vi "squash2016_2.vi"() -> ()   [LabVIEW 2014]
uses:
  <vilib>/vision/Image Controls.llb/IMAQ Image.ctl
  <vilib>/Utility/file.llb/Read From Spreadsheet File (string).vi
  <vilib>/Utility/file.llb/Read From Spreadsheet File (I64).vi
panel:
  in  "Upload edited video":bool
  in  "Extract data":bool
  in  "UNex win1":string="Unexpected \nwinner"
  in  "Expected Winner1 4":bool
  in  "Player 1 shots":string[](array[string])=["Att drive", "Def drive", "Att SW drive", "Def SW drive", "", "Drop", "Chop", "Lob", "Boast 2", "Boast 3", "Smash", "", "F-hand", "B-hand", "", "Straight", "Cross", "", "Bounce", "Volley", "H-volley"]
  in  "Player 1 shots 2":string[](array[string])=["Att drive", "Def drive", "Att SW drive", "Def SW drive", "", "Drop", "Chop", "Lob", "Boast 2", "Boast 3", "Smash", "", "F-hand", "B-hand", "", "Straight", "Cross", "", "Bounce", "Volley", "H-volley"]
  in  "Player2 2":bool
  in  "Player1 2":bool
  in  "FH":bool
  in  "BH":bool
  in  "ST":bool
  in  "CR":bool
  in  "Bounce":bool
  in  "Half Volley":bool
  in  "Volley":bool
  out "last saved data":i64[](array[numeric])
  out "Btn 10":string
  out "Btn 9":string
  out "Btn 8":string
  out "Btn 7":string
  out "Btn 6":string
  out "subarray":i64[](array[numeric])
  out "output array":i64[][](array[numeric])
  out "appended array":i64[](array[numeric])
  out "0, 1":i16[](array[numeric])
  in  "REPORT":bool
  out "Player 2 data":i64[](array[numeric])
  out "player 1 data":i64[](array[numeric])
  out "both player data":i64[](array[numeric])
  out "Edited data":i64[][](array[numeric])
  out "Event After":i64[][](array[numeric])
  out "Event before":i64[][](array[numeric])
  out "result":i32[](array[numeric])
  out "EVENTS\nTO PLAY":i32[](array[numeric])
  out "Combined data":i64[][](array[numeric])
  out "Extra":i16
  out "Score change":bool[](array[boolean])
  out "last row":i32[](array[numeric])
  out "Player 1/2":i16
  out "Service":i16
  out "Cross":i16
  out "Straight":i16
  out "position":i16
  out "Main tab 2":T1(ring)
  in  "fast rewind":bool
  out "refnum of data save file":refnum<file>
  in  "START":bool
  out "frames to write":i64[][](array[numeric])
  in  "Data file":path=path "C:/Users/KoKuM/Desktop/Current work/ISN/SQUASH/testdata/test2.xls" caption="Data"
  in  "playback speed":dbl(slide)=1.0 min=0.25 max=1.5 step=0.25 scale=0.25..1.5
  in  "Main tab":enum32{"Coding", "Display"}(tab)
  in  "Boast 10":bool
  in  "Boast 12":bool
  in  "Boast 9":bool
  in  "Boast 11":bool
  in  "Smash 12":bool
  in  "Smash 11":bool
  in  "Smash 10":bool
  in  "Smash 9":bool
  in  "lob 12":bool
  in  "Drop 12":bool
  in  "lob 11":bool
  in  "Drop 11":bool
  in  "lob 10":bool
  in  "Drop 10":bool
  in  "lob 9":bool
  in  "Drop 9":bool
  in  "Chop 12":bool
  in  "Chop 11":bool
  in  "Chop 10":bool
  in  "Chop 9":bool
  in  "Smash 8":bool
  in  "Smash 7":bool
  in  "Smash 6":bool
  in  "Smash 5":bool
  in  "Smash":bool
  in  "Smash 2":bool
  in  "Smash 3":bool
  in  "Smash 4":bool
  in  "Chop 8":bool
  in  "Chop 7":bool
  in  "Chop 6":bool
  in  "Chop 5":bool
  in  "Chop":bool
  in  "Chop 2":bool
  in  "Chop 3":bool
  in  "Chop 4":bool
  in  "Boast 7":bool
  in  "Boast 5":bool
  in  "Boast 3":bool
  in  "Boast":bool
  in  "lob 8":bool
  in  "Drop 8":bool
  in  "Boast 6":bool
  in  "lob 7":bool
  in  "Drop 7":bool
  in  "lob 6":bool
  in  "Drop 6":bool
  in  "Boast 8":bool
  in  "lob 5":bool
  in  "Drop 5":bool
  in  "lob 13":bool
  in  "Drop":bool
  in  "Boast 2":bool
  in  "lob 2":bool
  in  "Drop 2":bool
  in  "lob 3":bool
  in  "Drop 3":bool
  in  "Boast 4":bool
  in  "lob 4":bool
  in  "Drop 4":bool
  in  "Let":bool
  in  "Nolet1":bool
  in  "Nolet2":bool
  in  "Stroke1":bool
  in  "Stroke2":bool
  in  "Expected Winner1":bool
  in  "Expected Winner2":bool
  in  "Unexpected Winner1":bool
  in  "Unexpected Winner2":bool
  in  "Forced Error1":bool
  in  "Unforced Error1":bool
  in  "Forced Error2":bool
  in  "Unforced Error2":bool
  in  "Pause lag(s)":dbl=1.0 min=0.0 max=2.0 step=0.5 format="%#.1g"
  in  "Code lag(s)":dbl=1.0 min=0.0 max=5.0 step=0.5 format="%#.1g"
  in  "Link Errors":bool
  in  "Btn 1":string
  in  "Btn 2":string
  in  "Btn 3":string
  in  "Btn 4":string
  in  "Btn 5":string
  in  "Button 1":bool
  in  "Button 2":bool
  in  "Button 3":bool
  in  "Button 4":bool
  in  "Button 5":bool
  out "P2":i32
  out "P1":i32
  out "Player1/Player2":bool[](array[boolean])
  in  "S6":bool
  in  "S5":bool
  in  "S4":bool
  in  "S3":bool
  in  "S2":bool
  in  "Service1":bool
  in  "Service2":bool
  in  "S1":bool
  in  "Player2":bool
  in  "Player1":bool
  in  "Auto switch":bool
  in  "5 4":bool
  in  "5 3":bool
  in  "5 2":bool
  in  "5 1":bool
  in  "6 4":bool
  in  "6 3":bool
  in  "6 2":bool
  in  "6 1":bool
  in  "4 4":bool
  in  "4 3":bool
  in  "4 2":bool
  in  "4 1":bool
  in  "3 4":bool
  in  "3 3":bool
  in  "3 2":bool
  in  "3 1":bool
  in  "2 4":bool
  in  "2 3":bool
  in  "2 2":bool
  in  "2 1":bool
  in  "1 4":bool
  in  "1 3":bool
  in  "1 2":bool
  in  "1 1":bool
  in  "after 2":u8(slide)=2 scale=0.0..5.0
  in  "before 2":u8(slide)=2
  in  "Pause lag on":bool
  in  "SWDrive":bool
  in  "SWADrive 12":bool
  in  "SWADrive 11":bool
  in  "SWADrive 10":bool
  in  "SWADrive 9":bool
  in  "SWDDrive 12":bool
  in  "SWDDrive 11":bool
  in  "SWDDrive 10":bool
  in  "SWDDrive 9":bool
  in  "ADrive 12":bool
  in  "ADrive 11":bool
  in  "ADrive 10":bool
  in  "ADrive 9":bool
  in  "DDrive 12":bool
  in  "DDrive 11":bool
  in  "DDrive 10":bool
  in  "DDrive 9":bool
  in  "DDrive 8":bool
  in  "DDrive 7":bool
  in  "DDrive 6":bool
  in  "DDrive 5":bool
  in  "DDrive":bool
  in  "DDrive 2":bool
  in  "DDrive 3":bool
  in  "DDrive 4":bool
  in  "ADrive 8":bool
  in  "ADrive 7":bool
  in  "ADrive 6":bool
  in  "ADrive 5":bool
  in  "ADrive":bool
  in  "ADrive 2":bool
  in  "ADrive 3":bool
  in  "ADrive 4":bool
  in  "SWDDrive 8":bool
  in  "SWDDrive 7":bool
  in  "SWDDrive 6":bool
  in  "SWDDrive 5":bool
  in  "SWDDrive":bool
  in  "SWDDrive 2":bool
  in  "SWDDrive 3":bool
  in  "SWDDrive 4":bool
  in  "SWADrive 8":bool
  in  "SWADrive 7":bool
  in  "SWADrive 6":bool
  in  "SWADrive 5":bool
  in  "SWADrive":bool
  in  "SWADrive 2":bool
  in  "SWADrive 3":bool
  in  "SWADrive 4":bool
  in  "Drive":bool
  in  "Undo":bool
  in  "Display tab":enum32{"Edit ", "Data Display"}(tab)
  in  "1 10":bool
  in  "1 7":bool
  in  "1 6":bool
  in  "1 5":bool
  in  "2 10":bool
  in  "2 7":bool
  in  "2 6":bool
  in  "2 5":bool
  in  "3 9":bool
  in  "3 7":bool
  in  "3 6":bool
  in  "3 5":bool
  in  "4 9":bool
  in  "4 7":bool
  in  "4 6":bool
  in  "4 5":bool
  in  "before":u8(slide)=2
  in  "after":u8(slide)=2 scale=0.0..5.0
  in  "Combine":bool
  in  "S6 2":bool
  in  "S5 2":bool
  in  "S4 2":bool
  in  "S1 2":bool
  in  "Service2 2":bool
  in  "Service1 2":bool
  in  "S2 2":bool
  in  "S3 2":bool
  out "Video files to write":string[](array[string])
  in  "Video compress":bool=TRUE
  in  "Abort":bool
  in  "Write file":bool
  in  "Delete":bool[](array[boolean])
  out "Writing":u32(slide) scale=0.0..404.0
  in  "File name":string
  in  "Add to lib":bool
  in  "Video to write":path caption="Folder"
  in  "Examine code":bool
  in  "Update":bool
  in  "Reset":bool
  in  "Code number display":i32 min=1 max=4
  in  "Next":bool
  in  "Previous":bool
  in  "6 5":bool
  in  "6 6":bool
  in  "6 7":bool
  in  "6 8":bool
  in  "5 5":bool
  in  "5 6":bool
  in  "5 7":bool
  in  "5 8":bool
  in  "Button 7":bool
  in  "Button 8":bool
  in  "Button 9":bool
  in  "Button 10":bool
  in  "Button 6":bool
  in  "playback interval on":bool
  in  "Player 2 shots":string[](array[string])=["Att drive", "Def drive", "Att SW drive", "Def SW drive", "", "Drop", "Chop", "Lob", "Boast 2", "Boast 3", "Smash", "", "F-hand", "B-hand", "", "Straight", "Cross", "", "Bounce", "Volley", "H-volley"]
  out "FH 2":u8(slide) scale=0.0..2.0
  out "BH 2":u8(slide) scale=0.0..2.0
  out "Straight 2":u8(slide) scale=0.0..2.0
  out "Cross 2":u8(slide) scale=0.0..2.0
  out "Bounce 2":u8(slide) scale=0.0..2.0
  out "Volley 2":u8(slide) scale=0.0..2.0
  out "Drive 2":u8(slide) scale=0.0..2.0
  out "Lob 2":u8(slide) scale=0.0..2.0
  out "Drop 13":u8(slide) scale=0.0..2.0
  out "Boast 13":u8(slide) scale=0.0..2.0
  out "Player 2 shots numbers":string[](array[string])=["0", "0", "0", "0", "", " ", "0", "0", "", "0", "0", "", "0", "0"]
  in  "Fh 2":string="Forehand"
  in  "BH 4":string="Backhand"
  in  "Cross 6":string="Cross"
  in  "bounce 2":string="Bounce"
  in  "Straight 6":string="Straight"
  in  "volley 2":string="Volley"
  in  "H-volley 2":string="Half volley"
  out "F-hand 2":string="0"
  out "B-hand 2":string="0"
  out "Cross 3":string="0"
  out "Bounce 3":string="0"
  out "Straight 3":string="0"
  out "Volley 3":string="0"
  out "H-volley 3":string="0"
  out "4 42":dbl
  out "4 32":dbl
  out "4 22":dbl
  out "4 12":dbl
  out "3 42":dbl
  out "3 32":dbl
  out "3 22":dbl
  out "3 12":dbl
  out "2 42":dbl
  out "2 32":dbl
  out "2 22":dbl
  out "2 12":dbl
  out "1 42":dbl
  out "1 32":dbl
  out "1 22":dbl
  out "1 12":dbl
  in  "H-volley":string="Half volley"
  in  "volley":string="Volley"
  in  "Straight 5":string="Straight"
  in  "bounce":string="Bounce"
  in  "Cross 5":string="Cross"
  in  "BH 3":string="Backhand"
  in  "Fh":string="Forehand"
  out "1 14":dbl
  out "1 13":dbl
  out "1 11":dbl
  out "1 9":dbl
  out "2 14":dbl
  out "2 13":dbl
  out "2 11":dbl
  out "2 9":dbl
  out "3 13":dbl
  out "3 11":dbl
  out "3 10":dbl
  out "3 8":dbl
  out "4 13":dbl
  out "4 11":dbl
  out "4 10":dbl
  out "4 8":dbl
  out "H-volley 1":string="0"
  out "F-hand 1":string="0"
  out "B-hand 1":string="0"
  out "Cross 1":string="0"
  out "Bounce 1":string="0"
  out "Straight 1":string="0"
  out "Volley 1":string="0"
  out "FH 1":u8(slide) scale=0.0..2.0
  out "BH 1":u8(slide) scale=0.0..2.0
  out "Straight 4":u8(slide) scale=0.0..2.0
  out "Cross 4":u8(slide) scale=0.0..2.0
  out "Bounce 4":u8(slide) scale=0.0..2.0
  out "Volley 4":u8(slide) scale=0.0..2.0
  out "Drive 1":u8(slide) scale=0.0..2.0
  out "Lob 1":u8(slide) scale=0.0..2.0
  out "Drop 1":u8(slide) scale=0.0..2.0
  out "Boast 1":u8(slide) scale=0.0..2.0
  out "Player 1 shots numbers":string[](array[string])=["0", "0", "0", "0", "", " ", "0", "0", "", "0", "0", "", "0", "0"]
  in  "display\nselection":string(combo)="1"
  out "5 14":dbl
  out "5 23":dbl
  out "5 33":dbl
  out "5 43":dbl
  out "6 15":dbl
  out "6 24":dbl
  out "6 34":dbl
  out "6 44":dbl
  out "5 18":dbl
  out "5 15":dbl
  out "5 16":dbl
  out "5 17":dbl
  out "6 18":dbl
  out "6 19":dbl
  out "6 20":dbl
  out "6 21":dbl
  in  "Smash 13":bool
  in  "DSWdrive":bool
  in  "Lob":bool
  in  "ASWdrive":bool
  in  "Adrive":bool
  in  "Ddrive":bool
  in  "Chop 13":bool
  in  "Drop 14":bool
  in  "Boast2":bool
  in  "Boast3":bool
  in  "String":string="Def SW drive"
  out "No Let 2":string="0"
  out "Let 4":string="0"
  out "Stroke 4":string="0"
  out "ex win2 num":string="0"
  out "UNex win2 num":string="0"
  out "F err2 num":string="0"
  out "UF err2 num":string="0"
  in  "Let 5":bool
  in  "Nolet2 2":bool
  in  "Stroke2 2":bool
  in  "Unforced Error2 2":bool
  in  "Forced Error2 2":bool
  in  "Unexpected Winner2 2":bool
  in  "Expected Winner2 2":bool
  out "No Let 1":string="0"
  out "Let 3":string="0"
  out "Stroke 3":string="0"
  out "ex win1 num":string="0"
  out "UNex win1 num":string="0"
  out "F err1 num":string="0"
  out "UF err1 num":string="0"
  in  "Let 2":bool
  in  "Nolet1 2":bool
  in  "Stroke1 2":bool
  in  "Unforced Error1 2":bool
  in  "Forced Error1 2":bool
  in  "Unexpected Winner1 2":bool
  in  "Expected Winner1 2":bool
  in  "Load video":bool
  in  "Play":bool
  out "ful video frames":i64[](array[numeric])
  out "playback speed":dbl
  out "Number of Frames":u32
  out "framesPerSecond":u32
  out "Last Edit":bool[](array[boolean])
  out "frames 2 play":i64[](array[numeric])
  in  "stop":bool
  out "Video Frame":u32
  out "edited\nevents":i64[][](array[numeric])
  out "edited to play":i64[](array[numeric])
  out "frames edited":i64[](array[numeric])
  in  "fast forward":bool
  in  "Pause":bool
  out "coding":i64[][](array[numeric])
  in  "Progress...":u32(slide) min=400 max=47374 scale=-1.1..130372.0
  in  "Video file":path=path "C:/Users/KoKuM/Desktop/Current work/ISN/SQUASH/testdata/WWC16_FIN_w1.avi" caption="Video"
  out "task":i32(slide) scale=0.0..300.0
  out "Video":T2(plugin-control)
  # "Playback interval (s)"
  # "© 2016 National Sports Institute of Malaysia All Rights Reserved"
  # "Position"
  # "Drop"
  # "Chop"
  # "Lob"
  # "Boast"
  # "Smash"
  # "Att"
  # "Def"
  # "Att"
  # "Def"
  # "Half volley"
  # "Forehand"
  # "Backhand"
  # "St"
  # "Cr"
  # "St"
  # "Cr"
  # "Volley"
  # "Forehand"
  # "Backhand"
  # "St"
  # "Cr"
  # "St"
  # "Cr"
  # "Bounce"
  # "Forehand"
  # "Backhand"
  # "St"
  # "Cr"
  # "St"
  # "Cr"
  # "Lead and lag settings"
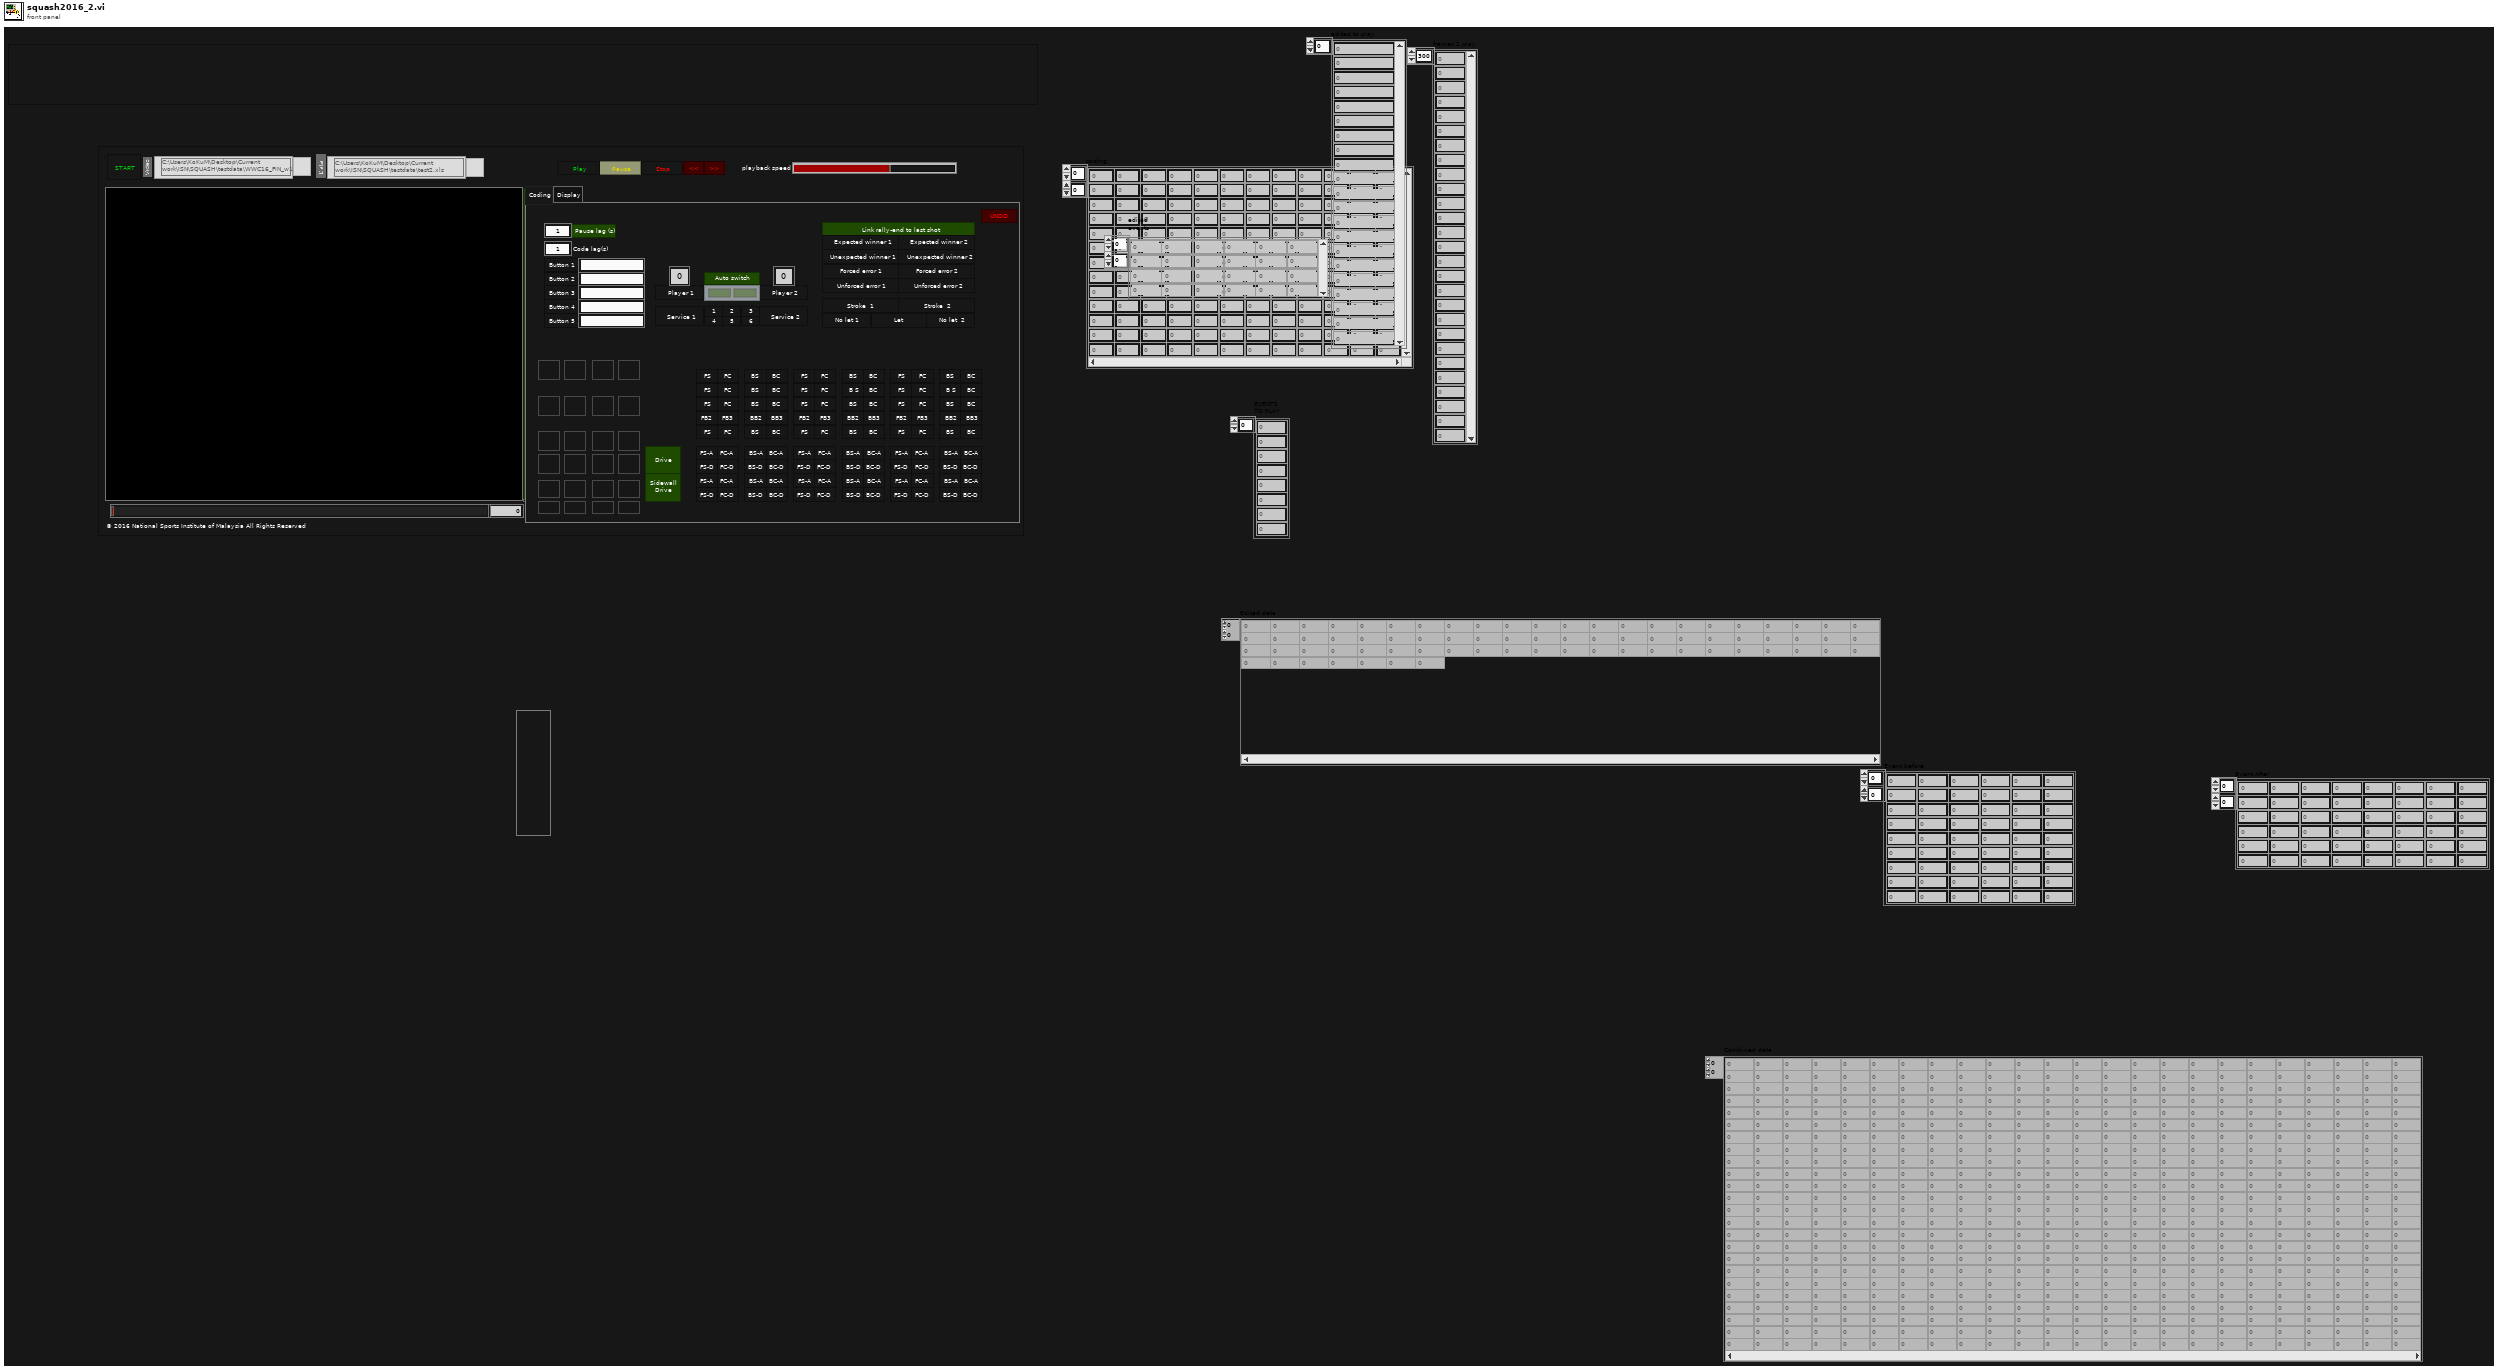
[diagram p1: front panel]
types:
  T1 = enum32{"Coding", "Edit video", "Examine coding", "Display", "Update coding", "Edit coding"}
  T2 = typedef "IMAQ Image.ctl" = refnum<image>
  T3 = enum16{"open", "replace", "create", "open or create", "replace or create", "replace or create with confirmation"}
  T4 = enum8{"Enabled", "Disabled", "Disabled and Grayed Out"}
  T5 = typedef "Image Type" = u32
  T6 = typedef "AviRefnum.ctl" = refnum<k1>
  T7 = cluster{"width":u32, "height":u32, "framesPerSecond":u32, "compressionFilter":string, "hasData":bool}
  T8 = typedef "eventvkey.ctl" = enum16{"ASCII", "Enter", "Return", "Shift", "Ctrl", "Alt", "Cmd", "Opt", "Caps", "NumLock", "Clear", "Break", "Up", "Down", "Left", "Right", "Insert", "Delete", "Home", "End", "PageUp", "PageDown", "Escape", "Help", "Pause", "ScrollLock", "F1", "F2", "F3", "F4", "F5", "F6", "F7", "F8", "F9", "F10", "F11", "F12", "F13", "F14", "F15", "F16", "F17", "F18", "F19", "F20", "F21", "F22", "F23", "F24", "Play", "VolumeUp", "VolumeDown", "Mute", "Two Byte Char"}
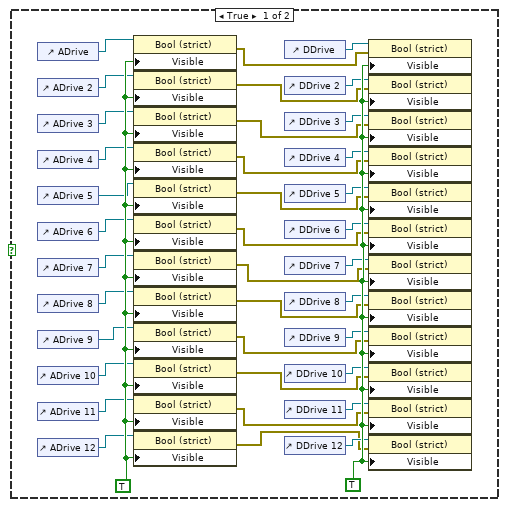
[diagram p2: hidden frame]
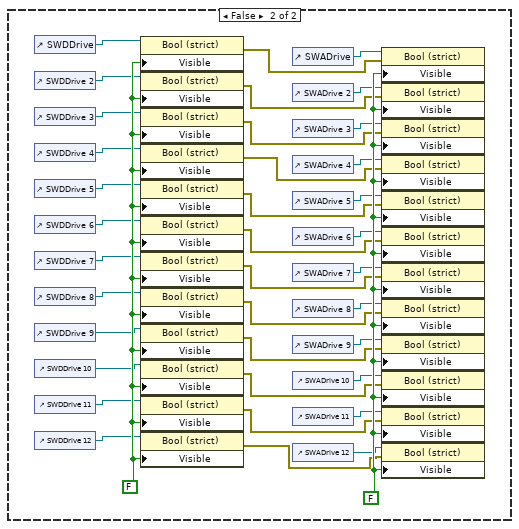
[diagram p3: hidden frame]
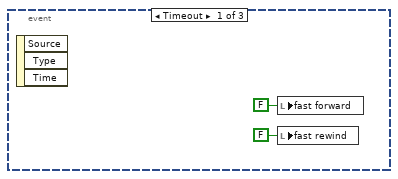
[diagram p4: hidden frame]
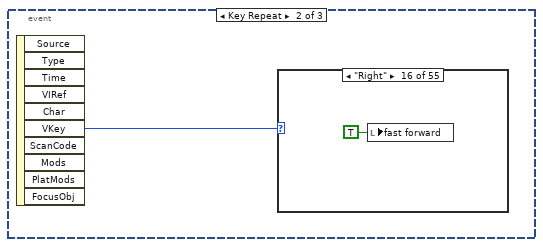
[diagram p5: hidden frame]
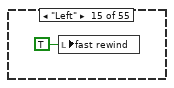
[diagram p20: hidden frame]
diagram:
  n1 = while {
    stop <- FALSE stop-if-true
    n2 = flat-sequence {
      tunnel: [w42] -> w15
      tunnel: [w43] -> w16
      tunnel: w16 -> [w136]
      tunnel: w15 -> [w135]
      tunnel: [w135] -> w14
      tunnel: [w136] -> w13
      tunnel: w14 -> [w176]
      tunnel: w13 -> [w159]
      tunnel: [w175] -> w11
      tunnel: [w158] -> w10
      tunnel: [w157] -> w9
      tunnel: [w156] -> w1
      tunnel: [w155] -> w8
      frame #0 {
        w37 = T4."Enabled" ("Disabled")
        w39 = u32 0 ("Progress...")
        w36 = FALSE ("START")
        w35 = T4."Disabled and Grayed Out" ("Disabled")
        n3 = property on="Play" class="Bool (strict)"("DisabledEnum"=w35, "Value"=w36) -> ()  [unwired: 2 in, 2 out]
        n4 = property on="stop" class="Bool (strict)"("DisabledEnum"=w35, "Value"=w36) -> ()  [unwired: 2 in, 2 out]
        n5 = property on="Pause" class="Bool (strict)"("DisabledEnum"=w35, "Value"=w36) -> ()  [unwired: 2 in, 2 out]
        n6 = property on="fast forward" class="Bool (strict)"("DisabledEnum"=w35, "Value"=w36) -> ()  [unwired: 2 in, 2 out]
        n7 = property on="playback speed" class="Slide (strict)"("DisabledEnum"=w35, "Value"=1.0 ("playback speed")) -> ()  [unwired: 2 in, 2 out]
        n8 = property on="Main tab" class="TabCtl (strict)"("DisabledEnum"=w35, "Value"=enum32{"Coding", "Display"}."Coding" ("Main tab")) -> ()  [unwired: 2 in, 2 out]
        n9 = property on="Progress..." class="Slide (strict)"("DisabledEnum"=w35, "Value"=w39) -> ()  [unwired: 2 in, 2 out]
        n10 = property on="Video Frame" class="DigNum (strict)"("DisabledEnum"=w35, "Value"=w39) -> ()  [unwired: 2 in, 2 out]
        n11 = property on="Video" class="ImageControl"("DisabledEnum"=w35, "Value"=T2 refnum ("Video")) -> ()  [unwired: 2 in, 2 out]
        n12 = property on="START" class="Bool (strict)"("DisabledEnum"=w37, "Value"=w36) -> ()  [unwired: 2 in, 2 out]
        n13 = property on="Video file" class="Path"("DisabledEnum"=w37) -> ()  [unwired: 2 in, 2 out]
        n14 = property on="Data file" class="Path"("DisabledEnum"=w37) -> ()  [unwired: 2 in, 2 out]
        n15 = property on="fast rewind" class="Bool (strict)"("DisabledEnum"=w35, "Value"=w36) -> ()  [unwired: 2 in, 2 out]
      }
      frame #1 {
        n16 = while {
          tunnel: [w45] -> w43
          tunnel: [w44] -> w42
          stop <- w46 stop-if-true
          n17 = case shown="True" "START" {
            tunnel: [FALSE w51] -> w46
            tunnel: [w48 w54] -> w45
            tunnel: [w48 w53] -> w44
            frame False {
              w48 = path "" ("dup path")
              n18 = Wait (ms)(milliseconds to wait=u32 200) -> ()  [unwired: 1 out]
            }
            frame True {
              n19 = Path To String(path="Data file") -> (string=w63:string)
              n20 = Wait (ms)(milliseconds to wait=u32 200) -> ()  [unwired: 1 out]
              n21 = Empty String/Path?(string/path=w63) -> (empty?=w62:bool)
              n22 = case shown="False" w62 {
                tunnel: "Data file" -> [w84 w109]
                tunnel: [w83 FALSE] -> w60
                tunnel: [w82 w109] -> w53
                frame False {
                  n23 = Strip Path(path=w84) -> (stripped path=w89:path)  [unwired: 1 out]
                  n24 = Path To String(path=w89) -> (string=w88:string)
                  n25 = call <vilib>:"Get File Extension.vi"("file"=w84) -> ("filename without extension"=w91:string)  [unwired: 7 in, 3 out]
                  n26 = Concatenate Strings(w88, "\\" ("string"), w91, ".xls" ("string")) -> (w90:string)
                  n27 = String To Path(string=w90) -> (path=w85:path)
                  n28 = call <vilib>:"Check if File or Folder Exists.vi"("path"=w85) -> ("file or folder exists?"=w86:bool)  [unwired: 8 in, 2 out]
                  n29 = case shown="True" w86 {
                    selector: w86 -> [_ w108]
                    tunnel: w85 -> [w95 w107]
                    tunnel: [w94 w108] -> w83
                    tunnel: [w93 w107] -> w82
                    frame False {
                      n30 = Two Button Dialog(message="This data file does not exist.\nDo you wish to start a new project?", 1:"No" ("F button name (\"Cancel\")"), 2:"Yes" ("T button name (\"OK\")")) -> (T button?=w96:bool)
                      n31 = case shown="False" w96 {
                        selector: w96 -> [w101 w103]
                        tunnel: w95 -> [_ w102]
                        tunnel: [w101 w103] -> w94
                        tunnel: [path "" ("dup path") w102] -> w93
                        frame False {
                        }
                        frame True {
                          n32 = Open/Create/Replace File(file path (use dialog)=w102, operation (0:open)=T3."create") -> (refnum out=w104:refnum<file>, error out=w106:errorcluster)  [unwired: 4 in, 1 out]
                          n33 = Close File(refnum=w104, error in=w106) -> ()  [unwired: 2 out]
                        }
                      }
                    }
                    frame True {
                    }
                  }
                }
                frame True {
                  n34 = One Button Dialog(message="Please enter data file") -> ()  [unwired: 1 in, 1 out]
                }
              }
              n35 = Path To String(path="Video file") -> (string=w58:string)
              n36 = Empty String/Path?(string/path=w58) -> (empty?=w57:bool)
              n37 = case shown="True" w57 {
                selector: w57 -> [_ w81]
                tunnel: "Video file" -> [w68 w79]
                tunnel: [w65 w79] -> w54
                tunnel: [w64 w81] -> w55
                frame False {
                  n38 = call <vilib>:"Check if File or Folder Exists.vi"("path"=w68) -> ("file or folder exists?"=w72:bool, "dup path"=w66:path)  [unwired: 8 in, 1 out]
                  n39 = call <vilib>:"Get File Extension.vi"("file"=w68) -> ("lowercase file extension"=w69:string)  [unwired: 7 in, 3 out]
                  n40 = Not(x=w72) -> (.not. x?=w73:bool)
                  n41 = Not Equal?(x=w69, y="avi" ("lowercase file extension")) -> (x != y?=w71:bool)
                  n42 = Or(x=w73, y=w71) -> (x .or. y?=w67:bool)
                  n43 = case shown="True" w67 {
                    selector: w67 -> [w74 w76]
                    tunnel: w66 -> [w75 _]
                    tunnel: [w75 path "" ("dup path")] -> w65
                    tunnel: [w74 w76] -> w64
                    frame False {
                    }
                    frame True {
                      n44 = One Button Dialog(message="You have chosen an invalid video file for coding\n\nPossible reasons\n1)\tChosen video file format was not AVI\n2)\tChosen video file does not exist") -> ()  [unwired: 1 in, 1 out]
                    }
                  }
                }
                frame True {
                  n45 = One Button Dialog(message="Please enter video file") -> ()  [unwired: 1 in, 1 out]
                }
              }
              n46 = Not(x=w55) -> (.not. x?=w59:bool)
              n47 = local write "Video file"(w54) -> ()
              n48 = And(x=w59, y=w60) -> (x .and. y?=w51:bool)
              n49 = local write "Data file"(w53) -> ()
              n50 = local write "START"(w51) -> ()
            }
          }
        }
      }
      frame #2 {
        w115 = FALSE ("Combine")
        w114 = i64[] [] ("to write")
        w131 = 0 ("P1")
        w112 = FALSE ("4 6")
        w116 = TRUE ("4 6")
        w151 = FALSE ("4 6")
        w149 = TRUE ("Extract data")
        w117 = u8 2 ("before")
        w134 = T4."Disabled and Grayed Out" ("Disabled")
        w154 = u32 0 ("Progress...")
        w137 = FALSE ("START")
        w138 = T4."Enabled" ("Disabled")
        n51 = property on="Play" class="Bool (strict)"("DisabledEnum"=w138, "Value"=w137) -> ()  [unwired: 2 in, 2 out]
        n52 = property on="stop" class="Bool (strict)"("DisabledEnum"=w138, "Value"=w137) -> ()  [unwired: 2 in, 2 out]
        n53 = property on="Pause" class="Bool (strict)"("DisabledEnum"=w138, "Value"=w137) -> ()  [unwired: 2 in, 2 out]
        n54 = property on="fast forward" class="Bool (strict)"("DisabledEnum"=w138, "Value"=w137) -> ()  [unwired: 2 in, 2 out]
        n55 = property on="fast rewind" class="Bool (strict)"("DisabledEnum"=w138, "Value"=w137) -> ()  [unwired: 2 in, 2 out]
        n56 = property on="playback speed" class="Slide (strict)"("DisabledEnum"=w138, "Value"=1.0 ("playback speed")) -> ()  [unwired: 2 in, 2 out]
        n57 = property on="Main tab" class="TabCtl (strict)"("DisabledEnum"=w138, "Value"=enum32{"Coding", "Display"}."Coding" ("Main tab")) -> ()  [unwired: 2 in, 2 out]
        n58 = property on="Progress..." class="Slide (strict)"("DisabledEnum"=w138, "Value"=w154) -> ()  [unwired: 2 in, 2 out]
        n59 = property on="Video Frame" class="DigNum (strict)"("DisabledEnum"=w138, "Value"=w154) -> ()  [unwired: 2 in, 2 out]
        n60 = property on="Video" class="ImageControl"("DisabledEnum"=w138) -> ()  [unwired: 2 in, 2 out]
        n61 = property on="Video file" class="Path"("DisabledEnum"=w134) -> ()  [unwired: 2 in, 2 out]
        n62 = property on="Data file" class="Path"("DisabledEnum"=w134) -> ()  [unwired: 2 in, 2 out]
        n63 = property on="Code number display" class="DigNum (strict)"("DisabledEnum"=w134) -> ()  [unwired: 2 in, 2 out]
        n64 = property on="Next" class="Bool (strict)"("DisabledEnum"=w134) -> ()  [unwired: 2 in, 2 out]
        n65 = property on="Reset" class="Bool (strict)"("DisabledEnum"=w134) -> ()  [unwired: 2 in, 2 out]
        n66 = property on="Update" class="Bool (strict)"("DisabledEnum"=w134) -> ()  [unwired: 2 in, 2 out]
        n67 = property on="Previous" class="Bool (strict)"("DisabledEnum"=w134) -> ()  [unwired: 2 in, 2 out]
        n68 = local write "Pause lag(s)"(1.0 ("Pause lag(s)")) -> ()
        n69 = local write "Code lag(s)"(0.5 ("Code lag(s)")) -> ()
        n70 = local write "Link Errors"(TRUE ("Link Errors")) -> ()
        n71 = local write "Pause lag on"(w116) -> ()
        n72 = local write "SWDrive"(w116) -> ()
        n73 = local write "Drive"(w116) -> ()
        n74 = local write "playback interval on"(w116) -> ()
        n75 = local write "Auto switch"(w116) -> ()
        n76 = local write "Combine"(w115) -> ()
        n77 = local write "Button 10"(w115) -> ()
        n78 = local write "Undo"(w115) -> ()
        n79 = local write "Button 8"(w115) -> ()
        n80 = local write "Button 9"(w115) -> ()
        n81 = local write "Button 6"(w115) -> ()
        n82 = local write "Button 7"(w115) -> ()
        n83 = local write "Last Edit"(bool[] [FALSE, FALSE, FALSE, FALSE, FALSE, FALSE, FALSE, FALSE, FALSE, FALSE, FALSE, FALSE, FALSE, FALSE, FALSE, FALSE, FALSE, FALSE, FALSE, FALSE, FALSE, FALSE, FALSE, FALSE, FALSE, FALSE, FALSE, FALSE, FALSE, FALSE, FALSE, FALSE, FALSE, FALSE, FALSE, FALSE] ("Last Edit")) -> ()
        n84 = local write "File name"("" ("File name")) -> ()
        n85 = local write "Code number display"(1 ("Code number display")) -> ()
        n86 = local write "Delete"(bool[] [TRUE, TRUE, TRUE, TRUE, TRUE] ("Array 2")) -> ()
        n87 = local write "Video compress"(w149) -> ()
        n88 = local write "Extract data"(w149) -> ()
        n89 = local write "Upload edited video"(w151) -> ()
        n90 = local write "Add to lib"(w151) -> ()
        n91 = local write "Abort"(w151) -> ()
        n92 = local write "Write file"(w151) -> ()
        n93 = local write "REPORT"(w151) -> ()
        n94 = local write "Examine code"(w151) -> ()
        n95 = local write "Update"(w151) -> ()
        n96 = local write "Reset"(w151) -> ()
        n97 = local write "Previous"(w151) -> ()
        n98 = local write "Next"(w151) -> ()
        n99 = local write "before"(w117) -> ()
        n100 = local write "after"(w117) -> ()
        n101 = local write "before 2"(w117) -> ()
        n102 = local write "after 2"(w117) -> ()
        n103 = call-poly <vilib>:"Read From Spreadsheet File.vi"("file path (dialog if empty)"=w135) -> ("all rows"=w123:string[][])  [unwired: 6 in, 4 out]
        n104 = Index Array(array=w123, index (row)=3) -> (element=w125:string[])  [unwired: 1 in]
        n105 = Index Array(array=w125, index #1=71 ("index"), index #2=72 ("index"), index #3=73 ("index"), index #4=74 ("index"), index #5=75 ("index")) -> (element #1=w120:string, element #2=w121:string, element #3=w122:string, element #4=w119:string, element #5=w118:string)
        n106 = local write "display\nselection"("1" ("display\nselection")) -> ()
        n107 = local write "task"(300 ("task")) -> ()
        n108 = local write "Load video"(FALSE ("Pause")) -> ()
        n109 = local write "Video files to write"(string[] [] ("Video files to write")) -> ()
        n110 = local write "frames to write"(i64[][] [] ("to write")) -> ()
        n111 = local write "player 1 data"(w114) -> ()
        n112 = local write "both player data"(w114) -> ()
        n113 = local write "Player 2 data"(w114) -> ()
        n114 = local write "last saved data"(w114) -> ()
        n115 = local write "Btn 1"(w120) -> ()
        n116 = local write "Btn 2"(w121) -> ()
        n117 = local write "Btn 3"(w122) -> ()
        n118 = local write "Btn 4"(w119) -> ()
        n119 = local write "Btn 5"(w118) -> ()
        n120 = local write "P1"(w131) -> ()
        n121 = local write "P2"(w131) -> ()
        n122 = local write "Drop"(w112) -> ()
        n123 = local write "Drop 2"(w112) -> ()
        n124 = local write "Drop 3"(w112) -> ()
        n125 = local write "Drop 4"(w112) -> ()
        n126 = local write "Drop 5"(w112) -> ()
        n127 = local write "Drop 6"(w112) -> ()
        n128 = local write "Drop 7"(w112) -> ()
        n129 = local write "Drop 8"(w112) -> ()
        n130 = local write "Drop 9"(w112) -> ()
        n131 = local write "Drop 10"(w112) -> ()
        n132 = local write "Drop 11"(w112) -> ()
        n133 = local write "Drop 12"(w112) -> ()
        n134 = local write "Chop"(w112) -> ()
        n135 = local write "Chop 2"(w112) -> ()
        n136 = local write "Chop 3"(w112) -> ()
        n137 = local write "Chop 4"(w112) -> ()
        n138 = local write "Chop 5"(w112) -> ()
        n139 = local write "Chop 6"(w112) -> ()
        n140 = local write "Chop 7"(w112) -> ()
        n141 = local write "Chop 8"(w112) -> ()
        n142 = local write "Chop 9"(w112) -> ()
        n143 = local write "Chop 10"(w112) -> ()
        n144 = local write "Chop 11"(w112) -> ()
        n145 = local write "Chop 12"(w112) -> ()
        n146 = local write "Player2 2"(w112) -> ()
        n147 = local write "Player1 2"(w112) -> ()
        n148 = local write "Button 7"(w112) -> ()
        n149 = local write "Button 8"(w112) -> ()
        n150 = local write "Button 9"(w112) -> ()
        n151 = local write "Button 10"(w112) -> ()
        n152 = local write "Button 6"(w112) -> ()
        n153 = local write "S6 2"(w112) -> ()
        n154 = local write "S5 2"(w112) -> ()
        n155 = local write "S4 2"(w112) -> ()
        n156 = local write "S1 2"(w112) -> ()
        n157 = local write "Service2 2"(w112) -> ()
        n158 = local write "Service1 2"(w112) -> ()
        n159 = local write "S2 2"(w112) -> ()
        n160 = local write "S3 2"(w112) -> ()
        n161 = local write "lob 13"(w112) -> ()
        n162 = local write "lob 2"(w112) -> ()
        n163 = local write "lob 3"(w112) -> ()
        n164 = local write "lob 4"(w112) -> ()
        n165 = local write "lob 5"(w112) -> ()
        n166 = local write "lob 6"(w112) -> ()
        n167 = local write "lob 7"(w112) -> ()
        n168 = local write "lob 8"(w112) -> ()
        n169 = local write "lob 9"(w112) -> ()
        n170 = local write "lob 10"(w112) -> ()
        n171 = local write "lob 11"(w112) -> ()
        n172 = local write "lob 12"(w112) -> ()
        n173 = local write "Smash"(w112) -> ()
        n174 = local write "Smash 2"(w112) -> ()
        n175 = local write "Smash 3"(w112) -> ()
        n176 = local write "Smash 4"(w112) -> ()
        n177 = local write "Smash 5"(w112) -> ()
        n178 = local write "Smash 6"(w112) -> ()
        n179 = local write "Smash 7"(w112) -> ()
        n180 = local write "Smash 8"(w112) -> ()
        n181 = local write "Smash 9"(w112) -> ()
        n182 = local write "Smash 10"(w112) -> ()
        n183 = local write "Smash 11"(w112) -> ()
        n184 = local write "Smash 12"(w112) -> ()
        n185 = local write "4 5"(w112) -> ()
        n186 = local write "4 6"(w112) -> ()
        n187 = local write "4 7"(w112) -> ()
        n188 = local write "4 9"(w112) -> ()
        n189 = local write "3 5"(w112) -> ()
        n190 = local write "3 6"(w112) -> ()
        n191 = local write "3 7"(w112) -> ()
        n192 = local write "3 9"(w112) -> ()
        n193 = local write "2 5"(w112) -> ()
        n194 = local write "2 6"(w112) -> ()
        n195 = local write "2 7"(w112) -> ()
        n196 = local write "2 10"(w112) -> ()
        n197 = local write "1 5"(w112) -> ()
        n198 = local write "1 6"(w112) -> ()
        n199 = local write "1 7"(w112) -> ()
        n200 = local write "1 10"(w112) -> ()
        n201 = local write "6 5"(w112) -> ()
        n202 = local write "6 6"(w112) -> ()
        n203 = local write "6 7"(w112) -> ()
        n204 = local write "6 8"(w112) -> ()
        n205 = local write "5 5"(w112) -> ()
        n206 = local write "5 6"(w112) -> ()
        n207 = local write "5 7"(w112) -> ()
        n208 = local write "5 8"(w112) -> ()
        n209 = local write "Half Volley"(w112) -> ()
        n210 = local write "ADrive"(w112) -> ()
        n211 = local write "ADrive 2"(w112) -> ()
        n212 = local write "ADrive 3"(w112) -> ()
        n213 = local write "ADrive 4"(w112) -> ()
        n214 = local write "ADrive 5"(w112) -> ()
        n215 = local write "ADrive 6"(w112) -> ()
        n216 = local write "ADrive 7"(w112) -> ()
        n217 = local write "ADrive 8"(w112) -> ()
        n218 = local write "ADrive 9"(w112) -> ()
        n219 = local write "ADrive 10"(w112) -> ()
        n220 = local write "ADrive 11"(w112) -> ()
        n221 = local write "ADrive 12"(w112) -> ()
        n222 = local write "DDrive"(w112) -> ()
        n223 = local write "DDrive 2"(w112) -> ()
        n224 = local write "DDrive 3"(w112) -> ()
        n225 = local write "DDrive 4"(w112) -> ()
        n226 = local write "DDrive 5"(w112) -> ()
        n227 = local write "DDrive 6"(w112) -> ()
        n228 = local write "DDrive 7"(w112) -> ()
        n229 = local write "DDrive 8"(w112) -> ()
        n230 = local write "DDrive 9"(w112) -> ()
        n231 = local write "DDrive 10"(w112) -> ()
        n232 = local write "DDrive 11"(w112) -> ()
        n233 = local write "DDrive 12"(w112) -> ()
        n234 = local write "Smash 13"(w112) -> ()
        n235 = local write "Boast3"(w112) -> ()
        n236 = local write "DSWdrive"(w112) -> ()
        n237 = local write "Lob"(w112) -> ()
        n238 = local write "ASWdrive"(w112) -> ()
        n239 = local write "Adrive"(w112) -> ()
        n240 = local write "Ddrive"(w112) -> ()
        n241 = local write "Chop 13"(w112) -> ()
        n242 = local write "Drop 14"(w112) -> ()
        n243 = local write "Boast2"(w112) -> ()
        n244 = local write "FH"(w112) -> ()
        n245 = local write "BH"(w112) -> ()
        n246 = local write "ST"(w112) -> ()
        n247 = local write "CR"(w112) -> ()
        n248 = local write "Bounce"(w112) -> ()
        n249 = local write "Volley"(w112) -> ()
        n250 = local write "SWADrive"(w112) -> ()
        n251 = local write "SWADrive 2"(w112) -> ()
        n252 = local write "SWADrive 3"(w112) -> ()
        n253 = local write "SWADrive 4"(w112) -> ()
        n254 = local write "SWADrive 5"(w112) -> ()
        n255 = local write "SWADrive 6"(w112) -> ()
        n256 = local write "SWADrive 7"(w112) -> ()
        n257 = local write "SWADrive 8"(w112) -> ()
        n258 = local write "SWADrive 9"(w112) -> ()
        n259 = local write "SWADrive 10"(w112) -> ()
        n260 = local write "SWADrive 11"(w112) -> ()
        n261 = local write "SWADrive 12"(w112) -> ()
        n262 = local write "SWDDrive"(w112) -> ()
        n263 = local write "SWDDrive 2"(w112) -> ()
        n264 = local write "SWDDrive 3"(w112) -> ()
        n265 = local write "SWDDrive 4"(w112) -> ()
        n266 = local write "SWDDrive 5"(w112) -> ()
        n267 = local write "SWDDrive 6"(w112) -> ()
        n268 = local write "SWDDrive 7"(w112) -> ()
        n269 = local write "SWDDrive 8"(w112) -> ()
        n270 = local write "SWDDrive 9"(w112) -> ()
        n271 = local write "SWDDrive 10"(w112) -> ()
        n272 = local write "SWDDrive 11"(w112) -> ()
        n273 = local write "SWDDrive 12"(w112) -> ()
        n274 = local write "Let 2"(w112) -> ()
        n275 = local write "Nolet2 2"(w112) -> ()
        n276 = local write "Nolet1 2"(w112) -> ()
        n277 = local write "Stroke2 2"(w112) -> ()
        n278 = local write "Stroke1 2"(w112) -> ()
        n279 = local write "Unforced Error2 2"(w112) -> ()
        n280 = local write "Forced Error2 2"(w112) -> ()
        n281 = local write "Unforced Error1 2"(w112) -> ()
        n282 = local write "Forced Error1 2"(w112) -> ()
        n283 = local write "Unexpected Winner2 2"(w112) -> ()
        n284 = local write "Unexpected Winner1 2"(w112) -> ()
        n285 = local write "Expected Winner2 2"(w112) -> ()
        n286 = local write "Expected Winner1 2"(w112) -> ()
        n287 = local write "Let 5"(w112) -> ()
        n288 = local write "Boast"(w112) -> ()
        n289 = local write "Boast 2"(w112) -> ()
        n290 = local write "Boast 3"(w112) -> ()
        n291 = local write "Boast 4"(w112) -> ()
        n292 = local write "Boast 5"(w112) -> ()
        n293 = local write "Boast 6"(w112) -> ()
        n294 = local write "Boast 7"(w112) -> ()
        n295 = local write "Boast 8"(w112) -> ()
        n296 = local write "Boast 9"(w112) -> ()
        n297 = local write "Boast 10"(w112) -> ()
        n298 = local write "Boast 11"(w112) -> ()
        n299 = local write "Boast 12"(w112) -> ()
        n300 = local write "4 4"(w112) -> ()
        n301 = local write "4 3"(w112) -> ()
        n302 = local write "4 2"(w112) -> ()
        n303 = local write "4 1"(w112) -> ()
        n304 = local write "3 4"(w112) -> ()
        n305 = local write "3 3"(w112) -> ()
        n306 = local write "3 2"(w112) -> ()
        n307 = local write "3 1"(w112) -> ()
        n308 = local write "2 4"(w112) -> ()
        n309 = local write "2 3"(w112) -> ()
        n310 = local write "2 2"(w112) -> ()
        n311 = local write "2 1"(w112) -> ()
        n312 = local write "1 4"(w112) -> ()
        n313 = local write "1 3"(w112) -> ()
        n314 = local write "1 2"(w112) -> ()
        n315 = local write "1 1"(w112) -> ()
        n316 = local write "5 4"(w112) -> ()
        n317 = local write "5 3"(w112) -> ()
        n318 = local write "5 2"(w112) -> ()
        n319 = local write "5 1"(w112) -> ()
        n320 = local write "6 4"(w112) -> ()
        n321 = local write "6 3"(w112) -> ()
        n322 = local write "6 2"(w112) -> ()
        n323 = local write "6 1"(w112) -> ()
        n324 = local write "S6"(w112) -> ()
        n325 = local write "S5"(w112) -> ()
        n326 = local write "S4"(w112) -> ()
        n327 = local write "S1"(w112) -> ()
        n328 = local write "S2"(w112) -> ()
        n329 = local write "S3"(w112) -> ()
        n330 = local write "Let"(w112) -> ()
        n331 = local write "Unexpected Winner2"(w112) -> ()
        n332 = local write "Unexpected Winner1"(w112) -> ()
        n333 = local write "Expected Winner2"(w112) -> ()
        n334 = local write "Expected Winner1"(w112) -> ()
        n335 = local write "Forced Error2"(w112) -> ()
        n336 = local write "Forced Error1"(w112) -> ()
        n337 = local write "Service2"(w112) -> ()
        n338 = local write "Service1"(w112) -> ()
        n339 = local write "Nolet2"(w112) -> ()
        n340 = local write "Nolet1"(w112) -> ()
        n341 = local write "Stroke2"(w112) -> ()
        n342 = local write "Stroke1"(w112) -> ()
        n343 = local write "Unforced Error2"(w112) -> ()
        n344 = local write "Unforced Error1"(w112) -> ()
        n345 = local write "Button 5"(w112) -> ()
        n346 = local write "Button 4"(w112) -> ()
        n347 = local write "Button 3"(w112) -> ()
        n348 = local write "Button 2"(w112) -> ()
        n349 = local write "Button 1"(w112) -> ()
        "Score change" <- bool[] [FALSE, FALSE] ("Score change")
        "Player1/Player2" <- bool[] [TRUE, FALSE] ("Score change")
      }
      frame #3 {
        w161 = T5 4 items=["Grayscale (U8)", "Grayscale (I16)", "Grayscale (SGL)", "Complex (CSG)", "RGB (U32)", "HSL (U32)", "RGB (U64)"] ("Image Type")
        n350 = Path to Array of Strings(0:w159) -> (2:w172:string[])  [unwired: 1 out]
        n351 = call "IMAQ AVI Open"("AVI Path"=w159) -> ("error out"=w163:errorcluster, "Avi Refnum"=w162:T6)  [unwired: 9 in]
        n352 = Delete From Array(array=w172) -> (array with subset deleted=w173:string[])  [unwired: 2 in, 1 out]
        n353 = call "IMAQ AVI Get Info"("error in (no error)"=w163, "Avi Refnum"=w162) -> ("error out"=w165:errorcluster, "Number of Frames"=w168:u32, "Avi Refnum (duplicate)"=w158:T6, "Frame Data"=w164:T7)  [unwired: 5 in, 1 out]
        "Number of Frames" <- w168
        n354 = Array of Strings to Path(0:w173) -> (2:w174:path)  [unwired: 1 in]
        n355 = call-poly <vilib>:"Read From Spreadsheet File.vi"("file path (dialog if empty)"=w176) -> ("all rows"=w179:i64[][])  [unwired: 6 in, 4 out]
        n356 = Decrement(x=w168) -> (x-1=w171:u32)
        n357 = local write "Video to write"(w174) -> ()
        n358 = Subtract(x=w171, y=200.0) -> (x-y=w169:dbl)
        n359 = Unbundle By Name(w164) -> ("framesPerSecond"=→"framesPerSecond":u32)
        n360 = property on="Progress..." class="Slide (strict)"(error in=w165, "Scale.Maximum"=w171) -> (error out=w166:errorcluster)  [unwired: 1 in, 1 out]
        n361 = Delete From Array(array=w179, length=4, index (row)=0) -> (array with subset deleted=w175:i64[][])  [unwired: 1 in, 1 out]
        n362 = for {
          N: w169 -> [_]
          tunnel: [w183] -> w155 mode=indexing
          i -> [w183]
        }
        "ful video frames" <- w155
        n363 = Index Array(array=w175, index (col)=0 ("disabled index (col)")) -> (element=w181:i64[])  [unwired: 1 in]
        n364 = Array Max & Min(array=w181) -> (max value=w180:i64)  [unwired: 3 out]
        n365 = call "IMAQ Create"("Image Name"="Video", "Image Type"=w161, "error in (no error)"=w166) -> ("New Image"=w157:T2, "error out"=w156:errorcluster)  [unwired: 2 in]
        n366 = local write "Progress..."(w180) -> ()
      }
    }
    n367 = while {
      tunnel: w10 -> [w355]
      tunnel: w9 -> [w354]
      tunnel: w1 -> [w353]
      shift-right: [w347] -> _
      shift-left: w8 -> [w346]
      tunnel: [w330] -> w4
      stop <- w331 continue-if-true
      # "This loop is the video play loop"
      # "1000/playback speed    / frames per sec"
      n368 = while {
        stop <- w371 continue-if-true
        n369 = local read "START"() -> (w370:bool)
        n370 = And(x=w370, y="Pause") -> (x .and. y?=w371:bool)
      }
      n371 = Index Array(array=w346, index="Progress...") -> (element=w333:i64)
      n372 = Array Max & Min(array=w346) -> (max value=w351:i64, max index (indices)=w352:i32)  [unwired: 2 out]
      n373 = while {
        stop <- w360 stop-if-true
        n374 = local read "START"() -> (w357:bool)
        n375 = Not(x=w357) -> (.not. x?=w356:bool)
        n376 = Compound Arithmetic op=OR(w356, "Play", "Load video", "stop") -> (w360:bool)
        n377 = case shown="True" "stop" {
          frame False {
          }
          frame True {
            w362 = FALSE ("Play")
            n378 = local write "stop"(w362) -> ()
            n379 = local write "Play"(w362) -> ()
          }
        }
      }
      n380 = property on="Progress..." class="Slide (strict)"("Scale.Maximum"=w352) -> ()  [unwired: 2 in, 2 out]
      n381 = Increment(x=w333) -> (x+1=w334:i64)
      n382 = Greater Or Equal?(x=w334, y=w351) -> (x >= y?=w337:bool)
      n383 = Select(t=w351, s=w337, f=w333) -> (s? t:f=w348:i64)
      "Video Frame" <- w348
      n384 = call "IMAQ AVI Read Frame"("error in (no error)"=w353, "Frame Number"=w348, "Image"=w354, "Avi Refnum"=w355) -> ("Image Out"=→"Video":T2, "Avi Refnum (duplicate)"=w330:T6)  [unwired: 4 in, 2 out]
      n385 = Search 1D Array(1D array=w346, element=w348) -> ()  [unwired: 1 in, 1 out]
      n386 = Or(x="fast forward", y="fast rewind") -> (x .or. y?=w328:bool)
      n387 = Increment(x="Progress...") -> (x+1=w329:u32)
      n388 = Select(t=1.0, s=w328, f="playback speed") -> (s? t:f=w340:dbl)
      n389 = Increment(x=w329) -> (x+1=w332:u32)
      n390 = local read "framesPerSecond"() -> (w345:u32)
      n391 = Select(t=w332, s="fast forward", f=w329) -> (s? t:f=w324:u32)
      n392 = Subtract(x="Progress...", y=2) -> (x-y=w325:u32)
      n393 = Divide(x=1000.0, y=w340) -> (x/y=w344:dbl)
      n394 = Divide(x=w344, y=w345) -> (x/y=w342:dbl)
      n395 = Select(t=w325, s="fast rewind", f=w324) -> (s? t:f=w323:u32)
      n396 = Round Toward -Infinity(1:w342) -> (0:w341:dbl)
      "playback speed" <- w341
      n397 = Wait (ms)(milliseconds to wait=w341) -> ()  [unwired: 1 out]
      n398 = local read "Load video"() -> (w335:bool)
      n399 = Select(t="Progress...", s=w337, f=w323) -> (s? t:f=w336:u32)
      n400 = case shown="True" w335 {
        tunnel: w346 -> [w363 _]
        tunnel: w336 -> [w364 _]
        tunnel: [w364 w365] -> w350
        tunnel: [w363 w368] -> w347
        frame False {
        }
        frame True {
          n401 = local read "frames 2 play"() -> (w368:i64[])
          n402 = Array Max & Min(array=w368) -> (max index (indices)=w367:i32)  [unwired: 3 out]
          n403 = property on="Progress..." class="Slide (strict)"("Scale.Maximum"=w367) -> ()  [unwired: 2 in, 2 out]
          n404 = local write "Load video"(FALSE ("Play")) -> ()
          n405 = local read "Progress..."() -> (w365:u32)
        }
      }
      n406 = local write "Progress..."(w350) -> ()
      n407 = local read "START"() -> (w331:bool)
    }
    n408 = while {
      shift-right: [w372] -> _
      shift-left: T1."Display" ("Main tab") -> [w373]
      tunnel: w10 -> [w386]
      shift-right: [w376] -> _
      shift-left: w11 -> [w389]
      tunnel: w8 -> [_]
      tunnel: w1 -> [_]
      tunnel: [w374] -> w7
      stop <- w375 continue-if-true
      w379 = T1."Coding" ("Main tab")
      # "Moving to display tab"
      n409 = case shown="\"Coding\", Default" w373 {
        tunnel: w389 -> [w576 w1482 w1740 w2107 w2144 w2279]
        tunnel: [w420 w1482 w1740 w2107 w2144 w2261] -> w376
        tunnel: [T1."Edit video" ("Main tab") w1494 T1."Display" ("Main tab") T1."Edit coding" ("Main tab") w2145 T1."Edit video" ("Main tab")] -> w381
        tunnel: w386 -> [w574 _ _ _ _ _]
        tunnel: [w416 w1487 w1754 w2105 w2142 w2267] -> w374
        frame "Coding", Default {
          n410 = local read "Drop"() -> (w572:bool)
          n411 = local read "Drop 2"() -> (w571:bool)
          n412 = local read "Drop 3"() -> (w570:bool)
          n413 = local read "Drop 4"() -> (w569:bool)
          n414 = local read "Drop 5"() -> (w568:bool)
          n415 = local read "Drop 6"() -> (w567:bool)
          n416 = local read "Drop 7"() -> (w566:bool)
          n417 = local read "Drop 8"() -> (w565:bool)
          n418 = local read "Drop 9"() -> (w564:bool)
          n419 = local read "Drop 10"() -> (w563:bool)
          n420 = local read "Drop 11"() -> (w562:bool)
          n421 = local read "Drop 12"() -> (w561:bool)
          n422 = local read "Chop"() -> (w560:bool)
          n423 = local read "Chop 2"() -> (w559:bool)
          n424 = local read "Chop 3"() -> (w558:bool)
          n425 = local read "Chop 4"() -> (w557:bool)
          n426 = local read "Chop 5"() -> (w556:bool)
          n427 = local read "Chop 6"() -> (w555:bool)
          n428 = local read "Chop 7"() -> (w554:bool)
          n429 = local read "Chop 8"() -> (w553:bool)
          n430 = local read "Chop 9"() -> (w552:bool)
          n431 = local read "Chop 10"() -> (w551:bool)
          n432 = local read "Chop 11"() -> (w550:bool)
          n433 = local read "Chop 12"() -> (w549:bool)
          n434 = local read "Let"() -> (w548:bool)
          n435 = local read "Unexpected Winner2"() -> (w539:bool)
          n436 = local read "Unexpected Winner1"() -> (w538:bool)
          n437 = local read "Expected Winner2"() -> (w537:bool)
          n438 = local read "Expected Winner1"() -> (w536:bool)
          n439 = local read "Forced Error2"() -> (w542:bool)
          n440 = local read "Forced Error1"() -> (w540:bool)
          n441 = local read "Nolet2"() -> (w547:bool)
          n442 = local read "Nolet1"() -> (w546:bool)
          n443 = local read "Stroke2"() -> (w545:bool)
          n444 = local read "Stroke1"() -> (w544:bool)
          n445 = local read "Unforced Error2"() -> (w543:bool)
          n446 = local read "Unforced Error1"() -> (w541:bool)
          n447 = Build Array(w572, w571, w570, w569, w568, w567, w566, w565, w564, w563, w562, w561, w560, w559, w558, w557, w556, w555, w554, w553, w552, w551, w550, w549, w548, w547, w546, w545, w544, w543, w542, w541, w540, w539, w538, w537, w536) -> (w426:bool[])
          n448 = local read "lob 13"() -> (w535:bool)
          n449 = local read "lob 2"() -> (w534:bool)
          n450 = local read "lob 3"() -> (w533:bool)
          n451 = local read "lob 4"() -> (w532:bool)
          n452 = local read "lob 5"() -> (w531:bool)
          n453 = local read "lob 6"() -> (w530:bool)
          n454 = local read "lob 7"() -> (w529:bool)
          n455 = local read "lob 8"() -> (w528:bool)
          n456 = local read "lob 9"() -> (w527:bool)
          n457 = local read "lob 10"() -> (w526:bool)
          n458 = local read "lob 11"() -> (w525:bool)
          n459 = local read "lob 12"() -> (w524:bool)
          n460 = local read "Smash"() -> (w523:bool)
          n461 = local read "Smash 2"() -> (w522:bool)
          n462 = local read "Smash 3"() -> (w521:bool)
          n463 = local read "Smash 4"() -> (w520:bool)
          n464 = local read "Smash 5"() -> (w519:bool)
          n465 = local read "Smash 6"() -> (w518:bool)
          n466 = local read "Smash 7"() -> (w517:bool)
          n467 = local read "Smash 8"() -> (w516:bool)
          n468 = local read "Smash 9"() -> (w515:bool)
          n469 = local read "Smash 10"() -> (w514:bool)
          n470 = local read "Smash 11"() -> (w513:bool)
          n471 = local read "Smash 12"() -> (w512:bool)
          n472 = local read "Boast"() -> (w511:bool)
          n473 = local read "Boast 2"() -> (w510:bool)
          n474 = local read "Boast 3"() -> (w509:bool)
          n475 = local read "Boast 4"() -> (w508:bool)
          n476 = local read "Boast 5"() -> (w507:bool)
          n477 = local read "Boast 6"() -> (w506:bool)
          n478 = local read "Boast 7"() -> (w505:bool)
          n479 = local read "Boast 8"() -> (w504:bool)
          n480 = local read "Boast 9"() -> (w503:bool)
          n481 = local read "Boast 10"() -> (w502:bool)
          n482 = local read "Boast 11"() -> (w501:bool)
          n483 = local read "Boast 12"() -> (w500:bool)
          n484 = Build Array(w535, w534, w533, w532, w531, w530, w529, w528, w527, w526, w525, w524, w523, w522, w521, w520, w519, w518, w517, w516, w515, w514, w513, w512, w511, w510, w509, w508, w507, w506, w505, w504, w503, w502, w501, w500) -> (w425:bool[])
          n485 = local read "Player2"() -> (w417:bool)
          n486 = local read "Player1"() -> (w418:bool)
          n487 = local read "Pause"() -> (w419:bool)
          n488 = local read "ADrive"() -> (w499:bool)
          n489 = local read "ADrive 2"() -> (w498:bool)
          n490 = local read "ADrive 3"() -> (w497:bool)
          n491 = local read "ADrive 4"() -> (w496:bool)
          n492 = local read "ADrive 5"() -> (w495:bool)
          n493 = local read "ADrive 6"() -> (w494:bool)
          n494 = local read "ADrive 7"() -> (w493:bool)
          n495 = local read "ADrive 8"() -> (w492:bool)
          n496 = local read "ADrive 9"() -> (w491:bool)
          n497 = local read "ADrive 10"() -> (w490:bool)
          n498 = local read "ADrive 11"() -> (w489:bool)
          n499 = local read "ADrive 12"() -> (w488:bool)
          n500 = local read "SWADrive"() -> (w487:bool)
          n501 = local read "SWADrive 2"() -> (w486:bool)
          n502 = local read "SWADrive 3"() -> (w485:bool)
          n503 = local read "SWADrive 4"() -> (w484:bool)
          n504 = local read "SWADrive 5"() -> (w483:bool)
          n505 = local read "SWADrive 6"() -> (w482:bool)
          n506 = local read "SWADrive 7"() -> (w481:bool)
          n507 = local read "SWADrive 8"() -> (w480:bool)
          n508 = local read "SWADrive 9"() -> (w479:bool)
          n509 = local read "SWADrive 10"() -> (w478:bool)
          n510 = local read "SWADrive 11"() -> (w477:bool)
          n511 = local read "SWADrive 12"() -> (w476:bool)
          n512 = local read "S6"() -> (w473:bool)
          n513 = local read "S5"() -> (w472:bool)
          n514 = local read "S4"() -> (w471:bool)
          n515 = local read "S1"() -> (w470:bool)
          n516 = local read "S2"() -> (w469:bool)
          n517 = local read "S3"() -> (w468:bool)
          n518 = local read "Service2"() -> (w475:bool)
          n519 = local read "Service1"() -> (w474:bool)
          n520 = Build Array(w499, w498, w497, w496, w495, w494, w493, w492, w491, w490, w489, w488, w487, w486, w485, w484, w483, w482, w481, w480, w479, w478, w477, w476, w475, w474, w473, w472, w471, w470, w469, w468, w419, w418, w417) -> (w424:bool[])
          n521 = local read "DDrive"() -> (w467:bool)
          n522 = local read "DDrive 2"() -> (w466:bool)
          n523 = local read "DDrive 3"() -> (w465:bool)
          n524 = local read "DDrive 4"() -> (w464:bool)
          n525 = local read "DDrive 5"() -> (w463:bool)
          n526 = local read "DDrive 6"() -> (w462:bool)
          n527 = local read "DDrive 7"() -> (w461:bool)
          n528 = local read "DDrive 8"() -> (w460:bool)
          n529 = local read "DDrive 9"() -> (w459:bool)
          n530 = local read "DDrive 10"() -> (w458:bool)
          n531 = local read "DDrive 11"() -> (w457:bool)
          n532 = local read "DDrive 12"() -> (w456:bool)
          n533 = local read "SWDDrive"() -> (w455:bool)
          n534 = local read "SWDDrive 2"() -> (w454:bool)
          n535 = local read "SWDDrive 3"() -> (w453:bool)
          n536 = local read "SWDDrive 4"() -> (w452:bool)
          n537 = local read "SWDDrive 5"() -> (w451:bool)
          n538 = local read "SWDDrive 6"() -> (w450:bool)
          n539 = local read "SWDDrive 7"() -> (w449:bool)
          n540 = local read "SWDDrive 8"() -> (w448:bool)
          n541 = local read "SWDDrive 9"() -> (w447:bool)
          n542 = local read "SWDDrive 10"() -> (w446:bool)
          n543 = local read "SWDDrive 11"() -> (w445:bool)
          n544 = local read "SWDDrive 12"() -> (w444:bool)
          n545 = local read "Button 5"() -> (w415:bool)
          n546 = local read "Button 4"() -> (w414:bool)
          n547 = local read "Button 3"() -> (w413:bool)
          n548 = local read "Button 2"() -> (w412:bool)
          n549 = local read "Button 1"() -> (w411:bool)
          n550 = Build Array(w467, w466, w465, w464, w463, w462, w461, w460, w459, w458, w457, w456, w455, w454, w453, w452, w451, w450, w449, w448, w447, w446, w445, w444) -> (w422:bool[])
          n551 = local read "4 4"() -> (w436:bool)
          n552 = local read "4 3"() -> (w437:bool)
          n553 = local read "4 2"() -> (w438:bool)
          n554 = local read "4 1"() -> (w439:bool)
          n555 = local read "3 4"() -> (w440:bool)
          n556 = local read "3 3"() -> (w441:bool)
          n557 = local read "3 2"() -> (w442:bool)
          n558 = local read "3 1"() -> (w443:bool)
          n559 = local read "2 4"() -> (w435:bool)
          n560 = local read "2 3"() -> (w434:bool)
          n561 = local read "2 2"() -> (w433:bool)
          n562 = local read "2 1"() -> (w432:bool)
          n563 = local read "1 4"() -> (w431:bool)
          n564 = local read "1 3"() -> (w430:bool)
          n565 = local read "1 2"() -> (w429:bool)
          n566 = local read "1 1"() -> (w428:bool)
          n567 = local read "5 4"() -> (w409:bool)
          n568 = local read "5 3"() -> (w408:bool)
          n569 = local read "5 2"() -> (w407:bool)
          n570 = local read "5 1"() -> (w406:bool)
          n571 = local read "6 4"() -> (w405:bool)
          n572 = local read "6 3"() -> (w404:bool)
          n573 = local read "6 2"() -> (w403:bool)
          n574 = local read "6 1"() -> (w402:bool)
          n575 = local read "Undo"() -> (w401:bool)
          n576 = Build Array(w415, w414, w413, w412, w411, w401) -> (w410:bool[])
          n577 = Build Array(w436, w437, w438, w439, w440, w441, w442, w443, w435, w434, w433, w432, w431, w430, w429, w428, w409, w408, w407, w406, w405, w404, w403, w402) -> (w423:bool[])
          n578 = local read "Video Frame"() -> (w573:u32)
          n579 = Build Array(w410, w422, w423, w424, w425, w426) -> (w427:bool[][])
          n580 = Or Array Elements(Boolean array=w427) -> (logical OR=w421:bool)
          n581 = case shown="True" w421 {
            tunnel: w573 -> [_ w739]
            tunnel: w576 -> [w580 w740]
            tunnel: [w580 w603] -> w420
            tunnel: w574 -> [_ w736]
            tunnel: [w577 w632] -> w416
            frame False {
              n582 = local read "Data file"() -> (w578:path)
              n583 = Open/Create/Replace File(file path (use dialog)=w578, operation (0:open)=T3."open") -> (refnum out=w577:refnum<file>)  [unwired: 4 in, 2 out]
            }
            frame True {
              w597 = 0 ("index")
              w607 = "\t"
              w643 = "\r"
              # "extra code buttons\n\nundo button / error button\n\nlink all (extra buttons) to linkshots logic"
              n584 = stacked-sequence {
                tunnel: w740 -> [w764 _ _ _ _ _ _ _ _ _ _ _ _ _ w1430 _]
                tunnel: [w764 _ _ _ _ _ _ _ _ _ _ _ _ _ _ _] -> w601
                tunnel: w739 -> [w770 _ _ _ _ _ _ _ _ _ _ _ _ _ _ _]
                tunnel: [w770 _ _ _ _ _ _ _ _ _ _ _ _ _ _ _] -> w605
                tunnel: w736 -> [w769 _ _ _ _ _ _ _ _ _ _ _ _ _ _ _]
                tunnel: [w766 _ _ _ _ _ _ _ _ _ _ _ _ _ _ _] -> w735
                tunnel: [_ _ "before 2" _ _ _ _ _ _ _ _ _ _ _ _ _] -> w734
                tunnel: [_ _ "after 2" _ _ _ _ _ _ _ _ _ _ _ _ _] -> w733
                tunnel: [_ _ w851 _ _ _ _ _ _ _ _ _ _ _ _ _] -> w732
                tunnel: [_ _ w850 _ _ _ _ _ _ _ _ _ _ _ _ _] -> w731
                tunnel: [_ _ w849 _ _ _ _ _ _ _ _ _ _ _ _ _] -> w730
                tunnel: [_ _ w848 _ _ _ _ _ _ _ _ _ _ _ _ _] -> w729
                tunnel: [_ _ w847 _ _ _ _ _ _ _ _ _ _ _ _ _] -> w728
                tunnel: [_ _ w846 _ _ _ _ _ _ _ _ _ _ _ _ _] -> w727
                tunnel: [_ _ w845 _ _ _ _ _ _ _ _ _ _ _ _ _] -> w726
                tunnel: [_ _ w844 _ _ _ _ _ _ _ _ _ _ _ _ _] -> w725
                tunnel: [_ _ w843 _ _ _ _ _ _ _ _ _ _ _ _ _] -> w724
                tunnel: [_ _ w842 _ _ _ _ _ _ _ _ _ _ _ _ _] -> w723
                tunnel: [_ _ w841 _ _ _ _ _ _ _ _ _ _ _ _ _] -> w722
                tunnel: [_ _ w840 _ _ _ _ _ _ _ _ _ _ _ _ _] -> w721
                tunnel: [_ _ w839 _ _ _ _ _ _ _ _ _ _ _ _ _] -> w720
                tunnel: [_ _ w838 _ _ _ _ _ _ _ _ _ _ _ _ _] -> w719
                tunnel: [_ _ w837 _ _ _ _ _ _ _ _ _ _ _ _ _] -> w718
                tunnel: [_ _ w836 _ _ _ _ _ _ _ _ _ _ _ _ _] -> w717
                tunnel: [_ _ w835 _ _ _ _ _ _ _ _ _ _ _ _ _] -> w716
                tunnel: [_ _ w834 _ _ _ _ _ _ _ _ _ _ _ _ _] -> w715
                tunnel: [_ _ w833 _ _ _ _ _ _ _ _ _ _ _ _ _] -> w714
                tunnel: [_ _ w832 _ _ _ _ _ _ _ _ _ _ _ _ _] -> w713
                tunnel: [_ _ w831 _ _ _ _ _ _ _ _ _ _ _ _ _] -> w712
                tunnel: [_ _ w830 _ _ _ _ _ _ _ _ _ _ _ _ _] -> w711
                tunnel: [_ _ w829 _ _ _ _ _ _ _ _ _ _ _ _ _] -> w710
                tunnel: [_ _ w828 _ _ _ _ _ _ _ _ _ _ _ _ _] -> w709
                tunnel: [_ _ _ w893 _ _ _ _ _ _ _ _ _ _ _ _] -> w708
                tunnel: [_ _ _ w892 _ _ _ _ _ _ _ _ _ _ _ _] -> w707
                tunnel: [_ _ _ w891 _ _ _ _ _ _ _ _ _ _ _ _] -> w706
                tunnel: [_ _ _ w890 _ _ _ _ _ _ _ _ _ _ _ _] -> w705
                tunnel: [_ _ _ _ w948 _ _ _ _ _ _ _ _ _ _ _] -> w704
                tunnel: [_ _ _ _ w947 _ _ _ _ _ _ _ _ _ _ _] -> w703
                tunnel: [_ _ _ _ w946 _ _ _ _ _ _ _ _ _ _ _] -> w702
                tunnel: [_ _ _ _ _ w990 _ _ _ _ _ _ _ _ _ _] -> w701
                tunnel: [_ _ _ _ _ w989 _ _ _ _ _ _ _ _ _ _] -> w700
                tunnel: [_ _ _ _ _ w988 _ _ _ _ _ _ _ _ _ _] -> w699
                tunnel: [_ _ _ _ _ _ w1018 _ _ _ _ _ _ _ _ _] -> w698
                tunnel: [_ _ _ _ _ _ _ w1076 _ _ _ _ _ _ _ _] -> w697
                tunnel: [_ _ _ _ _ _ _ _ w1134 _ _ _ _ _ _ _] -> w696
                tunnel: [_ _ _ _ _ _ _ _ _ w1186 _ _ _ _ _ _] -> w695
                tunnel: [_ _ _ _ _ _ _ _ _ _ w1250 _ _ _ _ _] -> w694
                tunnel: [_ _ _ _ _ _ _ _ _ _ _ w1290 _ _ _ _] -> w693
                tunnel: [_ _ _ _ _ _ _ _ _ _ _ _ w1330 _ _ _] -> w692
                tunnel: [_ _ _ _ _ _ _ _ _ _ _ _ _ _ w1393 _] -> w691
                tunnel: [_ _ _ _ _ _ _ _ _ _ _ _ _ _ w1394 _] -> w690
                tunnel: [_ _ _ _ _ _ _ _ _ _ _ _ _ _ w1395 _] -> w689
                tunnel: [_ _ _ _ _ _ _ _ _ _ _ _ _ _ w1400 _] -> w688
                tunnel: [_ _ _ _ _ _ _ _ _ _ _ _ _ _ w1401 _] -> w687
                tunnel: [_ _ _ _ _ _ _ _ _ _ _ _ _ _ w1402 _] -> w686
                tunnel: [_ _ _ _ _ _ _ _ _ _ _ _ _ _ w1403 _] -> w685
                tunnel: [_ _ _ _ _ _ _ _ _ _ _ _ _ _ w1404 _] -> w684
                tunnel: [_ _ _ _ _ _ _ _ _ _ _ _ _ _ w1405 _] -> w683
                tunnel: [_ _ _ _ _ _ _ _ _ _ _ _ _ _ w1406 _] -> w682
                tunnel: [_ _ _ _ _ _ _ _ _ _ _ _ _ _ w1407 _] -> w681
                tunnel: [_ _ _ _ _ _ _ _ _ _ _ _ _ _ w1408 _] -> w680
                tunnel: [_ _ _ _ _ _ _ _ _ _ _ _ _ _ w1408 _] -> w679
                tunnel: [_ _ _ _ _ _ _ _ _ _ _ _ _ _ w1396 _] -> w678
                tunnel: [_ _ _ _ _ _ _ _ _ _ _ _ _ _ w1397 _] -> w677
                tunnel: [_ _ _ _ _ _ _ _ _ _ _ _ _ _ w1398 _] -> w676
                tunnel: [_ _ _ _ _ _ _ _ _ _ _ _ _ _ w1399 _] -> w675
                tunnel: [_ _ _ _ _ _ _ _ _ _ _ _ _ _ _ w1449] -> w646
                tunnel: [_ _ _ _ _ _ _ _ _ _ _ _ _ w1379 _ _] -> w631
                tunnel: [_ _ _ _ _ _ _ _ _ _ _ _ _ w1378 _ _] -> w630
                tunnel: [_ _ _ _ _ _ _ _ _ _ _ _ _ w1377 _ _] -> w629
                tunnel: [_ _ _ _ _ _ _ _ _ _ _ _ _ w1376 _ _] -> w628
                tunnel: [_ _ _ _ _ _ _ _ _ _ _ _ _ w1375 _ _] -> w627
                tunnel: [_ _ w815 _ _ _ _ _ _ _ _ _ _ _ _ _] -> w619
                tunnel: [_ _ _ _ _ _ _ _ _ _ _ _ _ w1374 _ _] -> w618
                tunnel: [_ _ _ _ _ _ _ _ _ _ _ _ _ w1373 _ _] -> w617
                tunnel: [_ _ _ _ _ _ _ _ _ _ _ _ _ w1372 _ _] -> w616
                tunnel: [_ _ _ _ _ _ _ _ _ _ _ _ _ w1371 _ _] -> w615
                tunnel: [_ _ _ _ _ _ _ _ _ _ _ _ _ w1370 _ _] -> w614
                tunnel: [_ _ w819 _ _ _ _ _ _ _ _ _ _ _ _ _] -> w613
                tunnel: [_ _ w818 _ _ _ _ _ _ _ _ _ _ _ _ _] -> w612
                tunnel: [_ _ w817 _ _ _ _ _ _ _ _ _ _ _ _ _] -> w611
                tunnel: [_ _ w816 _ _ _ _ _ _ _ _ _ _ _ _ _] -> w610
                frame #0 {
                  n585 = local read "Pause"() -> (w765:bool)
                  n586 = And(x=w765, y="Pause lag on") -> (x .and. y?=w768:bool)
                  n587 = case shown="False" w765 {
                    frame False {
                      n588 = Tick Count (ms)() -> (millisecond timer value=w771:u32)
                      n589 = while {
                        tunnel: w771 -> [w783]
                        i -> [w774]
                        stop <- w781 stop-if-true
                        w777 = u32 25 ("milliseconds to wait")
                        n590 = Tick Count (ms)() -> (millisecond timer value=w784:u32)
                        n591 = Subtract(x=w784, y=w783) -> (x-y=w782:u32)
                        n592 = Multiply(x="Code lag(s)", y=1000) -> (x*y=w778:dbl)
                        n593 = Greater Or Equal?(x=w782, y=w778) -> (x >= y?=w781:bool)
                        n594 = Divide(x=w778, y=w777) -> (x/y=w776:dbl)
                        n595 = Divide(x=300.0, y=w776) -> (x/y=w773:dbl)
                        n596 = Multiply(x=w774, y=w773) -> (x*y=→"task":dbl)
                        n597 = Wait (ms)(milliseconds to wait=w777) -> ()  [unwired: 1 out]
                      }
                    }
                    frame True {
                    }
                  }
                  n598 = case shown="True" w768 {
                    tunnel: w770 -> [_ w788]
                    tunnel: w769 -> [_ w790]
                    tunnel: ["pauselag" ("Image Name") w786] -> w766
                    frame False {
                    }
                    frame True {
                      w791 = T5 4 items=["Grayscale (U8)", "Grayscale (I16)", "Grayscale (SGL)", "Complex (CSG)", "RGB (U32)", "HSL (U32)", "RGB (U64)"] ("Image Type")
                      n599 = local read "framesPerSecond"() -> (w797:u32)
                      n600 = local read "Number of Frames"() -> (w787:u32)
                      n601 = Increment(x=w788) -> (x+1=w789:u32)
                      n602 = Multiply(x="Pause lag(s)", y=w797) -> (x*y=w795:dbl)
                      n603 = call "IMAQ Create"("Image Name"="pauselag", "Image Type"=w791) -> ("New Image"=w786:T2, "error out"=w792:errorcluster)  [unwired: 3 in]
                      n604 = Round Toward +Infinity(x=w795) -> (ceil(x): smallest int >= x=w794:dbl)
                      n605 = for {
                        N: w794 -> [_]
                        tunnel: w789 -> [w804]
                        tunnel: w792 -> [w807]
                        tunnel: w786 -> [w806]
                        tunnel: w790 -> [w803]
                        tunnel: w787 -> [w801]
                        i -> [w805]
                        n606 = Add(x=w805, y=w804) -> (x+y=w800:u32)
                        n607 = local read "playback speed"() -> (w798:dbl)
                        n608 = Less Or Equal?(x=w801, y=w800) -> (x <= y?=w802:bool)
                        n609 = Select(t=w801, s=w802, f=w800) -> (s? t:f=w799:u32)
                        n610 = call "IMAQ AVI Read Frame"("error in (no error)"=w807, "Frame Number"=w799, "Image"=w806, "Avi Refnum"=w803) -> ("Image Out"=w808:T2)  [unwired: 4 in, 3 out]
                        n611 = local write "Video"(w808) -> ()
                        n612 = Wait (ms)(milliseconds to wait=w798) -> ()  [unwired: 1 out]
                      }
                    }
                  }
                }
                frame #1 {
                  w809 = i16 0 ("Service")
                  n613 = while {
                    stop <- w810 continue-if-true
                    n614 = local read "START"() -> (w811:bool)
                    n615 = local read "Pause"() -> (w812:bool)
                    n616 = And(x=w811, y=w812) -> (x .and. y?=w810:bool)
                  }
                  n617 = local write "Service"(w809) -> ()
                  n618 = local write "Cross"(w809) -> ()
                  n619 = local write "Straight"(w809) -> ()
                  n620 = local write "position"(w809) -> ()
                  n621 = local write "Player 1/2"(w809) -> ()
                  n622 = local write "Extra"(w809) -> ()
                }
                frame #2 {
                  n623 = local read "Service1"() -> (w859:bool)
                  n624 = local read "Service2"() -> (w861:bool)
                  n625 = Compound Arithmetic op=OR(w859, "Player1", w861, "Player2") -> (w858:bool)
                  n626 = Or(x="Player1", y="Player2") -> (x .or. y?=w864:bool)
                  n627 = case shown="True" w858 {
                    tunnel: w859 -> [_ w887]
                    tunnel: w861 -> [_ w886]
                    tunnel: "Player1" -> [_ w885]
                    tunnel: "Player2" -> [_ w884]
                    frame False {
                    }
                    frame True {
                      n628 = Or(x=w887, y=w885) -> (x .or. y?=w889:bool)
                      n629 = Or(x=w886, y=w884) -> (x .or. y?=w888:bool)
                      n630 = Build Array(w889, w888) -> (w883:bool[])
                      n631 = local write "Player1/Player2"(w883) -> ()
                    }
                  }
                  n632 = Boolean To (0,1)(Boolean=w864) -> (0, 1=→"Player 1/2":i16)
                  n633 = Boolean To (0,1)(Boolean="1 1") -> (0, 1=w851:i16)
                  n634 = Boolean To (0,1)(Boolean="1 2") -> (0, 1=w850:i16)
                  n635 = Boolean To (0,1)(Boolean="1 3") -> (0, 1=w849:i16)
                  n636 = Boolean To (0,1)(Boolean="1 4") -> (0, 1=w848:i16)
                  n637 = Boolean To (0,1)(Boolean="2 1") -> (0, 1=w847:i16)
                  n638 = Boolean To (0,1)(Boolean="2 2") -> (0, 1=w846:i16)
                  n639 = Boolean To (0,1)(Boolean="2 3") -> (0, 1=w845:i16)
                  n640 = Boolean To (0,1)(Boolean="2 4") -> (0, 1=w844:i16)
                  n641 = Boolean To (0,1)(Boolean="3 1") -> (0, 1=w843:i16)
                  n642 = Boolean To (0,1)(Boolean="3 2") -> (0, 1=w842:i16)
                  n643 = Boolean To (0,1)(Boolean="3 3") -> (0, 1=w841:i16)
                  n644 = Boolean To (0,1)(Boolean="3 4") -> (0, 1=w840:i16)
                  n645 = Boolean To (0,1)(Boolean="4 1") -> (0, 1=w839:i16)
                  n646 = Boolean To (0,1)(Boolean="4 2") -> (0, 1=w838:i16)
                  n647 = Boolean To (0,1)(Boolean="4 3") -> (0, 1=w837:i16)
                  n648 = Boolean To (0,1)(Boolean="4 4") -> (0, 1=w836:i16)
                  n649 = Boolean To (0,1)(Boolean="5 1") -> (0, 1=w835:i16)
                  n650 = Boolean To (0,1)(Boolean="5 2") -> (0, 1=w834:i16)
                  n651 = Boolean To (0,1)(Boolean="5 3") -> (0, 1=w833:i16)
                  n652 = Boolean To (0,1)(Boolean="5 4") -> (0, 1=w832:i16)
                  n653 = Boolean To (0,1)(Boolean="6 1") -> (0, 1=w831:i16)
                  n654 = Boolean To (0,1)(Boolean="6 2") -> (0, 1=w830:i16)
                  n655 = Boolean To (0,1)(Boolean="6 3") -> (0, 1=w829:i16)
                  n656 = Boolean To (0,1)(Boolean="6 4") -> (0, 1=w828:i16)
                  n657 = Compound Arithmetic op=OR("1 1", "1 2", "1 3", "1 4", "2 1", "2 2", "2 3", "2 4", "3 1", "3 2", "3 3", "3 4", "4 1", "4 2", "4 3", "4 4", "5 1", "5 2", "5 3", "5 4", "6 1", "6 2", "6 3", "6 4") -> (w882:bool)
                  n658 = Boolean To (0,1)(Boolean=w882) -> (0, 1=→"position":i16)
                  n659 = Boolean To (0,1)(Boolean="Button 1") -> (0, 1=w819:i16)
                  n660 = Boolean To (0,1)(Boolean="Button 2") -> (0, 1=w818:i16)
                  n661 = Boolean To (0,1)(Boolean="Button 3") -> (0, 1=w817:i16)
                  n662 = Boolean To (0,1)(Boolean="Button 4") -> (0, 1=w816:i16)
                  n663 = Boolean To (0,1)(Boolean="Button 5") -> (0, 1=w815:i16)
                  n664 = Compound Arithmetic op=OR(w819, w818, w817, w816, w815) -> (→"Extra":i16)
                }
                frame #3 {
                  n665 = Compound Arithmetic op=OR("ADrive", "ADrive 2", "ADrive 3", "ADrive 4", "ADrive 5", "ADrive 6", "ADrive 7", "ADrive 8", "ADrive 9", "ADrive 10", "ADrive 11", "ADrive 12") -> (w945:bool)
                  n666 = Compound Arithmetic op=OR("SWADrive", "SWADrive 2", "SWADrive 3", "SWADrive 4", "SWADrive 5", "SWADrive 6", "SWADrive 7", "SWADrive 8", "SWADrive 9", "SWADrive 10", "SWADrive 11", "SWADrive 12") -> (w906:bool)
                  n667 = Boolean To (0,1)(Boolean=w945) -> (0, 1=w893:i16)
                  n668 = Boolean To (0,1)(Boolean=w906) -> (0, 1=w891:i16)
                  n669 = Compound Arithmetic op=OR("DDrive", "DDrive 2", "DDrive 3", "DDrive 4", "DDrive 5", "DDrive 6", "DDrive 7", "DDrive 8", "DDrive 9", "DDrive 10", "DDrive 11", "DDrive 12") -> (w932:bool)
                  n670 = Compound Arithmetic op=OR("SWDDrive", "SWDDrive 2", "SWDDrive 3", "SWDDrive 4", "SWDDrive 5", "SWDDrive 6", "SWDDrive 7", "SWDDrive 8", "SWDDrive 9", "SWDDrive 10", "SWDDrive 11", "SWDDrive 12") -> (w919:bool)
                  n671 = Boolean To (0,1)(Boolean=w932) -> (0, 1=w892:i16)
                  n672 = Boolean To (0,1)(Boolean=w919) -> (0, 1=w890:i16)
                }
                frame #4 {
                  n673 = Compound Arithmetic op=OR("Chop", "Chop 2", "Chop 3", "Chop 4", "Chop 5", "Chop 6", "Chop 7", "Chop 8", "Chop 9", "Chop 10", "Chop 11", "Chop 12") -> (w985:bool)
                  n674 = Boolean To (0,1)(Boolean=w985) -> (0, 1=w947:i16)
                  n675 = Compound Arithmetic op=OR("lob 13", "lob 2", "lob 3", "lob 4", "lob 5", "lob 6", "lob 7", "lob 8", "lob 9", "lob 10", "lob 11", "lob 12") -> (w986:bool)
                  n676 = Compound Arithmetic op=OR("Drop", "Drop 2", "Drop 3", "Drop 4", "Drop 5", "Drop 6", "Drop 7", "Drop 8", "Drop 9", "Drop 10", "Drop 11", "Drop 12") -> (w987:bool)
                  n677 = Boolean To (0,1)(Boolean=w987) -> (0, 1=w948:i16)
                  n678 = Boolean To (0,1)(Boolean=w986) -> (0, 1=w946:i16)
                }
                frame #5 {
                  n679 = Compound Arithmetic op=OR("Boast 2", "Boast 4", "Boast 6", "Boast 8", "Boast 10", "Boast 12") -> (w1009:bool)
                  n680 = Boolean To (0,1)(Boolean=w1009) -> (0, 1=w989:i16)
                  n681 = Compound Arithmetic op=OR("Smash", "Smash 2", "Smash 3", "Smash 4", "Smash 5", "Smash 6", "Smash 7", "Smash 8", "Smash 9", "Smash 10", "Smash 11", "Smash 12") -> (w1016:bool)
                  n682 = Compound Arithmetic op=OR("Boast", "Boast 3", "Boast 5", "Boast 7", "Boast 9", "Boast 11") -> (w1017:bool)
                  n683 = Boolean To (0,1)(Boolean=w1017) -> (0, 1=w990:i16)
                  n684 = Boolean To (0,1)(Boolean=w1016) -> (0, 1=w988:i16)
                }
                frame #6 {
                  # "forehand"
                  n685 = local read "Smash 10"() -> (w1052:bool)
                  n686 = local read "Chop 10"() -> (w1064:bool)
                  n687 = local read "Smash 2"() -> (w1056:bool)
                  n688 = local read "Smash 5"() -> (w1055:bool)
                  n689 = local read "Smash 6"() -> (w1054:bool)
                  n690 = local read "Smash 9"() -> (w1053:bool)
                  n691 = local read "Boast 10"() -> (w1046:bool)
                  n692 = local read "Drop 10"() -> (w1070:bool)
                  n693 = local read "Chop 2"() -> (w1068:bool)
                  n694 = local read "Chop 5"() -> (w1067:bool)
                  n695 = local read "Chop 6"() -> (w1066:bool)
                  n696 = local read "Chop 9"() -> (w1065:bool)
                  n697 = local read "Boast 2"() -> (w1050:bool)
                  n698 = local read "Boast 5"() -> (w1049:bool)
                  n699 = local read "Boast 6"() -> (w1048:bool)
                  n700 = local read "Boast 9"() -> (w1047:bool)
                  n701 = local read "Drop 2"() -> (w1074:bool)
                  n702 = local read "Drop 5"() -> (w1073:bool)
                  n703 = local read "Drop 6"() -> (w1072:bool)
                  n704 = local read "Drop 9"() -> (w1071:bool)
                  n705 = local read "Smash"() -> (w1057:bool)
                  n706 = local read "lob 10"() -> (w1058:bool)
                  n707 = local read "Chop"() -> (w1069:bool)
                  n708 = local read "Boast"() -> (w1051:bool)
                  n709 = local read "Drop"() -> (w1075:bool)
                  n710 = local read "lob 2"() -> (w1062:bool)
                  n711 = local read "lob 5"() -> (w1061:bool)
                  n712 = local read "lob 6"() -> (w1060:bool)
                  n713 = local read "lob 9"() -> (w1059:bool)
                  n714 = local read "lob 13"() -> (w1063:bool)
                  n715 = Compound Arithmetic op=OR(w1075, w1074, w1073, w1072, w1071, w1070, w1069, w1068, w1067, w1066, w1065, w1064, w1063, w1062, w1061, w1060, w1059, w1058, w1057, w1056, w1055, w1054, w1053, w1052, w1051, w1050, w1049, w1048, w1047, w1046) -> (w1019:bool)
                  n716 = local read "SWADrive 10"() -> (w1039:bool)
                  n717 = local read "SWDDrive 10"() -> (w1045:bool)
                  n718 = local read "SWADrive 2"() -> (w1035:bool)
                  n719 = local read "SWADrive 5"() -> (w1036:bool)
                  n720 = local read "SWADrive 6"() -> (w1037:bool)
                  n721 = local read "SWADrive 9"() -> (w1038:bool)
                  n722 = local read "SWDDrive 2"() -> (w1041:bool)
                  n723 = local read "SWDDrive 5"() -> (w1042:bool)
                  n724 = local read "SWDDrive 6"() -> (w1043:bool)
                  n725 = local read "SWDDrive 9"() -> (w1044:bool)
                  n726 = local read "SWADrive"() -> (w1034:bool)
                  n727 = local read "SWDDrive"() -> (w1040:bool)
                  n728 = local read "ADrive 10"() -> (w1027:bool)
                  n729 = local read "DDrive 10"() -> (w1033:bool)
                  n730 = local read "ADrive 2"() -> (w1023:bool)
                  n731 = local read "ADrive 5"() -> (w1024:bool)
                  n732 = local read "ADrive 6"() -> (w1025:bool)
                  n733 = local read "ADrive 9"() -> (w1026:bool)
                  n734 = local read "DDrive 2"() -> (w1029:bool)
                  n735 = local read "DDrive 5"() -> (w1030:bool)
                  n736 = local read "DDrive 6"() -> (w1031:bool)
                  n737 = local read "DDrive 9"() -> (w1032:bool)
                  n738 = local read "ADrive"() -> (w1022:bool)
                  n739 = local read "DDrive"() -> (w1028:bool)
                  n740 = Compound Arithmetic op=OR(w1022, w1023, w1024, w1025, w1026, w1027, w1028, w1029, w1030, w1031, w1032, w1033, w1034, w1035, w1036, w1037, w1038, w1039, w1040, w1041, w1042, w1043, w1044, w1045) -> (w1020:bool)
                  n741 = Or(x=w1019, y=w1020) -> (x .or. y?=w1021:bool)
                  n742 = Boolean To (0,1)(Boolean=w1021) -> (0, 1=w1018:i16)
                }
                frame #7 {
                  # "backhand"
                  n743 = local read "Smash 11"() -> (w1108:bool)
                  n744 = local read "Smash 12"() -> (w1107:bool)
                  n745 = local read "Chop 11"() -> (w1120:bool)
                  n746 = local read "Chop 12"() -> (w1119:bool)
                  n747 = local read "Smash 3"() -> (w1112:bool)
                  n748 = local read "Smash 4"() -> (w1111:bool)
                  n749 = local read "Smash 7"() -> (w1110:bool)
                  n750 = local read "Smash 8"() -> (w1109:bool)
                  n751 = local read "Boast 11"() -> (w1102:bool)
                  n752 = local read "Boast 12"() -> (w1101:bool)
                  n753 = local read "Drop 11"() -> (w1126:bool)
                  n754 = local read "Drop 12"() -> (w1125:bool)
                  n755 = local read "Chop 3"() -> (w1124:bool)
                  n756 = local read "Chop 4"() -> (w1123:bool)
                  n757 = local read "Chop 7"() -> (w1122:bool)
                  n758 = local read "Chop 8"() -> (w1121:bool)
                  n759 = local read "Boast 3"() -> (w1106:bool)
                  n760 = local read "Boast 4"() -> (w1105:bool)
                  n761 = local read "Boast 7"() -> (w1104:bool)
                  n762 = local read "Boast 8"() -> (w1103:bool)
                  n763 = local read "Drop 3"() -> (w1130:bool)
                  n764 = local read "Drop 4"() -> (w1129:bool)
                  n765 = local read "Drop 7"() -> (w1128:bool)
                  n766 = local read "Drop 8"() -> (w1127:bool)
                  n767 = local read "lob 11"() -> (w1114:bool)
                  n768 = local read "lob 12"() -> (w1113:bool)
                  n769 = local read "lob 3"() -> (w1118:bool)
                  n770 = local read "lob 4"() -> (w1117:bool)
                  n771 = local read "lob 7"() -> (w1116:bool)
                  n772 = local read "lob 8"() -> (w1115:bool)
                  n773 = Compound Arithmetic op=OR(w1130, w1129, w1128, w1127, w1126, w1125, w1124, w1123, w1122, w1121, w1120, w1119, w1118, w1117, w1116, w1115, w1114, w1113, w1112, w1111, w1110, w1109, w1108, w1107, w1106, w1105, w1104, w1103, w1102, w1101) -> (w1131:bool)
                  n774 = local read "SWADrive 11"() -> (w1084:bool)
                  n775 = local read "SWADrive 12"() -> (w1083:bool)
                  n776 = local read "SWDDrive 11"() -> (w1078:bool)
                  n777 = local read "SWDDrive 12"() -> (w1077:bool)
                  n778 = local read "SWADrive 3"() -> (w1088:bool)
                  n779 = local read "SWADrive 4"() -> (w1087:bool)
                  n780 = local read "SWADrive 7"() -> (w1086:bool)
                  n781 = local read "SWADrive 8"() -> (w1085:bool)
                  n782 = local read "SWDDrive 3"() -> (w1082:bool)
                  n783 = local read "SWDDrive 4"() -> (w1081:bool)
                  n784 = local read "SWDDrive 7"() -> (w1080:bool)
                  n785 = local read "SWDDrive 8"() -> (w1079:bool)
                  n786 = local read "ADrive 11"() -> (w1096:bool)
                  n787 = local read "ADrive 12"() -> (w1095:bool)
                  n788 = local read "DDrive 11"() -> (w1090:bool)
                  n789 = local read "DDrive 12"() -> (w1089:bool)
                  n790 = local read "ADrive 3"() -> (w1100:bool)
                  n791 = local read "ADrive 4"() -> (w1099:bool)
                  n792 = local read "ADrive 7"() -> (w1098:bool)
                  n793 = local read "ADrive 8"() -> (w1097:bool)
                  n794 = local read "DDrive 3"() -> (w1094:bool)
                  n795 = local read "DDrive 4"() -> (w1093:bool)
                  n796 = local read "DDrive 7"() -> (w1092:bool)
                  n797 = local read "DDrive 8"() -> (w1091:bool)
                  n798 = Compound Arithmetic op=OR(w1100, w1099, w1098, w1097, w1096, w1095, w1094, w1093, w1092, w1091, w1090, w1089, w1088, w1087, w1086, w1085, w1084, w1083, w1082, w1081, w1080, w1079, w1078, w1077) -> (w1132:bool)
                  n799 = Or(x=w1131, y=w1132) -> (x .or. y?=w1133:bool)
                  n800 = Boolean To (0,1)(Boolean=w1133) -> (0, 1=w1076:i16)
                }
                frame #8 {
                  # "straight"
                  n801 = local read "Smash 11"() -> (w1159:bool)
                  n802 = local read "Chop 11"() -> (w1171:bool)
                  n803 = local read "Smash 3"() -> (w1163:bool)
                  n804 = local read "Smash 5"() -> (w1162:bool)
                  n805 = local read "Smash 7"() -> (w1161:bool)
                  n806 = local read "Smash 9"() -> (w1160:bool)
                  n807 = local read "Drop 11"() -> (w1177:bool)
                  n808 = local read "Chop 3"() -> (w1175:bool)
                  n809 = local read "Chop 5"() -> (w1174:bool)
                  n810 = local read "Chop 7"() -> (w1173:bool)
                  n811 = local read "Chop 9"() -> (w1172:bool)
                  n812 = local read "Drop 3"() -> (w1181:bool)
                  n813 = local read "Drop 5"() -> (w1180:bool)
                  n814 = local read "Drop 7"() -> (w1179:bool)
                  n815 = local read "Drop 9"() -> (w1178:bool)
                  n816 = local read "Smash"() -> (w1164:bool)
                  n817 = local read "lob 11"() -> (w1165:bool)
                  n818 = local read "Chop"() -> (w1176:bool)
                  n819 = local read "Drop"() -> (w1182:bool)
                  n820 = local read "lob 3"() -> (w1169:bool)
                  n821 = local read "lob 5"() -> (w1168:bool)
                  n822 = local read "lob 7"() -> (w1167:bool)
                  n823 = local read "lob 9"() -> (w1166:bool)
                  n824 = local read "lob 13"() -> (w1170:bool)
                  n825 = Compound Arithmetic op=OR(w1182, w1181, w1180, w1179, w1178, w1177, w1176, w1175, w1174, w1173, w1172, w1171, w1170, w1169, w1168, w1167, w1166, w1165, w1164, w1163, w1162, w1161, w1160, w1159) -> (w1183:bool)
                  n826 = local read "SWADrive 11"() -> (w1141:bool)
                  n827 = local read "SWDDrive 11"() -> (w1135:bool)
                  n828 = local read "SWADrive 3"() -> (w1145:bool)
                  n829 = local read "SWADrive 5"() -> (w1144:bool)
                  n830 = local read "SWADrive 7"() -> (w1143:bool)
                  n831 = local read "SWADrive 9"() -> (w1142:bool)
                  n832 = local read "SWDDrive 3"() -> (w1139:bool)
                  n833 = local read "SWDDrive 5"() -> (w1138:bool)
                  n834 = local read "SWDDrive 7"() -> (w1137:bool)
                  n835 = local read "SWDDrive 9"() -> (w1136:bool)
                  n836 = local read "SWADrive"() -> (w1146:bool)
                  n837 = local read "SWDDrive"() -> (w1140:bool)
                  n838 = local read "ADrive 11"() -> (w1153:bool)
                  n839 = local read "DDrive 11"() -> (w1147:bool)
                  n840 = local read "ADrive 3"() -> (w1157:bool)
                  n841 = local read "ADrive 5"() -> (w1156:bool)
                  n842 = local read "ADrive 7"() -> (w1155:bool)
                  n843 = local read "ADrive 9"() -> (w1154:bool)
                  n844 = local read "DDrive 3"() -> (w1151:bool)
                  n845 = local read "DDrive 5"() -> (w1150:bool)
                  n846 = local read "DDrive 7"() -> (w1149:bool)
                  n847 = local read "DDrive 9"() -> (w1148:bool)
                  n848 = local read "ADrive"() -> (w1158:bool)
                  n849 = local read "DDrive"() -> (w1152:bool)
                  n850 = Compound Arithmetic op=OR(w1158, w1157, w1156, w1155, w1154, w1153, w1152, w1151, w1150, w1149, w1148, w1147, w1146, w1145, w1144, w1143, w1142, w1141, w1140, w1139, w1138, w1137, w1136, w1135) -> (w1184:bool)
                  n851 = Or(x=w1183, y=w1184) -> (x .or. y?=w1185:bool)
                  n852 = Boolean To (0,1)(Boolean=w1185) -> (0, 1=w1134:i16)
                  "Straight" <- w1134
                }
                frame #9 {
                  # "cross"
                  n853 = local read "Smash 10"() -> (w1225:bool)
                  n854 = local read "Smash 12"() -> (w1224:bool)
                  n855 = local read "Chop 10"() -> (w1237:bool)
                  n856 = local read "Chop 12"() -> (w1236:bool)
                  n857 = local read "Smash 2"() -> (w1229:bool)
                  n858 = local read "Smash 4"() -> (w1228:bool)
                  n859 = local read "Smash 6"() -> (w1227:bool)
                  n860 = local read "Smash 8"() -> (w1226:bool)
                  n861 = local read "Boast 10"() -> (w1214:bool)
                  n862 = local read "Boast 11"() -> (w1213:bool)
                  n863 = local read "Boast 12"() -> (w1212:bool)
                  n864 = local read "Drop 10"() -> (w1243:bool)
                  n865 = local read "Drop 12"() -> (w1242:bool)
                  n866 = local read "Chop 2"() -> (w1241:bool)
                  n867 = local read "Chop 4"() -> (w1240:bool)
                  n868 = local read "Chop 6"() -> (w1239:bool)
                  n869 = local read "Chop 8"() -> (w1238:bool)
                  n870 = local read "Boast 2"() -> (w1222:bool)
                  n871 = local read "Boast 3"() -> (w1221:bool)
                  n872 = local read "Boast 4"() -> (w1220:bool)
                  n873 = local read "Boast 5"() -> (w1219:bool)
                  n874 = local read "Boast 6"() -> (w1218:bool)
                  n875 = local read "Boast 7"() -> (w1217:bool)
                  n876 = local read "Boast 8"() -> (w1216:bool)
                  n877 = local read "Boast 9"() -> (w1215:bool)
                  n878 = local read "Drop 2"() -> (w1247:bool)
                  n879 = local read "Drop 4"() -> (w1246:bool)
                  n880 = local read "Drop 6"() -> (w1245:bool)
                  n881 = local read "Drop 8"() -> (w1244:bool)
                  n882 = local read "lob 10"() -> (w1231:bool)
                  n883 = local read "lob 12"() -> (w1230:bool)
                  n884 = local read "Boast"() -> (w1223:bool)
                  n885 = local read "lob 2"() -> (w1235:bool)
                  n886 = local read "lob 4"() -> (w1234:bool)
                  n887 = local read "lob 6"() -> (w1233:bool)
                  n888 = local read "lob 8"() -> (w1232:bool)
                  n889 = Compound Arithmetic op=OR(w1247, w1246, w1245, w1244, w1243, w1242, w1241, w1240, w1239, w1238, w1237, w1236, w1235, w1234, w1233, w1232, w1231, w1230, w1229, w1228, w1227, w1226, w1225, w1224, w1223, w1222, w1221, w1220, w1219, w1218, w1217, w1216, w1215, w1214, w1213, w1212) -> (w1187:bool)
                  n890 = local read "SWADrive 10"() -> (w1195:bool)
                  n891 = local read "SWADrive 12"() -> (w1194:bool)
                  n892 = local read "SWDDrive 10"() -> (w1189:bool)
                  n893 = local read "SWDDrive 12"() -> (w1188:bool)
                  n894 = local read "SWADrive 2"() -> (w1199:bool)
                  n895 = local read "SWADrive 4"() -> (w1198:bool)
                  n896 = local read "SWADrive 6"() -> (w1197:bool)
                  n897 = local read "SWADrive 8"() -> (w1196:bool)
                  n898 = local read "SWDDrive 2"() -> (w1193:bool)
                  n899 = local read "SWDDrive 4"() -> (w1192:bool)
                  n900 = local read "SWDDrive 6"() -> (w1191:bool)
                  n901 = local read "SWDDrive 8"() -> (w1190:bool)
                  n902 = local read "ADrive 10"() -> (w1207:bool)
                  n903 = local read "ADrive 12"() -> (w1206:bool)
                  n904 = local read "DDrive 10"() -> (w1201:bool)
                  n905 = local read "DDrive 12"() -> (w1200:bool)
                  n906 = local read "ADrive 2"() -> (w1211:bool)
                  n907 = local read "ADrive 4"() -> (w1210:bool)
                  n908 = local read "ADrive 6"() -> (w1209:bool)
                  n909 = local read "ADrive 8"() -> (w1208:bool)
                  n910 = local read "DDrive 2"() -> (w1205:bool)
                  n911 = local read "DDrive 4"() -> (w1204:bool)
                  n912 = local read "DDrive 6"() -> (w1203:bool)
                  n913 = local read "DDrive 8"() -> (w1202:bool)
                  n914 = Compound Arithmetic op=OR(w1211, w1210, w1209, w1208, w1207, w1206, w1205, w1204, w1203, w1202, w1201, w1200, w1199, w1198, w1197, w1196, w1195, w1194, w1193, w1192, w1191, w1190, w1189, w1188) -> (w1248:bool)
                  n915 = Or(x=w1187, y=w1248) -> (x .or. y?=w1249:bool)
                  n916 = Boolean To (0,1)(Boolean=w1249) -> (0, 1=w1186:i16)
                  "Cross" <- w1186
                }
                frame #10 {
                  # "bounce"
                  n917 = local read "Smash 2"() -> (w1257:bool)
                  n918 = local read "Smash 3"() -> (w1256:bool)
                  n919 = local read "Smash 4"() -> (w1255:bool)
                  n920 = local read "Chop 2"() -> (w1281:bool)
                  n921 = local read "Chop 3"() -> (w1280:bool)
                  n922 = local read "Chop 4"() -> (w1279:bool)
                  n923 = local read "Boast 2"() -> (w1253:bool)
                  n924 = local read "Boast 3"() -> (w1252:bool)
                  n925 = local read "Boast 4"() -> (w1251:bool)
                  n926 = local read "Drop 2"() -> (w1285:bool)
                  n927 = local read "Drop 3"() -> (w1284:bool)
                  n928 = local read "Drop 4"() -> (w1283:bool)
                  n929 = local read "Smash"() -> (w1258:bool)
                  n930 = local read "Chop"() -> (w1282:bool)
                  n931 = local read "Boast"() -> (w1254:bool)
                  n932 = local read "Drop"() -> (w1286:bool)
                  n933 = local read "lob 2"() -> (w1260:bool)
                  n934 = local read "lob 3"() -> (w1261:bool)
                  n935 = local read "lob 4"() -> (w1259:bool)
                  n936 = local read "lob 13"() -> (w1262:bool)
                  n937 = Compound Arithmetic op=OR(w1286, w1285, w1284, w1283, w1282, w1281, w1280, w1279, w1262, w1260, w1261, w1259, w1258, w1257, w1256, w1255, w1254, w1253, w1252, w1251) -> (w1287:bool)
                  n938 = local read "SWADrive 2"() -> (w1269:bool)
                  n939 = local read "SWADrive 3"() -> (w1268:bool)
                  n940 = local read "SWADrive 4"() -> (w1267:bool)
                  n941 = local read "SWDDrive 2"() -> (w1265:bool)
                  n942 = local read "SWDDrive 3"() -> (w1264:bool)
                  n943 = local read "SWDDrive 4"() -> (w1263:bool)
                  n944 = local read "SWADrive"() -> (w1270:bool)
                  n945 = local read "SWDDrive"() -> (w1266:bool)
                  n946 = local read "ADrive 2"() -> (w1277:bool)
                  n947 = local read "ADrive 3"() -> (w1276:bool)
                  n948 = local read "ADrive 4"() -> (w1275:bool)
                  n949 = local read "DDrive 2"() -> (w1273:bool)
                  n950 = local read "DDrive 3"() -> (w1272:bool)
                  n951 = local read "DDrive 4"() -> (w1271:bool)
                  n952 = local read "ADrive"() -> (w1278:bool)
                  n953 = local read "DDrive"() -> (w1274:bool)
                  n954 = Compound Arithmetic op=OR(w1278, w1277, w1276, w1275, w1274, w1273, w1272, w1271, w1270, w1269, w1268, w1267, w1266, w1265, w1264, w1263) -> (w1288:bool)
                  n955 = Or(x=w1287, y=w1288) -> (x .or. y?=w1289:bool)
                  n956 = Boolean To (0,1)(Boolean=w1289) -> (0, 1=w1250:i16)
                }
                frame #11 {
                  # "volley"
                  n957 = local read "Smash 5"() -> (w1314:bool)
                  n958 = local read "Smash 6"() -> (w1313:bool)
                  n959 = local read "Smash 7"() -> (w1312:bool)
                  n960 = local read "Smash 8"() -> (w1311:bool)
                  n961 = local read "Chop 5"() -> (w1322:bool)
                  n962 = local read "Chop 6"() -> (w1321:bool)
                  n963 = local read "Chop 7"() -> (w1320:bool)
                  n964 = local read "Chop 8"() -> (w1319:bool)
                  n965 = local read "Boast 5"() -> (w1310:bool)
                  n966 = local read "Boast 6"() -> (w1309:bool)
                  n967 = local read "Boast 7"() -> (w1308:bool)
                  n968 = local read "Boast 8"() -> (w1307:bool)
                  n969 = local read "Drop 5"() -> (w1326:bool)
                  n970 = local read "Drop 6"() -> (w1325:bool)
                  n971 = local read "Drop 7"() -> (w1324:bool)
                  n972 = local read "Drop 8"() -> (w1323:bool)
                  n973 = local read "lob 5"() -> (w1318:bool)
                  n974 = local read "lob 6"() -> (w1317:bool)
                  n975 = local read "lob 7"() -> (w1316:bool)
                  n976 = local read "lob 8"() -> (w1315:bool)
                  n977 = Compound Arithmetic op=OR(w1326, w1325, w1324, w1323, w1322, w1321, w1320, w1319, w1318, w1317, w1316, w1315, w1314, w1313, w1312, w1311, w1310, w1309, w1308, w1307) -> (w1327:bool)
                  n978 = local read "SWADrive 5"() -> (w1298:bool)
                  n979 = local read "SWADrive 6"() -> (w1297:bool)
                  n980 = local read "SWADrive 7"() -> (w1296:bool)
                  n981 = local read "SWADrive 8"() -> (w1295:bool)
                  n982 = local read "SWDDrive 5"() -> (w1294:bool)
                  n983 = local read "SWDDrive 6"() -> (w1293:bool)
                  n984 = local read "SWDDrive 7"() -> (w1292:bool)
                  n985 = local read "SWDDrive 8"() -> (w1291:bool)
                  n986 = local read "ADrive 5"() -> (w1306:bool)
                  n987 = local read "ADrive 6"() -> (w1305:bool)
                  n988 = local read "ADrive 7"() -> (w1304:bool)
                  n989 = local read "ADrive 8"() -> (w1303:bool)
                  n990 = local read "DDrive 5"() -> (w1302:bool)
                  n991 = local read "DDrive 6"() -> (w1301:bool)
                  n992 = local read "DDrive 7"() -> (w1300:bool)
                  n993 = local read "DDrive 8"() -> (w1299:bool)
                  n994 = Compound Arithmetic op=OR(w1306, w1305, w1304, w1303, w1302, w1301, w1300, w1299, w1298, w1297, w1296, w1295, w1294, w1293, w1292, w1291) -> (w1328:bool)
                  n995 = Or(x=w1327, y=w1328) -> (x .or. y?=w1329:bool)
                  n996 = Boolean To (0,1)(Boolean=w1329) -> (0, 1=w1290:i16)
                }
                frame #12 {
                  # "half volley"
                  n997 = local read "Smash 10"() -> (w1353:bool)
                  n998 = local read "Smash 11"() -> (w1352:bool)
                  n999 = local read "Smash 12"() -> (w1351:bool)
                  n1000 = local read "Chop 10"() -> (w1361:bool)
                  n1001 = local read "Chop 11"() -> (w1360:bool)
                  n1002 = local read "Chop 12"() -> (w1359:bool)
                  n1003 = local read "Smash 9"() -> (w1354:bool)
                  n1004 = local read "Boast 10"() -> (w1349:bool)
                  n1005 = local read "Boast 11"() -> (w1348:bool)
                  n1006 = local read "Boast 12"() -> (w1347:bool)
                  n1007 = local read "Drop 10"() -> (w1365:bool)
                  n1008 = local read "Drop 11"() -> (w1364:bool)
                  n1009 = local read "Drop 12"() -> (w1363:bool)
                  n1010 = local read "Chop 9"() -> (w1362:bool)
                  n1011 = local read "Boast 9"() -> (w1350:bool)
                  n1012 = local read "Drop 9"() -> (w1366:bool)
                  n1013 = local read "lob 10"() -> (w1357:bool)
                  n1014 = local read "lob 11"() -> (w1356:bool)
                  n1015 = local read "lob 12"() -> (w1355:bool)
                  n1016 = local read "lob 9"() -> (w1358:bool)
                  n1017 = Compound Arithmetic op=OR(w1366, w1365, w1364, w1363, w1362, w1361, w1360, w1359, w1358, w1357, w1356, w1355, w1354, w1353, w1352, w1351, w1350, w1349, w1348, w1347) -> (w1367:bool)
                  n1018 = local read "SWADrive 10"() -> (w1337:bool)
                  n1019 = local read "SWADrive 11"() -> (w1336:bool)
                  n1020 = local read "SWADrive 12"() -> (w1335:bool)
                  n1021 = local read "SWDDrive 10"() -> (w1333:bool)
                  n1022 = local read "SWDDrive 11"() -> (w1332:bool)
                  n1023 = local read "SWDDrive 12"() -> (w1331:bool)
                  n1024 = local read "SWADrive 9"() -> (w1338:bool)
                  n1025 = local read "SWDDrive 9"() -> (w1334:bool)
                  n1026 = local read "ADrive 10"() -> (w1345:bool)
                  n1027 = local read "ADrive 11"() -> (w1344:bool)
                  n1028 = local read "ADrive 12"() -> (w1343:bool)
                  n1029 = local read "DDrive 10"() -> (w1341:bool)
                  n1030 = local read "DDrive 11"() -> (w1340:bool)
                  n1031 = local read "DDrive 12"() -> (w1339:bool)
                  n1032 = local read "ADrive 9"() -> (w1346:bool)
                  n1033 = local read "DDrive 9"() -> (w1342:bool)
                  n1034 = Compound Arithmetic op=OR(w1346, w1345, w1344, w1343, w1342, w1341, w1340, w1339, w1338, w1337, w1336, w1335, w1334, w1333, w1332, w1331) -> (w1368:bool)
                  n1035 = Or(x=w1367, y=w1368) -> (x .or. y?=w1369:bool)
                  n1036 = Boolean To (0,1)(Boolean=w1369) -> (0, 1=w1330:i16)
                }
                frame #13 {
                  n1037 = local read "Player1/Player2"() -> (w1380:bool[])
                  n1038 = Index Array(array=w1380) -> (element #1=w1381:bool, element #2=w1382:bool)  [unwired: 2 in]
                  n1039 = Boolean To (0,1)(Boolean=w1382) -> (0, 1=w1370:i16)
                  n1040 = Boolean To (0,1)(Boolean=w1381) -> (0, 1=w1371:i16)
                  n1041 = Compound Arithmetic op=OR("Service1", "Service2", "S1", "S2", "S3", "S4", "S5", "S6") -> (w1392:bool)
                  n1042 = Boolean To (0,1)(Boolean=w1392) -> (0, 1=→"Service":i16)
                  n1043 = Boolean To (0,1)(Boolean="Service1") -> (0, 1=w1379:i16)
                  n1044 = Boolean To (0,1)(Boolean="Service2") -> (0, 1=w1378:i16)
                  n1045 = Boolean To (0,1)(Boolean="S1") -> (0, 1=w1377:i16)
                  n1046 = Boolean To (0,1)(Boolean="S2") -> (0, 1=w1376:i16)
                  n1047 = Boolean To (0,1)(Boolean="S3") -> (0, 1=w1375:i16)
                  n1048 = Boolean To (0,1)(Boolean="S4") -> (0, 1=w1374:i16)
                  n1049 = Boolean To (0,1)(Boolean="S5") -> (0, 1=w1373:i16)
                  n1050 = Boolean To (0,1)(Boolean="S6") -> (0, 1=w1372:i16)
                }
                frame #14 {
                  w1408 = 0 ("disabled index (col)")
                  n1051 = Index Array(array=w1430, index (col) #1=51 ("disabled index (col)"), index (col) #2=52 ("index (col)"), index (col) #3=0 ("index (col)")) -> (element #1=w1419:i64[], element #2=w1418:i64[], element #3=w1421:i64[])  [unwired: 3 in]
                  n1052 = Or(x=w1419, y=w1418) -> (x .or. y?=w1426:i64[])
                  n1053 = Reverse 1D Array(array=w1426) -> (reversed array=w1425:i64[])
                  n1054 = Reverse 1D Array(array=w1421) -> (reversed array=w1423:i64[])
                  n1055 = Compound Arithmetic op=OR("Expected Winner1", "Unexpected Winner1", "Stroke1", "Forced Error2", "Unforced Error2", "Nolet2") -> (w1440:bool)
                  n1056 = Search 1D Array(1D array=w1425, element=i64 1) -> (index of element=w1422:i32)  [unwired: 1 in]
                  n1057 = Boolean To (0,1)(Boolean=w1440) -> (0, 1=w1406:i16)
                  n1058 = Compound Arithmetic op=OR("Expected Winner2", "Unexpected Winner2", "Stroke2", "Forced Error1", "Unforced Error1", "Nolet1") -> (w1439:bool)
                  n1059 = Boolean To (0,1)(Boolean="Expected Winner1") -> (0, 1=w1393:i16)
                  n1060 = Boolean To (0,1)(Boolean="Expected Winner2") -> (0, 1=w1394:i16)
                  n1061 = Boolean To (0,1)(Boolean="Unexpected Winner1") -> (0, 1=w1395:i16)
                  n1062 = Boolean To (0,1)(Boolean="Unexpected Winner2") -> (0, 1=w1396:i16)
                  n1063 = Boolean To (0,1)(Boolean="Stroke1") -> (0, 1=w1397:i16)
                  n1064 = Boolean To (0,1)(Boolean="Stroke2") -> (0, 1=w1398:i16)
                  n1065 = Boolean To (0,1)(Boolean="Forced Error1") -> (0, 1=w1399:i16)
                  n1066 = Boolean To (0,1)(Boolean="Forced Error2") -> (0, 1=w1400:i16)
                  n1067 = Boolean To (0,1)(Boolean="Unforced Error1") -> (0, 1=w1401:i16)
                  n1068 = Boolean To (0,1)(Boolean="Unforced Error2") -> (0, 1=w1402:i16)
                  n1069 = Boolean To (0,1)(Boolean="Nolet1") -> (0, 1=w1403:i16)
                  n1070 = Boolean To (0,1)(Boolean="Nolet2") -> (0, 1=w1404:i16)
                  n1071 = Boolean To (0,1)(Boolean="Let") -> (0, 1=w1405:i16)
                  n1072 = Index Array(array=w1423, index=w1422) -> (element=w1420:i64)
                  n1073 = Boolean To (0,1)(Boolean=w1439) -> (0, 1=w1407:i16)
                  n1074 = Search 1D Array(1D array=w1421, element=w1420) -> (index of element=w1417:i32)  [unwired: 1 in]
                  n1075 = Not Equal To 0?(x=w1406) -> (x != 0?=w1432:bool)
                  n1076 = Not Equal To 0?(x=w1407) -> (x != 0?=w1431:bool)
                  n1077 = Build Array(w1432, w1431) -> (w1409:bool[])
                  n1078 = Index Array(array=w1418, index=w1417) -> (element=w1413:i64)
                  n1079 = Index Array(array=w1419, index=w1417) -> (element=w1414:i64)
                  n1080 = Not Equal To 0?(x=w1414) -> (x != 0?=w1415:bool)
                  n1081 = Not Equal To 0?(x=w1413) -> (x != 0?=w1416:bool)
                  n1082 = Build Array(w1415, w1416) -> (w1410:bool[])
                  n1083 = Select(t=w1410, s="Let", f=w1409) -> (s? t:f=w1412:bool[])
                  n1084 = local write "Score change"(w1412) -> ()
                }
                frame #15 {
                  w1447 = FALSE ("4 6")
                  n1085 = local read "Service"() -> (w1456:i16)
                  n1086 = local read "Cross"() -> (w1455:i16)
                  n1087 = local read "Straight"() -> (w1454:i16)
                  n1088 = local read "position"() -> (w1453:i16)
                  n1089 = local read "Player 1/2"() -> (w1452:i16)
                  n1090 = local read "Extra"() -> (w1451:i16)
                  n1091 = local write "Drop"(w1447) -> ()
                  n1092 = local write "Drop 2"(w1447) -> ()
                  n1093 = local write "Drop 3"(w1447) -> ()
                  n1094 = local write "Drop 4"(w1447) -> ()
                  n1095 = local write "Drop 5"(w1447) -> ()
                  n1096 = local write "Drop 6"(w1447) -> ()
                  n1097 = local write "Drop 7"(w1447) -> ()
                  n1098 = local write "Drop 8"(w1447) -> ()
                  n1099 = local write "Drop 9"(w1447) -> ()
                  n1100 = local write "Drop 10"(w1447) -> ()
                  n1101 = local write "Drop 11"(w1447) -> ()
                  n1102 = local write "Drop 12"(w1447) -> ()
                  n1103 = local write "Chop"(w1447) -> ()
                  n1104 = local write "Chop 2"(w1447) -> ()
                  n1105 = local write "Chop 3"(w1447) -> ()
                  n1106 = local write "Chop 4"(w1447) -> ()
                  n1107 = local write "Chop 5"(w1447) -> ()
                  n1108 = local write "Chop 6"(w1447) -> ()
                  n1109 = local write "Chop 7"(w1447) -> ()
                  n1110 = local write "Chop 8"(w1447) -> ()
                  n1111 = local write "Chop 9"(w1447) -> ()
                  n1112 = local write "Chop 10"(w1447) -> ()
                  n1113 = local write "Chop 11"(w1447) -> ()
                  n1114 = local write "Chop 12"(w1447) -> ()
                  n1115 = Compound Arithmetic op=ADD(w1456, w1455, w1454, w1453, w1452, w1451) -> (w1450:i16)
                  n1116 = Equal To 0?(x=w1450) -> (x = 0?=w1449:bool)
                  n1117 = local write "lob 13"(w1447) -> ()
                  n1118 = local write "lob 2"(w1447) -> ()
                  n1119 = local write "lob 3"(w1447) -> ()
                  n1120 = local write "lob 4"(w1447) -> ()
                  n1121 = local write "lob 5"(w1447) -> ()
                  n1122 = local write "lob 6"(w1447) -> ()
                  n1123 = local write "lob 7"(w1447) -> ()
                  n1124 = local write "lob 8"(w1447) -> ()
                  n1125 = local write "lob 9"(w1447) -> ()
                  n1126 = local write "lob 10"(w1447) -> ()
                  n1127 = local write "lob 11"(w1447) -> ()
                  n1128 = local write "lob 12"(w1447) -> ()
                  n1129 = local write "Smash"(w1447) -> ()
                  n1130 = local write "Smash 2"(w1447) -> ()
                  n1131 = local write "Smash 3"(w1447) -> ()
                  n1132 = local write "Smash 4"(w1447) -> ()
                  n1133 = local write "Smash 5"(w1447) -> ()
                  n1134 = local write "Smash 6"(w1447) -> ()
                  n1135 = local write "Smash 7"(w1447) -> ()
                  n1136 = local write "Smash 8"(w1447) -> ()
                  n1137 = local write "Smash 9"(w1447) -> ()
                  n1138 = local write "Smash 10"(w1447) -> ()
                  n1139 = local write "Smash 11"(w1447) -> ()
                  n1140 = local write "Smash 12"(w1447) -> ()
                  n1141 = case shown="True" "Auto switch" {
                    tunnel: w1449 -> [_ w1457]
                    frame False {
                    }
                    frame True {
                      n1142 = local read "Player1/Player2"() -> (w1463:bool[])
                      n1143 = local read "Player1/Player2"() -> (w1464:bool[])
                      n1144 = Reverse 1D Array(array=w1463) -> (reversed array=w1462:bool[])
                      n1145 = Select(t=w1464, s=w1457, f=w1462) -> (s? t:f=w1458:bool[])
                      n1146 = local read "Score change"() -> (w1460:bool[])
                      n1147 = Or Array Elements(Boolean array=w1460) -> (logical OR=w1461:bool)
                      n1148 = Select(t=w1460, s=w1461, f=w1458) -> (s? t:f=w1459:bool[])
                      n1149 = local write "Player1/Player2"(w1459) -> ()
                    }
                  }
                  n1150 = local write "ADrive"(w1447) -> ()
                  n1151 = local write "ADrive 2"(w1447) -> ()
                  n1152 = local write "ADrive 3"(w1447) -> ()
                  n1153 = local write "ADrive 4"(w1447) -> ()
                  n1154 = local write "ADrive 5"(w1447) -> ()
                  n1155 = local write "ADrive 6"(w1447) -> ()
                  n1156 = local write "ADrive 7"(w1447) -> ()
                  n1157 = local write "ADrive 8"(w1447) -> ()
                  n1158 = local write "ADrive 9"(w1447) -> ()
                  n1159 = local write "ADrive 10"(w1447) -> ()
                  n1160 = local write "ADrive 11"(w1447) -> ()
                  n1161 = local write "ADrive 12"(w1447) -> ()
                  n1162 = local write "DDrive"(w1447) -> ()
                  n1163 = local write "DDrive 2"(w1447) -> ()
                  n1164 = local write "DDrive 3"(w1447) -> ()
                  n1165 = local write "DDrive 4"(w1447) -> ()
                  n1166 = local write "DDrive 5"(w1447) -> ()
                  n1167 = local write "DDrive 6"(w1447) -> ()
                  n1168 = local write "DDrive 7"(w1447) -> ()
                  n1169 = local write "DDrive 8"(w1447) -> ()
                  n1170 = local write "DDrive 9"(w1447) -> ()
                  n1171 = local write "DDrive 10"(w1447) -> ()
                  n1172 = local write "DDrive 11"(w1447) -> ()
                  n1173 = local write "DDrive 12"(w1447) -> ()
                  n1174 = local write "SWADrive"(w1447) -> ()
                  n1175 = local write "SWADrive 2"(w1447) -> ()
                  n1176 = local write "SWADrive 3"(w1447) -> ()
                  n1177 = local write "SWADrive 4"(w1447) -> ()
                  n1178 = local write "SWADrive 5"(w1447) -> ()
                  n1179 = local write "SWADrive 6"(w1447) -> ()
                  n1180 = local write "SWADrive 7"(w1447) -> ()
                  n1181 = local write "SWADrive 8"(w1447) -> ()
                  n1182 = local write "SWADrive 9"(w1447) -> ()
                  n1183 = local write "SWADrive 10"(w1447) -> ()
                  n1184 = local write "SWADrive 11"(w1447) -> ()
                  n1185 = local write "SWADrive 12"(w1447) -> ()
                  n1186 = local write "SWDDrive"(w1447) -> ()
                  n1187 = local write "SWDDrive 2"(w1447) -> ()
                  n1188 = local write "SWDDrive 3"(w1447) -> ()
                  n1189 = local write "SWDDrive 4"(w1447) -> ()
                  n1190 = local write "SWDDrive 5"(w1447) -> ()
                  n1191 = local write "SWDDrive 6"(w1447) -> ()
                  n1192 = local write "SWDDrive 7"(w1447) -> ()
                  n1193 = local write "SWDDrive 8"(w1447) -> ()
                  n1194 = local write "SWDDrive 9"(w1447) -> ()
                  n1195 = local write "SWDDrive 10"(w1447) -> ()
                  n1196 = local write "SWDDrive 11"(w1447) -> ()
                  n1197 = local write "SWDDrive 12"(w1447) -> ()
                  n1198 = local write "Boast"(w1447) -> ()
                  n1199 = local write "Boast 2"(w1447) -> ()
                  n1200 = local write "Boast 3"(w1447) -> ()
                  n1201 = local write "Boast 4"(w1447) -> ()
                  n1202 = local write "Boast 5"(w1447) -> ()
                  n1203 = local write "Boast 6"(w1447) -> ()
                  n1204 = local write "Boast 7"(w1447) -> ()
                  n1205 = local write "Boast 8"(w1447) -> ()
                  n1206 = local write "Boast 9"(w1447) -> ()
                  n1207 = local write "Boast 10"(w1447) -> ()
                  n1208 = local write "Boast 11"(w1447) -> ()
                  n1209 = local write "Boast 12"(w1447) -> ()
                  n1210 = local write "4 4"(w1447) -> ()
                  n1211 = local write "4 3"(w1447) -> ()
                  n1212 = local write "4 2"(w1447) -> ()
                  n1213 = local write "4 1"(w1447) -> ()
                  n1214 = local write "3 4"(w1447) -> ()
                  n1215 = local write "3 3"(w1447) -> ()
                  n1216 = local write "3 2"(w1447) -> ()
                  n1217 = local write "3 1"(w1447) -> ()
                  n1218 = local write "2 4"(w1447) -> ()
                  n1219 = local write "2 3"(w1447) -> ()
                  n1220 = local write "2 2"(w1447) -> ()
                  n1221 = local write "2 1"(w1447) -> ()
                  n1222 = local write "1 4"(w1447) -> ()
                  n1223 = local write "1 3"(w1447) -> ()
                  n1224 = local write "1 2"(w1447) -> ()
                  n1225 = local write "1 1"(w1447) -> ()
                  n1226 = local write "5 4"(w1447) -> ()
                  n1227 = local write "5 3"(w1447) -> ()
                  n1228 = local write "5 2"(w1447) -> ()
                  n1229 = local write "5 1"(w1447) -> ()
                  n1230 = local write "6 4"(w1447) -> ()
                  n1231 = local write "6 3"(w1447) -> ()
                  n1232 = local write "6 2"(w1447) -> ()
                  n1233 = local write "6 1"(w1447) -> ()
                  n1234 = local write "S6"(w1447) -> ()
                  n1235 = local write "S5"(w1447) -> ()
                  n1236 = local write "S4"(w1447) -> ()
                  n1237 = local write "S1"(w1447) -> ()
                  n1238 = local write "S2"(w1447) -> ()
                  n1239 = local write "S3"(w1447) -> ()
                  n1240 = local write "Let"(w1447) -> ()
                  n1241 = local write "Unexpected Winner2"(w1447) -> ()
                  n1242 = local write "Unexpected Winner1"(w1447) -> ()
                  n1243 = local write "Expected Winner2"(w1447) -> ()
                  n1244 = local write "Expected Winner1"(w1447) -> ()
                  n1245 = local write "Forced Error2"(w1447) -> ()
                  n1246 = local write "Forced Error1"(w1447) -> ()
                  n1247 = local write "Service2"(w1447) -> ()
                  n1248 = local write "Service1"(w1447) -> ()
                  n1249 = local write "Nolet2"(w1447) -> ()
                  n1250 = local write "Nolet1"(w1447) -> ()
                  n1251 = local write "Stroke2"(w1447) -> ()
                  n1252 = local write "Stroke1"(w1447) -> ()
                  n1253 = local write "Unforced Error2"(w1447) -> ()
                  n1254 = local write "Unforced Error1"(w1447) -> ()
                  n1255 = local write "Player1"(w1447) -> ()
                  n1256 = local write "Player2"(w1447) -> ()
                  n1257 = local write "Button 5"(w1447) -> ()
                  n1258 = local write "Button 4"(w1447) -> ()
                  n1259 = local write "Button 3"(w1447) -> ()
                  n1260 = local write "Button 2"(w1447) -> ()
                  n1261 = local write "Button 1"(w1447) -> ()
                }
              }
              n1262 = Build Array(w605, w734, w733, w732, w731, w730, w729, w728, w727, w726, w725, w724, w723, w722, w721, w720, w719, w718, w717, w716, w715, w714, w713, w712, w711, w710, w709, w708, w707, w706, w705, w704, w703, w702, w701, w700, w699, w698, w697, w696, w695, w694, w693, w692, w691, w690, w689, w678, w677, w676, w675, w688, w687, w686, w685, w684, w683, w682, w681, w680, w679, w631, w630, w629, w628, w627, w618, w617, w616, w615, w614, w613, w612, w611, w610, w619) -> (w599:u32[])
              n1263 = call "IMAQ Dispose"("Image"=w735) -> ()  [unwired: 5 in, 1 out]
              n1264 = Index Array(array=w601, index (col)=0 ("disabled index (col)")) -> (element=w743:i64[])  [unwired: 1 in]
              n1265 = Delete From Array(array=w599, index=0) -> (array with subset deleted=w659:u32[])  [unwired: 1 in, 1 out]
              n1266 = for {
                tunnel: w743 -> [w761] mode=indexing
                tunnel: w605 -> [w762]
                tunnel: [w761] -> w741 mode=indexing if=w763
                stop <- w763 continue-if-true
                n1267 = Less Or Equal?(x=w761, y=w762) -> (x <= y?=w763:bool)
              }
              n1268 = Delete From Array(array=w659, length=2, index=68) -> (array with subset deleted=w587:u32[])  [unwired: 1 out]
              n1269 = Array Size(array=w741) -> (size(s)=w600:i32)
              n1270 = Delete From Array(array=w587, length=17, index=43) -> (deleted portion=w653:u32[], array with subset deleted=w657:u32[])
              n1271 = Delete From Array(array=w587, length=2, index=0) -> (array with subset deleted=w584:u32[])  [unwired: 1 out]
              n1272 = Decrement(x=w600) -> (x-1=w651:i32)
              n1273 = Array Max & Min(array=w657) -> (max value=w658:u32)  [unwired: 3 out]
              n1274 = Array Max & Min(array=w653) -> (max value=w660:u32)  [unwired: 3 out]
              n1275 = Equal To 0?(x=w658) -> ()  [unwired: 1 out]
              n1276 = Not Equal To 0?(x=w660) -> (x != 0?=w656:bool)
              n1277 = Index Array(array=w601, index (row)=w651) -> (element=w654:i64[])  [unwired: 1 in]
              n1278 = Array Max & Min(array=w584) -> (max value=w737:u32)  [unwired: 3 out]
              n1279 = Compound Arithmetic op=AND(w646, w656, "Link Errors") -> (w602:bool)
              n1280 = Decrement(x=w600) -> (x-1=w647:i32)
              n1281 = Replace Array Subset(array=w654, new element=w653, index=44) -> (w598:i64[])
              n1282 = Equal To 0?(x=w737) -> (x = 0?=w590:bool)
              n1283 = Index Array(array=w598, index=w597) -> (element=w596:i64)
              n1284 = Replace Array Subset(array=w601, new element=w598, index (row)=w647) -> (w650:i64[][])  [unwired: 1 in]
              n1285 = Insert Into Array(array=w601, index (row)=w600, new element=w599) -> (w649:i64[][])  [unwired: 1 in]
              n1286 = Index Array(array=w599, index=w597) -> (element=w595:u32)
              n1287 = Select(t=w650, s=w602, f=w649) -> (s? t:f=w648:i64[][])
              n1288 = Select(t=w596, s=w602, f=w595) -> (s? t:f=w588:i64)
              n1289 = local read "last saved data"() -> (w593:i64[])
              n1290 = Select(t=w601, s=w590, f=w648) -> (s? t:f=w604:i64[][])
              n1291 = Search 1D Array(1D array=w593, element=w588) -> (index of element=w592:i32)  [unwired: 1 in]
              n1292 = Greater Than 0?(x=w592) -> (x > 0?=w591:bool)
              n1293 = Insert Into Array(array=w593, new element=w588) -> (w594:i64[])  [unwired: 1 in]
              n1294 = Or(x=w591, y=w590) -> (x .or. y?=w589:bool)
              n1295 = Select(t=w593, s=w589, f=w594) -> (s? t:f=w582:i64[])
              n1296 = case shown="True" "Undo" {
                tunnel: w604 -> [w745 w747]
                tunnel: [w745 w746] -> w603
                tunnel: w582 -> [w744 w756]
                tunnel: [w744 w749] -> w583
                frame False {
                }
                frame True {
                  n1297 = Reverse 1D Array(array=w756) -> (reversed array=w755:i64[])
                  n1298 = Delete From Array(array=w755, index=0) -> (deleted portion=w751:i64, array with subset deleted=w750:i64[])  [unwired: 1 in]
                  n1299 = Reverse 1D Array(array=w750) -> (reversed array=w749:i64[])
                  n1300 = Index Array(array=w747, index (col)=0 ("disabled index (col)")) -> (element=w752:i64[])  [unwired: 1 in]
                  n1301 = Search 1D Array(1D array=w752, element=w751) -> (index of element=w748:i32)  [unwired: 1 in]
                  n1302 = local write "Undo"(FALSE ("Undo")) -> ()
                  n1303 = Delete From Array(array=w747, index (row)=w748) -> (array with subset deleted=w746:i64[][])  [unwired: 2 in, 1 out]
                }
              }
              "last saved data" <- w583
              n1304 = Concatenate Strings("Btn 1", w607, "Btn 2", w607, "Btn 3", w607, "Btn 4", w607, "Btn 5", w607, "Error" ("String")) -> (w621:string)
              n1305 = for {
                tunnel: string[] ["frame number", "Lead", "Lag", "position 1", "position 2", "position 3", "position 4", "position 5", "position 6", "position 7", "position 8", "position 9", "position 10", "position 11", "position 12", "position 13", "position 14", "position 15", "position 16", "position 17", "position 18", "position 19", "position 20", "position 21", "position 22", "position 23", "position 24", "Drive A", "Drive D", "SW Drive A", "SW Drive D", "drop", "chop", "lob", "boast 2", "boast 3", "smash", "Forehand", "Backhand", "Straight", "Cross", "Bounce", "Half Volley", "Volley", "Expected winner 1", "Expected winner 2", "Unexpected winner 1", "Unexpected winner 2", "Stroke 1", "Stroke 2", "Forced error 1", "Forced error 2", "Unforced error 1", "Unforced error 2", "No let 1", "No let 2", "Let", "point1", "point2", "score1", "score2", "service1", "service2", "s1", "s2", "s3", "s4", "s5", "s6", "player1", "player2"] ("all rows") -> [w760] mode=indexing
                tunnel: [w758] -> w608 mode=indexing
                n1306 = Concatenate Strings(w760, "\t") -> (w758:string)
              }
              n1307 = Index Array(array=w603, index (col)=0 ("disabled index (col)")) -> (element=w672:i64[])  [unwired: 1 in]
              n1308 = local read "Video file"() -> (w640:path)
              n1309 = Index Array(array=w603, index (col) #1=57 ("disabled index (col)"), index (col) #2=58 ("index (col)")) -> (element #1=w668:i64[], element #2=w665:i64[])  [unwired: 2 in]
              n1310 = local read "Data file"() -> (w634:path)
              n1311 = Array Max & Min(array=w672) -> (max index (indices)=w673:i32)  [unwired: 3 out]
              n1312 = Add Array Elements(numeric array=w668) -> (sum=→"P1":i64)
              n1313 = Add Array Elements(numeric array=w665) -> (sum=→"P2":i64)
              n1314 = call <vilib>:"Get File Extension.vi"("file"=w640) -> ("filename without extension"=w642:string)  [unwired: 7 in, 3 out]
              n1315 = Open/Create/Replace File(file path (use dialog)=w634, operation (0:open)=T3."replace") -> (refnum out=w636:refnum<file>, error out=w635:errorcluster)  [unwired: 4 in, 1 out]
              n1316 = Index Array(array=w603, index (row)=w673) -> (element=→"last row":i64[])  [unwired: 1 in]
              n1317 = Concatenate Strings(w608, w621, "\r") -> (w633:string)
              n1318 = Array To Spreadsheet String(delimiter (Tab)="\t" ("delimiter (\\t)"), array=w603, 3:"%.3f" ("format (%.3f)")) -> (spreadsheet string=w645:string)
              n1319 = Concatenate Strings("avi file" ("string"), w643, w642, w643, w643, w633, w645) -> (w644:string)
              n1320 = Write to Text File(file (use dialog)=w636, text=w644, error in=w635) -> (refnum out=w632:refnum<file>)  [unwired: 1 in, 2 out]
            }
          }
          "coding" <- w576
        }
        frame "Display" {
          n1321 = flat-sequence {
            tunnel: [w1520] -> w1485
            tunnel: w1482 -> [w1521]
            tunnel: w1485 -> [w1528]
            tunnel: [w1527] -> w1481
            tunnel: [w1526] -> w1479
            tunnel: [w1525] -> w1478
            tunnel: w1481 -> [w1587]
            tunnel: [w1587] -> w1480
            tunnel: w1479 -> [w1585]
            tunnel: w1478 -> [w1586]
            tunnel: [w1586] -> w1477
            tunnel: [w1585] -> w1476
            tunnel: [w1629] -> w1484
            tunnel: w1480 -> [w1630]
            tunnel: w1477 -> [w1629]
            tunnel: w1476 -> [w1628]
            tunnel: [w1628] -> w1475
            tunnel: [w1628] -> w1474
            tunnel: w1484 -> [w1690]
            tunnel: [w1690] -> w1483
            tunnel: w1475 -> [_]
            tunnel: w1474 -> [w1679]
            tunnel: [w1679] -> w1473
            tunnel: w1483 -> [w1703]
            tunnel: w1473 -> [w1700]
            frame #0 {
              n1322 = case shown="\"2\"" "display\nselection" {
                tunnel: [w1523 w1524] -> w1520
                tunnel: w1521 -> [w1523 _]
                frame "1", Default {
                }
                frame "2" {
                  n1323 = local read "Edited data"() -> (w1524:i64[][])
                }
              }
            }
            frame #1 {
              w1537 = 64
              # "disreagard player on display option to be set here"
              # "ADD elements on one column to get the data"
              # "extract seperate data sets for player 1 and player 2"
              n1324 = Index Array(array=w1528, index (col)=69 ("index")) -> (element=w1530:i64[])  [unwired: 1 in]
              n1325 = Index Array(array=w1528, index (col)=70 ("index")) -> (element=w1533:i64[])  [unwired: 1 in]
              n1326 = for {
                tunnel: w1528 -> [w1566]
                tunnel: w1530 -> [w1568] mode=indexing
                shift-right: [w1561] -> w1535
                shift-left: i64[][] [] ("Combined data") -> [w1562]
                i -> [w1565]
                n1327 = Index Array(array=w1566, index (row)=w1565) -> (element=w1564:i64[])  [unwired: 1 in]
                n1328 = Not Equal To 0?(x=w1568) -> (x != 0?=w1567:bool)
                n1329 = Insert Into Array(array=w1562, new element=w1564) -> (w1563:i64[][])  [unwired: 2 in]
                n1330 = Select(t=w1563, s=w1567, f=w1562) -> (s? t:f=w1561:i64[][])
              }
              n1331 = for {
                tunnel: w1528 -> [w1558]
                tunnel: w1533 -> [w1560] mode=indexing
                shift-right: [w1553] -> w1536
                shift-left: i64[][] [] ("Combined data") -> [w1554]
                i -> [w1557]
                n1332 = Index Array(array=w1558, index (row)=w1557) -> (element=w1556:i64[])  [unwired: 1 in]
                n1333 = Not Equal To 0?(x=w1560) -> (x != 0?=w1559:bool)
                n1334 = Insert Into Array(array=w1554, new element=w1556) -> (w1555:i64[][])  [unwired: 2 in]
                n1335 = Select(t=w1555, s=w1559, f=w1554) -> (s? t:f=w1553:i64[][])
              }
              n1336 = for {
                N: w1537 -> [_]
                tunnel: w1536 -> [w1546]
                tunnel: [w1543] -> w1526 mode=indexing
                i -> [w1547]
                n1337 = Increment(x=w1547) -> (x+1=w1545:i32)
                n1338 = Index Array(array=w1546, index (col)=w1545) -> (element=w1544:i64[])  [unwired: 1 in]
                n1339 = Add Array Elements(numeric array=w1544) -> (sum=w1543:i64)
              }
              "Player 2 data" <- w1526
              n1340 = for {
                N: w1537 -> [_]
                tunnel: w1535 -> [w1551]
                tunnel: [w1548] -> w1525 mode=indexing
                i -> [w1552]
                n1341 = Increment(x=w1552) -> (x+1=w1550:i32)
                n1342 = Index Array(array=w1551, index (col)=w1550) -> (element=w1549:i64[])  [unwired: 1 in]
                n1343 = Add Array Elements(numeric array=w1549) -> (sum=w1548:i64)
              }
              "player 1 data" <- w1525
              n1344 = for {
                N: w1537 -> [_]
                tunnel: w1528 -> [w1541]
                tunnel: [w1538] -> w1527 mode=indexing
                i -> [w1542]
                n1345 = Increment(x=w1542) -> (x+1=w1540:i32)
                n1346 = Index Array(array=w1541, index (col)=w1540) -> (element=w1539:i64[])  [unwired: 1 in]
                n1347 = Add Array Elements(numeric array=w1539) -> (sum=w1538:i64)
              }
              "both player data" <- w1527
            }
            frame #2 {
              # "Position numbers"
              n1348 = Array Subset(array=w1586, index=2, length=26) -> (w1623:i64[])
              n1349 = Index Array(array=w1623) -> (element #1=→"1 13":i64, element #2=→"1 14":i64, element #3=→"1 11":i64, element #4=→"1 9":i64, element #5=→"2 14":i64, element #6=→"2 13":i64, element #7=→"2 11":i64, element #8=→"2 9":i64, element #9=→"3 13":i64, element #10=→"3 11":i64, element #11=→"3 10":i64, element #12=→"3 8":i64, element #13=→"4 13":i64, element #14=→"4 11":i64, element #15=→"4 10":i64, element #16=→"4 8":i64, element #17=→"5 17":i64, element #18=→"5 16":i64, element #19=→"5 15":i64, element #20=→"5 18":i64, element #21=→"6 21":i64, element #22=→"6 20":i64, element #23=→"6 19":i64, element #24=→"6 18":i64)  [unwired: 24 in]
              n1350 = Array Subset(array=w1585, index=2, length=26) -> (w1606:i64[])
              n1351 = Index Array(array=w1606) -> (element #1=→"1 12":i64, element #2=→"1 22":i64, element #3=→"1 32":i64, element #4=→"1 42":i64, element #5=→"2 12":i64, element #6=→"2 22":i64, element #7=→"2 32":i64, element #8=→"2 42":i64, element #9=→"3 12":i64, element #10=→"3 22":i64, element #11=→"3 32":i64, element #12=→"3 42":i64, element #13=→"4 12":i64, element #14=→"4 22":i64, element #15=→"4 32":i64, element #16=→"4 42":i64, element #17=→"5 14":i64, element #18=→"5 23":i64, element #19=→"5 33":i64, element #20=→"5 43":i64, element #21=→"6 15":i64, element #22=→"6 24":i64, element #23=→"6 34":i64, element #24=→"6 44":i64)  [unwired: 24 in]
            }
            frame #3 {
              # "winner error numbers"
              # "Shot numbers"
              n1352 = Array Subset(array=w1628, index=26, length=10) -> (w1647:i64[])
              n1353 = Index Array(array=w1628, index=55) -> (element=w1637:i64)
              n1354 = Index Array(array=w1629, index=55) -> (element=w1634:i64)
              n1355 = Array Subset(array=w1629, index=26, length=10) -> (w1648:i64[])
              n1356 = Number To Fractional String(number=w1647, precision (6)=i16 0) -> (F-format string=w1662:string[])  [unwired: 2 in]
              n1357 = Array Subset(array=w1630, index=43, length=12) -> (w1654:i64[])
              n1358 = Number To Fractional String(number=w1637, precision (6)=i16 0) -> (F-format string=→"Let 4":string)  [unwired: 2 in]
              n1359 = Number To Fractional String(number=w1648, precision (6)=i16 0) -> (F-format string=w1663:string[])  [unwired: 2 in]
              n1360 = Number To Fractional String(number=w1634, precision (6)=i16 0) -> (F-format string=→"Let 3":string)  [unwired: 2 in]
              n1361 = Insert Into Array(array=w1662, index=4, new element="" ("new element/subarray")) -> (→"Player 2 shots numbers":string[])
              n1362 = Number To Fractional String(number=w1654, precision (6)=i16 0) -> (F-format string=w1653:string[])  [unwired: 2 in]
              n1363 = Insert Into Array(array=w1663, index=4, new element="" ("new element/subarray")) -> (→"Player 1 shots numbers":string[])
              n1364 = Index Array(array=w1653) -> (element #1=→"ex win1 num":string, element #2=→"ex win2 num":string, element #3=→"UNex win1 num":string, element #4=→"UNex win2 num":string, element #5=→"Stroke 3":string, element #6=→"Stroke 4":string, element #7=→"F err1 num":string, element #8=→"F err2 num":string, element #9=→"UF err1 num":string, element #10=→"UF err2 num":string, element #11=→"No Let 1":string, element #12=→"No Let 2":string)  [unwired: 12 in]
            }
            frame #4 {
              n1365 = Array Subset(array=w1690, index=36, length=7) -> (w1692:i64[])
              n1366 = Array Subset(array=w1679, index=36, length=7) -> (w1683:i64[])
              n1367 = Number To Fractional String(number=w1692, precision (6)=i16 0) -> (F-format string=w1691:string[])  [unwired: 2 in]
              n1368 = Number To Fractional String(number=w1683, precision (6)=i16 0) -> (F-format string=w1684:string[])  [unwired: 2 in]
              n1369 = Index Array(array=w1691) -> (element #1=→"F-hand 1":string, element #2=→"B-hand 1":string, element #3=→"Straight 1":string, element #4=→"Cross 1":string, element #5=→"Bounce 1":string, element #6=→"H-volley 1":string, element #7=→"Volley 1":string)  [unwired: 7 in]
              n1370 = Index Array(array=w1684) -> (element #1=→"F-hand 2":string, element #2=→"B-hand 2":string, element #3=→"Straight 3":string, element #4=→"Cross 3":string, element #5=→"Bounce 3":string, element #6=→"H-volley 3":string, element #7=→"Volley 3":string)  [unwired: 7 in]
            }
            frame #5 {
              # "slider sclaes for graphical display"
              n1371 = Array Subset(array=w1703, index=26, length=10) -> (w1699:i64[])
              "subarray" <- w1699
              n1372 = Array Subset(array=w1700, index=26, length=10) -> (w1698:i64[])
              n1373 = Insert Into Array(array=w1699, new element=w1698) -> (w1697:i64[])  [unwired: 1 in]
              n1374 = Array Max & Min(array=w1698) -> (max value=w1707:i64)  [unwired: 3 out]
              n1375 = Equal To 0?(x=w1707) -> (x = 0?=w1706:bool)
              n1376 = Array Max & Min(array=w1697) -> (max value=w1711:i64)  [unwired: 3 out]
              n1377 = Select(t=1.0, s=w1706, f=w1707) -> ()  [unwired: 1 out]
              n1378 = Equal To 0?(x=w1711) -> (x = 0?=w1710:bool)
              n1379 = Select(t=1.0, s=w1710, f=w1711) -> (s? t:f=w1696:dbl)
              n1380 = property on="FH 2" class="Slide (strict)"("Scale.Maximum"=w1696) -> ()  [unwired: 2 in, 2 out]
              n1381 = property on="BH 2" class="Slide (strict)"("Scale.Maximum"=w1696) -> ()  [unwired: 2 in, 2 out]
              n1382 = property on="Straight 2" class="Slide (strict)"("Scale.Maximum"=w1696) -> ()  [unwired: 2 in, 2 out]
              n1383 = property on="Cross 2" class="Slide (strict)"("Scale.Maximum"=w1696) -> ()  [unwired: 2 in, 2 out]
              n1384 = property on="Bounce 2" class="Slide (strict)"("Scale.Maximum"=w1696) -> ()  [unwired: 2 in, 2 out]
              n1385 = property on="Volley 2" class="Slide (strict)"("Scale.Maximum"=w1696) -> ()  [unwired: 2 in, 2 out]
              n1386 = property on="Drive 2" class="Slide (strict)"("Scale.Maximum"=w1696) -> ()  [unwired: 2 in, 2 out]
              n1387 = property on="Drop 13" class="Slide (strict)"("Scale.Maximum"=w1696) -> ()  [unwired: 2 in, 2 out]
              n1388 = property on="Lob 2" class="Slide (strict)"("Scale.Maximum"=w1696) -> ()  [unwired: 2 in, 2 out]
              n1389 = property on="Boast 13" class="Slide (strict)"("Scale.Maximum"=w1696) -> ()  [unwired: 2 in, 2 out]
              n1390 = property on="Drive 1" class="Slide (strict)"("Scale.Maximum"=w1696) -> ()  [unwired: 2 in, 2 out]
              n1391 = property on="Drop 1" class="Slide (strict)"("Scale.Maximum"=w1696) -> ()  [unwired: 2 in, 2 out]
              n1392 = property on="Lob 1" class="Slide (strict)"("Scale.Maximum"=w1696) -> ()  [unwired: 2 in, 2 out]
              n1393 = property on="Boast 1" class="Slide (strict)"("Scale.Maximum"=w1696) -> ()  [unwired: 2 in, 2 out]
              n1394 = property on="FH 1" class="Slide (strict)"("Scale.Maximum"=w1696) -> ()  [unwired: 2 in, 2 out]
              n1395 = property on="BH 1" class="Slide (strict)"("Scale.Maximum"=w1696) -> ()  [unwired: 2 in, 2 out]
              n1396 = property on="Straight 4" class="Slide (strict)"("Scale.Maximum"=w1696) -> ()  [unwired: 2 in, 2 out]
              n1397 = property on="Cross 4" class="Slide (strict)"("Scale.Maximum"=w1696) -> ()  [unwired: 2 in, 2 out]
              n1398 = property on="Bounce 4" class="Slide (strict)"("Scale.Maximum"=w1696) -> ()  [unwired: 2 in, 2 out]
              n1399 = property on="Volley 4" class="Slide (strict)"("Scale.Maximum"=w1696) -> ()  [unwired: 2 in, 2 out]
              n1400 = Index Array(array=w1698) -> (element #1=→"Drive 2":i64, element #2=→"Drop 13":i64, element #3=→"Lob 2":i64, element #4=→"Boast 13":i64, element #5=→"FH 2":i64, element #6=→"BH 2":i64, element #7=→"Straight 2":i64, element #8=→"Cross 2":i64, element #9=→"Bounce 2":i64, element #10=→"Volley 2":i64)  [unwired: 10 in]
              n1401 = Index Array(array=w1699) -> (element #1=→"Drive 1":i64, element #2=→"Drop 1":i64, element #3=→"Lob 1":i64, element #4=→"Boast 1":i64, element #5=→"FH 1":i64, element #6=→"BH 1":i64, element #7=→"Straight 4":i64, element #8=→"Cross 4":i64, element #9=→"Bounce 4":i64, element #10=→"Volley 4":i64)  [unwired: 10 in]
            }
          }
          n1402 = local read "Video files to write"() -> (w1469:string[])
          n1403 = property on="Video files to write" class="Arr (strict)"() -> ("Index Values"=w1468:u32[])  [unwired: 2 in, 2 out]
          n1404 = local read "frames to write"() -> (w1470:i64[][])
          n1405 = case shown="True" "Upload edited video" {
            frame False {
            }
            frame True {
              n1406 = flat-sequence {
                frame #0 {
                  n1407 = local read "frames edited"() -> (w1516:i64[])
                  n1408 = local write "Progress..."(u32 0 ("Progress...")) -> ()
                  n1409 = local write "frames 2 play"(w1516) -> ()
                }
                frame #1 {
                  w1518 = FALSE ("stop")
                  w1519 = TRUE ("Play")
                  n1410 = local write "Load video"(w1519) -> ()
                  n1411 = local write "Play"(w1519) -> ()
                  n1412 = local write "stop"(w1518) -> ()
                  n1413 = local write "Upload edited video"(w1518) -> ()
                  n1414 = local write "Pause"(w1518) -> ()
                }
              }
            }
          }
          n1415 = Index Array(array=w1468) -> (element=w1465:u32)  [unwired: 1 in]
          n1416 = And Array Elements(Boolean array="Delete") -> (logical AND=w1467:bool)
          n1417 = case shown="True" "Add to lib" {
            tunnel: w1470 -> [_ w1511]
            tunnel: w1469 -> [_ w1508]
            frame False {
            }
            frame True {
              n1418 = local read "frames edited"() -> (w1507:i64[])
              n1419 = local write "Add to lib"(FALSE ("Add to lib")) -> ()
              n1420 = Build Array("File name") -> (w1509:string[])
              n1421 = Build Array(w1507) -> (w1512:i64[][])
              n1422 = Insert Into Array(array=w1512, new element=w1511) -> (→"frames to write":i64[][])  [unwired: 2 in]
              n1423 = Insert Into Array(array=w1509, new element=w1508) -> (→"Video files to write":string[])  [unwired: 1 in]
            }
          }
          n1424 = case shown="False" w1467 {
            tunnel: "Delete" -> [w1503 _]
            tunnel: w1465 -> [w1501 _]
            frame False {
              n1425 = for {
                tunnel: w1503 -> [w1506] mode=indexing
                tunnel: [w1504] -> w1502
                i -> [w1504]
                stop <- w1505 stop-if-true
                n1426 = Not(x=w1506) -> (.not. x?=w1505:bool)
              }
              n1427 = local write "Delete"(bool[] [TRUE, TRUE, TRUE, TRUE, TRUE] ("Array 2")) -> ()
              n1428 = local read "Video files to write"() -> (w1498:string[])
              n1429 = local read "frames to write"() -> (w1496:i64[][])
              n1430 = Add(x=w1502, y=w1501) -> (x+y=w1495:u32)
              n1431 = Delete From Array(array=w1498, index=w1495) -> (array with subset deleted=w1500:string[])  [unwired: 1 in, 1 out]
              n1432 = Delete From Array(array=w1496, index (row)=w1495) -> (array with subset deleted=w1497:i64[][])  [unwired: 2 in, 1 out]
              n1433 = local write "frames to write"(w1497) -> ()
              n1434 = local write "Video files to write"(w1500) -> ()
            }
            frame True {
            }
          }
          n1435 = local read "refnum of data save file"() -> (w1487:refnum<file>)
          n1436 = local write "Code number display"(1 ("Code number")) -> ()
          n1437 = Select(t=T1."Edit video" ("Main tab"), s="Extract data", f=T1."Display" ("Main tab")) -> (s? t:f=w1493:T1)
          n1438 = Select(t=T1."Examine coding" ("Main tab"), s="Examine code", f=w1493) -> (s? t:f=w1494:T1)
        }
        frame "Edit video" {
          w1753 = T4."Disabled and Grayed Out" ("Disabled")
          n1439 = local read "Btn 5"() -> (w1736:string)
          "Btn 10" <- w1736
          n1440 = local read "Btn 4"() -> (w1735:string)
          "Btn 9" <- w1735
          n1441 = local read "Btn 3"() -> (w1734:string)
          "Btn 8" <- w1734
          n1442 = local read "Btn 2"() -> (w1733:string)
          "Btn 7" <- w1733
          n1443 = local read "Btn 1"() -> (w1732:string)
          "Btn 6" <- w1732
          n1444 = property on="Button 10" class="Bool (strict)"("BoolText.Text"=w1736) -> ()  [unwired: 2 in, 2 out]
          n1445 = property on="Button 9" class="Bool (strict)"("BoolText.Text"=w1735) -> ()  [unwired: 2 in, 2 out]
          n1446 = property on="Button 8" class="Bool (strict)"("BoolText.Text"=w1734) -> ()  [unwired: 2 in, 2 out]
          n1447 = property on="Button 7" class="Bool (strict)"("BoolText.Text"=w1733) -> ()  [unwired: 2 in, 2 out]
          n1448 = property on="Button 6" class="Bool (strict)"("BoolText.Text"=w1732) -> ()  [unwired: 2 in, 2 out]
          n1449 = Array Size(array=w1740) -> (size(s)=w1741:i32[])
          n1450 = Index Array(array=w1741) -> (element #2=w1739:i32)  [unwired: 2 in, 1 out]
          n1451 = Initialize Array(i64 0 ("element"), w1739) -> (w1738:i64[])
          n1452 = local write "Extract data"(FALSE ("edit video")) -> ()
          n1453 = Build Array(w1738) -> (w1737:i64[][])
          n1454 = property on="Code number display" class="DigNum (strict)"("DisabledEnum"=w1753) -> ()  [unwired: 2 in, 2 out]
          n1455 = property on="Next" class="Bool (strict)"("DisabledEnum"=w1753) -> ()  [unwired: 2 in, 2 out]
          n1456 = property on="Reset" class="Bool (strict)"("DisabledEnum"=w1753) -> ()  [unwired: 2 in, 2 out]
          n1457 = property on="Update" class="Bool (strict)"("DisabledEnum"=w1753) -> ()  [unwired: 2 in, 2 out]
          n1458 = property on="Previous" class="Bool (strict)"("DisabledEnum"=w1753) -> ()  [unwired: 2 in, 2 out]
          n1459 = flat-sequence {
            tunnel: [w1772] -> w1743
            tunnel: [w1771] -> w1744
            tunnel: [w1770] -> w1745
            tunnel: [w1769] -> w1746
            tunnel: [w1768] -> w1747
            tunnel: [w1767] -> w1748
            tunnel: [w1766] -> w1749
            tunnel: [w1765] -> w1750
            tunnel: [w1764] -> w1751
            tunnel: [w1760] -> w1752
            tunnel: w1740 -> [w1758]
            tunnel: w1737 -> [w1757]
            tunnel: w1752 -> [w1851]
            tunnel: w1751 -> [w1852]
            tunnel: w1750 -> [w1853]
            tunnel: w1749 -> [w1861]
            tunnel: w1748 -> [w1862]
            tunnel: w1747 -> [w1871]
            tunnel: w1746 -> [w1872]
            tunnel: w1745 -> [w1873]
            tunnel: w1744 -> [w1881]
            tunnel: w1743 -> [w1904]
            frame #0 {
              # "seperate sections of data"
              n1460 = Insert Into Array(array=w1757, new element=w1758) -> (w1759:i64[][])  [unwired: 2 in]
              "Combined data" <- w1759
              n1461 = Array Size(array=w1759) -> (size(s)=w1763:i32[])
              n1462 = Index Array(array=w1763) -> (element=w1762:i32)  [unwired: 1 in]
              n1463 = Initialize Array(i64 0 ("element"), w1762) -> (w1760:i64[])
              n1464 = Array Subset(array=w1759, index (col)=3 ("index"), length (col)=24 ("length")) -> (w1772:i64[][])  [unwired: 2 in]
              n1465 = Array Subset(array=w1759, index (col)=27 ("index"), length (col)=10 ("length")) -> (w1771:i64[][])  [unwired: 2 in]
              n1466 = Array Subset(array=w1759, index (col)=37 ("index"), length (col)=2 ("length")) -> (w1770:i64[][])  [unwired: 2 in]
              n1467 = Array Subset(array=w1759, index (col)=39 ("index"), length (col)=2 ("length")) -> (w1769:i64[][])  [unwired: 2 in]
              n1468 = Array Subset(array=w1759, index (col)=41 ("index"), length (col)=3 ("length")) -> (w1768:i64[][])  [unwired: 2 in]
              n1469 = Array Subset(array=w1759, index (col)=44 ("index"), length (col)=13 ("length")) -> (w1767:i64[][])  [unwired: 2 in]
              n1470 = Array Subset(array=w1759, index (col)=61 ("index"), length (col)=8 ("length")) -> (w1766:i64[][])  [unwired: 2 in]
              n1471 = Array Subset(array=w1759, index (col)=69 ("index"), length (col)=2 ("length")) -> (w1765:i64[][])  [unwired: 2 in]
              n1472 = Array Subset(array=w1759, index (col)=71 ("index"), length (col)=5 ("length")) -> (w1764:i64[][])  [unwired: 2 in]
            }
            frame #1 {
              w1934 = i64[][] [] ("Combined data")
              # "AND different sections of data"
              # "needs data to display for\n\nfull match (combined data)\nedited section\n1 shot b4\n1shot after"
              # "display which data selector needs to be set here"
              # "extract select events ONLY from full data"
              # "delete negative frames\nand frames past last frame of video"
              # "delete repeated frames"
              n1473 = Build Array("Adrive", "Ddrive", "ASWdrive", "DSWdrive", "Drop 14", "Chop 13", "Lob", "Boast2", "Boast3", "Smash 13") -> (w1831:bool[])
              n1474 = Build Array("1 10", "1 7", "1 6", "1 5", "2 10", "2 7", "2 6", "2 5", "3 9", "3 7", "3 6", "3 5", "4 9", "4 7", "4 6", "4 5", "5 8", "5 7", "5 6", "5 5", "6 8", "6 7", "6 6", "6 5") -> (w1832:bool[])
              n1475 = call "or multiple inputs.vi"("zero array in"=w1851, "input array in"=w1831, "file data in"=w1881) -> ("array out"=w1848:dbl[], "no input?"=w1833:bool)
              n1476 = call "or multiple inputs.vi"("zero array in"=w1851, "input array in"=w1832, "file data in"=w1904) -> ("array out"=w1846:dbl[], "no input?"=w1835:bool)
              n1477 = Or(x="Let 2", y="Let 5") -> (x .or. y?=w1791:bool)
              n1478 = Build Array("Expected Winner1 2", "Expected Winner2 2", "Unexpected Winner1 2", "Unexpected Winner2 2", "Stroke1 2", "Stroke2 2", "Forced Error1 2", "Forced Error2 2", "Unforced Error1 2", "Unforced Error2 2", "Nolet1 2", "Nolet2 2", w1791) -> (w1827:bool[])
              n1479 = call "or multiple inputs.vi"("zero array in"=w1851, "input array in"=w1827, "file data in"=w1862) -> ("array out"=w1847:dbl[], "no input?"=w1834:bool)
              n1480 = Build Array("FH", "BH") -> (w1830:bool[])
              n1481 = Build Array("ST", "CR") -> (w1829:bool[])
              n1482 = Build Array("Bounce", "Half Volley", "Volley") -> (w1828:bool[])
              n1483 = Build Array("Player1 2", "Player2 2") -> (w1825:bool[])
              n1484 = Build Array("Button 6", "Button 7", "Button 8", "Button 9", "Button 10") -> (w1824:bool[])
              n1485 = Build Array("Service1 2", "Service2 2", "S1 2", "S2 2", "S3 2", "S4 2", "S5 2", "S6 2") -> (w1826:bool[])
              n1486 = call "or multiple inputs.vi"("zero array in"=w1851, "input array in"=w1830, "file data in"=w1873) -> ("array out"=w1850:dbl[], "no input?"=w1841:bool)
              n1487 = call "or multiple inputs.vi"("zero array in"=w1851, "input array in"=w1829, "file data in"=w1872) -> ("array out"=w1849:dbl[], "no input?"=w1840:bool)
              n1488 = call "or multiple inputs.vi"("zero array in"=w1851, "input array in"=w1828, "file data in"=w1871) -> ("array out"=w1842:dbl[], "no input?"=w1839:bool)
              n1489 = call "or multiple inputs.vi"("zero array in"=w1851, "input array in"=w1825, "file data in"=w1853) -> ("array out"=w1843:dbl[], "no input?"=w1838:bool)
              n1490 = call "or multiple inputs.vi"("zero array in"=w1851, "input array in"=w1824, "file data in"=w1852) -> ("array out"=w1844:dbl[], "no input?"=w1837:bool)
              n1491 = call "or multiple inputs.vi"("zero array in"=w1851, "input array in"=w1826, "file data in"=w1861) -> ("array out"=w1845:dbl[], "no input?"=w1836:bool)
              n1492 = Compound Arithmetic op=AND(w1850, w1849, w1842, w1843, w1844, w1845, w1846, w1847, w1848) -> (w1923:i32[])
              "result" <- w1923
              n1493 = Compound Arithmetic op=AND(w1841, w1840, w1839, w1838, w1837, w1836, w1835, w1834, w1833) -> (w1921:bool)
              n1494 = Select(t=i32[] [] ("result"), s=w1921, f=w1923) -> (s? t:f=w1936:i32[])
              "EVENTS\nTO PLAY" <- w1936
              n1495 = local read "Combined data"() -> (w1815:i64[][])
              n1496 = Insert Into Array(array=w1832, new element #1=w1831, new element #2=w1830, new element #3=w1829, new element #4=w1828, new element #5=w1827, new element #6=w1826, new element #7=w1825, new element #8=w1824) -> (w1823:bool[])  [unwired: 1 in]
              "Last Edit" <- w1823
              n1497 = for {
                tunnel: w1815 -> [w1965]
                tunnel: w1936 -> [w1974] mode=indexing
                shift-right: [w1975] -> w1933
                shift-left: w1934 -> [w1976]
                shift-right: [w1969] -> w1932
                shift-left: w1934 -> [w1970]
                shift-right: [w1962] -> w1931
                shift-left: w1934 -> [w1963]
                i -> [w1967]
                n1498 = Increment(x=w1967) -> (x+1=w1966:i32)
                n1499 = Decrement(x=w1967) -> (x-1=w1973:i32)
                n1500 = Index Array(array=w1965, index (row)=w1967) -> (element=w1978:i64[])  [unwired: 1 in]
                n1501 = Index Array(array=w1965, index (row)=w1966) -> (element=w1968:i64[])  [unwired: 1 in]
                n1502 = Not Equal To 0?(x=w1974) -> (x != 0?=w1961:bool)
                n1503 = Index Array(array=w1965, index (row)=w1973) -> (element=w1972:i64[])  [unwired: 1 in]
                n1504 = Insert Into Array(array=w1963, new element=w1968) -> (w1964:i64[][])  [unwired: 2 in]
                n1505 = Insert Into Array(array=w1976, new element=w1978) -> (w1977:i64[][])  [unwired: 2 in]
                n1506 = Insert Into Array(array=w1970, new element=w1972) -> (w1971:i64[][])  [unwired: 2 in]
                n1507 = Select(t=w1971, s=w1961, f=w1970) -> (s? t:f=w1969:i64[][])
                n1508 = Select(t=w1964, s=w1961, f=w1963) -> (s? t:f=w1962:i64[][])
                n1509 = Select(t=w1977, s=w1961, f=w1976) -> (s? t:f=w1975:i64[][])
              }
              "Edited data" <- w1933
              "Event After" <- w1931
              "Event before" <- w1932
              n1510 = Or Array Elements(Boolean array=w1823) -> (logical OR=w1814:bool)
              n1511 = Index Array(array=w1933, index (col) #1=0 ("disabled index (col)"), index (col) #2=1 ("disabled index (row)"), index (col) #3=2 ("disabled index (col)")) -> (element #1=w1942:i64[], element #2=w1799:i64[], element #3=w1798:i64[])  [unwired: 3 in]
              n1512 = Build Array(w1942) -> (w1930:i64[][])
              n1513 = Empty Array?(array=w1942) -> (empty?=w1821:bool)
              n1514 = Array Size(array=w1942) -> (size(s)=w1943:i32)
              n1515 = local read "framesPerSecond"() -> (w1797:u32)
              n1516 = Transpose 2D Array(2D array=w1930) -> (transposed array=→"edited\nevents":i64[][])
              n1517 = property on="Code number display" class="DigNum (strict)"("Maximum"=w1943, "Minimum"=1.0 ("Data Entry Limits:Minimum")) -> ()  [unwired: 2 in, 2 out]
              n1518 = And(x=w1821, y=w1814) -> (x .and. y?=w1822:bool)
              n1519 = case shown="True" w1822 {
                frame False {
                  n1520 = for {
                    N: 300 -> [_]
                    i -> [w2010]
                    n1521 = Increment(x=w2010) -> (x+1=w2009:i32)
                    n1522 = local write "task"(w2009) -> ()
                    n1523 = Wait (ms)(milliseconds to wait=u32 1) -> ()  [unwired: 1 out]
                  }
                }
                frame True {
                  n1524 = One Button Dialog(message="INVALID EVENTS\n\nSelected event(s) or combination of events does not exist") -> ()  [unwired: 1 in, 1 out]
                }
              }
              n1525 = for {
                tunnel: "after" -> [w1981]
                tunnel: w1942 -> [w2000] mode=indexing
                shift-right: [w1994] -> w1813
                shift-left: u32[] [] -> [w1996]
                tunnel: w1799 -> [w1984] mode=indexing
                tunnel: [w1980] -> _ mode=indexing
                tunnel: w1798 -> [w1980] mode=indexing
                tunnel: w1797 -> [w1986]
                tunnel: "before" -> [w1985]
                tunnel: "playback interval on" -> [w1979]
                n1526 = Select(t=w1985, s=w1979, f=w1984) -> (s? t:f=w1983:i64)
                n1527 = Select(t=w1981, s=w1979, f=w1980) -> (s? t:f=w1982:i64)
                n1528 = Multiply(x=w1986, y=w1983) -> (x*y=w1988:i64)
                n1529 = Multiply(x=w1986, y=w1982) -> (x*y=w1987:i64)
                n1530 = Array Max & Min(array=w1996) -> (max value=w1999:u32, max index (indices)=w1995:i32)  [unwired: 2 out]
                n1531 = Subtract(x=w2000, y=w1988) -> (x-y=w1998:i64)
                n1532 = Add(x=w1987, y=w2000) -> (x+y=w1997:i64)
                n1533 = Greater Or Equal?(x=w1999, y=w1998) -> (x >= y?=w1991:bool)
                n1534 = Build Array(w1998, w1997) -> (w1989:i64[])
                n1535 = Build Array(w1997) -> (w1993:i64[])
                n1536 = And(x="Combine", y=w1991) -> (x .and. y?=w1992:bool)
                n1537 = case shown="True" w1992 {
                  tunnel: w1996 -> [w2003 w2007]
                  tunnel: w1995 -> [_ w2006]
                  tunnel: w1993 -> [_ w2005]
                  tunnel: [w2002 w2004] -> w1994
                  tunnel: w1989 -> [w2001 _]
                  frame False {
                    n1538 = Insert Into Array(array=w2003, new element=w2001) -> (w2002:u32[])  [unwired: 1 in]
                  }
                  frame True {
                    n1539 = Replace Array Subset(array=w2007, new element=w2005, index=w2006) -> (w2004:u32[])
                  }
                }
              }
              n1540 = Delete From Array(array=w1815, length=1, index (col)=0 ("disabled index (col)")) -> (deleted portion=w1820:i64[][])  [unwired: 1 in, 1 out]
              n1541 = Array Max & Min(array=w1820) -> (max value=w1819:i64, min value=w1818:i64)  [unwired: 2 out]
              n1542 = Build Array(w1818, w1819) -> (w1811:i64[])
              n1543 = Select(t=w1813, s=w1814, f=w1811) -> (s? t:f=w1812:i64[])
              "edited to play" <- w1812
              n1544 = Array Size(array=w1812) -> (size(s)=w1925:i32)
              n1545 = Divide(x=w1925, y=2) -> (x/y=w1926:dbl)
              n1546 = for {
                N: w1926 -> [_]
                shift-right: [w1951] -> _
                shift-left: w1812 -> [w1953]
                shift-right: [w1946] -> w1924
                shift-left: i64[] [] ("edited\nto play 3") -> [w1947]
                n1547 = Split 1D Array(array=w1953, index=2) -> (first subarray=w1952:i64[], second subarray=w1951:i64[])
                n1548 = Index Array(array=w1952, index #1=1 ("index"), index #2=0 ("index")) -> (element #1=w1957:i64, element #2=w1950:i64)
                n1549 = Subtract(x=w1957, y=w1950) -> (x-y=w1949:i64)
                n1550 = Increment(x=w1949) -> (x+1=w1948:i64)
                n1551 = for {
                  N: w1948 -> [_]
                  tunnel: w1950 -> [w1960]
                  tunnel: [w1958] -> w1945 mode=indexing
                  tunnel: [w1958] -> _
                  i -> [w1959]
                  n1552 = Add(x=w1960, y=w1959) -> (x+y=w1958:i64)
                }
                n1553 = Insert Into Array(array=w1947, new element=w1945) -> (w1946:i64[])  [unwired: 1 in]
              }
              n1554 = local read "Number of Frames"() -> (w1939:u32)
              n1555 = Subtract(x=w1939, y=u32 2) -> (x-y=w1941:u32)
              n1556 = In Range and Coerce(upper limit=0, x=w1924, lower limit=w1941) -> (coerced(x)=w1810:i64[])  [unwired: 1 out]
              "frames edited" <- w1810
              "frames 2 play" <- w1810
              n1557 = for {
                tunnel: w1810 -> [_] mode=indexing
                shift-right: [w2017] -> _
                shift-left: w1810 -> [w2016]
                i -> [w2013]
                n1558 = Index Array(array=w2016, index=w2013) -> (element=w2015:i64)
                n1559 = Increment(x=w2013) -> (x+1=w2014:i32)
                n1560 = while {
                  shift-right: [w2022] -> w2017
                  shift-left: w2016 -> [w2023]
                  tunnel: w2015 -> [w2024]
                  tunnel: w2014 -> [w2018]
                  stop <- w2019 stop-if-true
                  n1561 = Search 1D Array(1D array=w2023, element=w2024, start index (0)=w2018) -> (index of element=w2021:i32)
                  n1562 = Equal?(x=w2021, y=-1) -> (x = y?=w2019:bool)
                  n1563 = Delete From Array(array=w2023, index=w2021) -> (array with subset deleted=w2022:i64[])  [unwired: 1 in, 1 out]
                }
              }
            }
          }
          n1564 = local read "refnum of data save file"() -> (w1754:refnum<file>)
        }
        frame "Examine coding" {
          w2102 = T4."Enabled" ("Disabled")
          n1565 = property on="Code number display" class="DigNum (strict)"("DisabledEnum"=w2102) -> ()  [unwired: 2 in, 2 out]
          n1566 = property on="Next" class="Bool (strict)"("DisabledEnum"=w2102) -> ()  [unwired: 2 in, 2 out]
          n1567 = property on="Reset" class="Bool (strict)"("DisabledEnum"=w2102) -> ()  [unwired: 2 in, 2 out]
          n1568 = property on="Update" class="Bool (strict)"("DisabledEnum"=w2102) -> ()  [unwired: 2 in, 2 out]
          n1569 = property on="Previous" class="Bool (strict)"("DisabledEnum"=w2102) -> ()  [unwired: 2 in, 2 out]
          n1570 = local read "edited\nevents"() -> (w2110:i64[][])
          n1571 = Decrement(x="Code number display") -> (x-1=w2103:i32)
          n1572 = flat-sequence {
            tunnel: "Code number display" -> [w2127]
            frame #0 {
              n1573 = local read "edited to play"() -> (w2126:i64[])
              n1574 = for {
                N: w2127 -> [_]
                shift-right: [w2132] -> _
                shift-left: w2126 -> [w2133]
                tunnel: [w2131] -> w2119
                n1575 = Split 1D Array(array=w2133, index=2) -> (first subarray=w2131:i64[], second subarray=w2132:i64[])
              }
              n1576 = Index Array(array=w2119, index #1=1 ("index"), index #2=0 ("index")) -> (element #1=w2125:i64, element #2=w2122:i64)
              n1577 = Subtract(x=w2125, y=w2122) -> (x-y=w2121:i64)
              n1578 = Increment(x=w2121) -> (x+1=w2120:i64)
              n1579 = for {
                N: w2120 -> [_]
                tunnel: w2122 -> [w2130]
                tunnel: [w2128] -> w2118 mode=indexing
                i -> [w2129]
                n1580 = Add(x=w2130, y=w2129) -> (x+y=w2128:i64)
              }
              n1581 = local write "Progress..."(u32 0 ("Progress...")) -> ()
              n1582 = local write "frames 2 play"(w2118) -> ()
            }
            frame #1 {
              w2135 = TRUE ("Play")
              w2136 = FALSE ("Next")
              n1583 = local write "Next"(w2136) -> ()
              n1584 = local write "Previous"(w2136) -> ()
              n1585 = local write "Reset"(w2136) -> ()
              n1586 = local write "stop"(w2136) -> ()
              n1587 = local write "Pause"(w2136) -> ()
              n1588 = local write "Load video"(w2135) -> ()
              n1589 = local write "Play"(w2135) -> ()
            }
          }
          n1590 = Index Array(array=w2110, index (row)=w2103, index (col)=0) -> (element=w2109:i64)
          n1591 = Index Array(array=w2107, index (col)=0 ("disabled index (col)")) -> (element=w2114:i64[])  [unwired: 1 in]
          n1592 = Search 1D Array(1D array=w2114, element=w2109) -> (index of element=w2113:i32)  [unwired: 1 in]
          n1593 = Index Array(array=w2107, index (row)=w2113) -> (element=w2112:i64[])  [unwired: 1 in]
          n1594 = Delete From Array(array=w2112, length=3, index=0) -> (array with subset deleted=w2111:i64[])  [unwired: 1 out]
          n1595 = for {
            tunnel: w2111 -> [w2141] mode=indexing
            tunnel: [w2137] -> w2026 mode=indexing
            n1596 = Equal To 0?(x=w2141) -> (x = 0?=w2140:bool)
            n1597 = Select(t=FALSE ("x = 0?"), s=w2140, f=TRUE) -> (s? t:f=w2137:bool)
          }
          n1598 = Split 1D Array(array=w2026, index=24) -> (first subarray=w2051:bool[], second subarray=w2052:bool[])
          n1599 = Index Array(array=w2051) -> (element #1=w2050:bool, element #2=w2049:bool, element #3=w2048:bool, element #4=w2047:bool, element #5=w2046:bool, element #6=w2045:bool, element #7=w2044:bool, element #8=w2043:bool, element #9=w2042:bool, element #10=w2041:bool, element #11=w2040:bool, element #12=w2039:bool, element #13=w2038:bool, element #14=w2037:bool, element #15=w2036:bool, element #16=w2035:bool, element #17=w2034:bool, element #18=w2033:bool, element #19=w2032:bool, element #20=w2031:bool, element #21=w2030:bool, element #22=w2029:bool, element #23=w2028:bool, element #24=w2027:bool)  [unwired: 30 in, 6 out]
          n1600 = Split 1D Array(array=w2052, index=34) -> (first subarray=w2053:bool[], second subarray=w2054:bool[])
          n1601 = local write "1 10"(w2050) -> ()
          n1602 = local write "1 7"(w2049) -> ()
          n1603 = local write "1 6"(w2048) -> ()
          n1604 = local write "1 5"(w2047) -> ()
          n1605 = local write "2 10"(w2046) -> ()
          n1606 = local write "2 7"(w2045) -> ()
          n1607 = local write "2 6"(w2044) -> ()
          n1608 = local write "2 5"(w2043) -> ()
          n1609 = local write "3 9"(w2042) -> ()
          n1610 = local write "3 7"(w2041) -> ()
          n1611 = local write "3 6"(w2040) -> ()
          n1612 = local write "3 5"(w2039) -> ()
          n1613 = local write "4 9"(w2038) -> ()
          n1614 = local write "4 7"(w2037) -> ()
          n1615 = local write "4 6"(w2036) -> ()
          n1616 = local write "4 5"(w2035) -> ()
          n1617 = local write "5 8"(w2034) -> ()
          n1618 = local write "5 7"(w2033) -> ()
          n1619 = local write "5 6"(w2032) -> ()
          n1620 = local write "5 5"(w2031) -> ()
          n1621 = local write "6 8"(w2030) -> ()
          n1622 = local write "6 7"(w2029) -> ()
          n1623 = local write "6 6"(w2028) -> ()
          n1624 = local write "6 5"(w2027) -> ()
          n1625 = Index Array(array=w2053) -> (element #1=w2099:bool, element #2=w2098:bool, element #3=w2097:bool, element #4=w2096:bool, element #5=w2095:bool, element #6=w2094:bool, element #7=w2093:bool, element #8=w2092:bool, element #9=w2091:bool, element #10=w2090:bool, element #11=w2089:bool, element #12=w2088:bool, element #13=w2087:bool, element #14=w2086:bool, element #15=w2085:bool, element #16=w2084:bool, element #17=w2083:bool, element #18=w2082:bool, element #19=w2081:bool, element #20=w2080:bool, element #21=w2079:bool, element #22=w2078:bool, element #23=w2077:bool, element #24=w2076:bool, element #25=w2075:bool, element #26=w2074:bool, element #27=w2073:bool, element #28=w2072:bool, element #29=w2071:bool, element #30=w2025:bool)  [unwired: 30 in]
          n1626 = local write "Adrive"(w2099) -> ()
          n1627 = local write "Ddrive"(w2098) -> ()
          n1628 = local write "ASWdrive"(w2097) -> ()
          n1629 = local write "DSWdrive"(w2096) -> ()
          n1630 = local write "Drop 14"(w2095) -> ()
          n1631 = local write "Chop 13"(w2094) -> ()
          n1632 = local write "Lob"(w2093) -> ()
          n1633 = local write "Boast2"(w2092) -> ()
          n1634 = local write "Boast3"(w2091) -> ()
          n1635 = local write "Smash 13"(w2090) -> ()
          n1636 = local write "FH"(w2089) -> ()
          n1637 = local write "BH"(w2088) -> ()
          n1638 = local write "ST"(w2087) -> ()
          n1639 = local write "CR"(w2086) -> ()
          n1640 = local write "Bounce"(w2085) -> ()
          n1641 = local write "Half Volley"(w2084) -> ()
          n1642 = local write "Volley"(w2083) -> ()
          n1643 = local write "Expected Winner1 2"(w2082) -> ()
          n1644 = local write "Expected Winner2 2"(w2081) -> ()
          n1645 = local write "Unexpected Winner1 2"(w2080) -> ()
          n1646 = local write "Unexpected Winner2 2"(w2079) -> ()
          n1647 = local write "Stroke1 2"(w2078) -> ()
          n1648 = local write "Stroke2 2"(w2077) -> ()
          n1649 = local write "Forced Error1 2"(w2076) -> ()
          n1650 = local write "Forced Error2 2"(w2075) -> ()
          n1651 = local write "Unforced Error1 2"(w2074) -> ()
          n1652 = local write "Unforced Error2 2"(w2073) -> ()
          n1653 = local write "Nolet1 2"(w2072) -> ()
          n1654 = local write "Nolet2 2"(w2071) -> ()
          n1655 = local write "Let 2"(w2025) -> ()
          n1656 = local write "Let 5"(w2025) -> ()
          n1657 = Index Array(array=w2054) -> (element #1=w2070:bool, element #2=w2069:bool, element #3=w2068:bool, element #4=w2067:bool, element #5=w2066:bool, element #6=w2065:bool, element #7=w2064:bool, element #8=w2063:bool, element #9=w2062:bool, element #10=w2061:bool, element #11=w2060:bool, element #12=w2059:bool, element #13=w2058:bool, element #14=w2057:bool, element #15=w2056:bool)  [unwired: 15 in]
          n1658 = local write "Service1 2"(w2070) -> ()
          n1659 = local write "Service2 2"(w2069) -> ()
          n1660 = local write "S1 2"(w2068) -> ()
          n1661 = local write "S2 2"(w2067) -> ()
          n1662 = local write "S3 2"(w2066) -> ()
          n1663 = local write "S4 2"(w2065) -> ()
          n1664 = local write "S5 2"(w2064) -> ()
          n1665 = local write "S6 2"(w2063) -> ()
          n1666 = local write "Player1 2"(w2062) -> ()
          n1667 = local write "Player2 2"(w2061) -> ()
          n1668 = local write "Button 6"(w2060) -> ()
          n1669 = local write "Button 7"(w2059) -> ()
          n1670 = local write "Button 8"(w2058) -> ()
          n1671 = local write "Button 9"(w2057) -> ()
          n1672 = local write "Button 10"(w2056) -> ()
          n1673 = local read "refnum of data save file"() -> (w2105:refnum<file>)
        }
        frame "Edit coding" {
          n1674 = local read "Examine code"() -> (w2143:bool)
          n1675 = case shown="False" w2143 {
            tunnel: [T1."Edit video" ("Main tab") w2226] -> w2145
            frame False {
              n1676 = local read "Last Edit"() -> (w2220:bool[])
              n1677 = Split 1D Array(array=w2220, index=24) -> (first subarray=w2171:bool[], second subarray=w2172:bool[])
              n1678 = Index Array(array=w2171) -> (element #1=w2170:bool, element #2=w2169:bool, element #3=w2168:bool, element #4=w2167:bool, element #5=w2166:bool, element #6=w2165:bool, element #7=w2164:bool, element #8=w2163:bool, element #9=w2162:bool, element #10=w2161:bool, element #11=w2160:bool, element #12=w2159:bool, element #13=w2158:bool, element #14=w2157:bool, element #15=w2156:bool, element #16=w2155:bool, element #17=w2154:bool, element #18=w2153:bool, element #19=w2152:bool, element #20=w2151:bool, element #21=w2150:bool, element #22=w2149:bool, element #23=w2148:bool, element #24=w2147:bool)  [unwired: 30 in, 6 out]
              n1679 = Split 1D Array(array=w2172, index=30) -> (first subarray=w2173:bool[], second subarray=w2174:bool[])
              n1680 = local write "1 10"(w2170) -> ()
              n1681 = local write "1 7"(w2169) -> ()
              n1682 = local write "1 6"(w2168) -> ()
              n1683 = local write "1 5"(w2167) -> ()
              n1684 = local write "2 10"(w2166) -> ()
              n1685 = local write "2 7"(w2165) -> ()
              n1686 = local write "2 6"(w2164) -> ()
              n1687 = local write "2 5"(w2163) -> ()
              n1688 = local write "3 9"(w2162) -> ()
              n1689 = local write "3 7"(w2161) -> ()
              n1690 = local write "3 6"(w2160) -> ()
              n1691 = local write "3 5"(w2159) -> ()
              n1692 = local write "4 9"(w2158) -> ()
              n1693 = local write "4 7"(w2157) -> ()
              n1694 = local write "4 6"(w2156) -> ()
              n1695 = local write "4 5"(w2155) -> ()
              n1696 = local write "5 8"(w2154) -> ()
              n1697 = local write "5 7"(w2153) -> ()
              n1698 = local write "5 6"(w2152) -> ()
              n1699 = local write "5 5"(w2151) -> ()
              n1700 = local write "6 8"(w2150) -> ()
              n1701 = local write "6 7"(w2149) -> ()
              n1702 = local write "6 6"(w2148) -> ()
              n1703 = local write "6 5"(w2147) -> ()
              n1704 = Index Array(array=w2173) -> (element #1=w2219:bool, element #2=w2218:bool, element #3=w2217:bool, element #4=w2216:bool, element #5=w2215:bool, element #6=w2214:bool, element #7=w2213:bool, element #8=w2212:bool, element #9=w2211:bool, element #10=w2210:bool, element #11=w2209:bool, element #12=w2208:bool, element #13=w2207:bool, element #14=w2206:bool, element #15=w2205:bool, element #16=w2204:bool, element #17=w2203:bool, element #18=w2202:bool, element #19=w2201:bool, element #20=w2200:bool, element #21=w2199:bool, element #22=w2198:bool, element #23=w2197:bool, element #24=w2196:bool, element #25=w2195:bool, element #26=w2194:bool, element #27=w2193:bool, element #28=w2192:bool, element #29=w2191:bool, element #30=w2146:bool)  [unwired: 30 in]
              n1705 = local write "Adrive"(w2219) -> ()
              n1706 = local write "Ddrive"(w2218) -> ()
              n1707 = local write "ASWdrive"(w2217) -> ()
              n1708 = local write "DSWdrive"(w2216) -> ()
              n1709 = local write "Drop 14"(w2215) -> ()
              n1710 = local write "Chop 13"(w2214) -> ()
              n1711 = local write "Lob"(w2213) -> ()
              n1712 = local write "Boast2"(w2212) -> ()
              n1713 = local write "Boast3"(w2211) -> ()
              n1714 = local write "Smash 13"(w2210) -> ()
              n1715 = local write "FH"(w2209) -> ()
              n1716 = local write "BH"(w2208) -> ()
              n1717 = local write "ST"(w2207) -> ()
              n1718 = local write "CR"(w2206) -> ()
              n1719 = local write "Bounce"(w2205) -> ()
              n1720 = local write "Half Volley"(w2204) -> ()
              n1721 = local write "Volley"(w2203) -> ()
              n1722 = local write "Expected Winner1 2"(w2202) -> ()
              n1723 = local write "Expected Winner2 2"(w2201) -> ()
              n1724 = local write "Unexpected Winner1 2"(w2200) -> ()
              n1725 = local write "Unexpected Winner2 2"(w2199) -> ()
              n1726 = local write "Stroke1 2"(w2198) -> ()
              n1727 = local write "Stroke2 2"(w2197) -> ()
              n1728 = local write "Forced Error1 2"(w2196) -> ()
              n1729 = local write "Forced Error2 2"(w2195) -> ()
              n1730 = local write "Unforced Error1 2"(w2194) -> ()
              n1731 = local write "Unforced Error2 2"(w2193) -> ()
              n1732 = local write "Nolet1 2"(w2192) -> ()
              n1733 = local write "Nolet2 2"(w2191) -> ()
              n1734 = local write "Let 2"(w2146) -> ()
              n1735 = local write "Let 5"(w2146) -> ()
              n1736 = Index Array(array=w2174) -> (element #1=w2190:bool, element #2=w2189:bool, element #3=w2188:bool, element #4=w2187:bool, element #5=w2186:bool, element #6=w2185:bool, element #7=w2184:bool, element #8=w2183:bool, element #9=w2182:bool, element #10=w2181:bool, element #11=w2180:bool, element #12=w2179:bool, element #13=w2178:bool, element #14=w2177:bool, element #15=w2176:bool)  [unwired: 15 in]
              n1737 = local write "Service1 2"(w2190) -> ()
              n1738 = local write "Service2 2"(w2189) -> ()
              n1739 = local write "S1 2"(w2188) -> ()
              n1740 = local write "S2 2"(w2187) -> ()
              n1741 = local write "S3 2"(w2186) -> ()
              n1742 = local write "S4 2"(w2185) -> ()
              n1743 = local write "S5 2"(w2184) -> ()
              n1744 = local write "S6 2"(w2183) -> ()
              n1745 = local write "Player1 2"(w2182) -> ()
              n1746 = local write "Player2 2"(w2181) -> ()
              n1747 = local write "Button 6"(w2180) -> ()
              n1748 = local write "Button 7"(w2179) -> ()
              n1749 = local write "Button 8"(w2178) -> ()
              n1750 = local write "Button 9"(w2177) -> ()
              n1751 = local write "Button 10"(w2176) -> ()
              n1752 = local write "Upload edited video"(TRUE ("Upload edited video")) -> ()
            }
            frame True {
              n1753 = event shown="[0] Timeout" {
                selector: _ -> [_ _]
                dyn-events: _ -> [_ _]
                timeout: 25 -> [_ _]
                tunnel: [FALSE TRUE] -> w2224
                event Timeout {
                  n1754 = event-data() -> ()  [unwired: 1 in, 3 out]
                }
                event "Code number display": Value Change {
                  n1755 = event-data() -> ()  [unwired: 1 in, 3 out]
                }
              }
              n1756 = case shown="True" "Next" {
                frame False {
                }
                frame True {
                  n1757 = local read "edited\nevents"() -> (w2243:i64[][])
                  n1758 = local read "Code number display"() -> (w2239:i32)
                  n1759 = Index Array(array=w2243, index (col)=0 ("disabled index (col)")) -> (element=w2245:i64[])  [unwired: 1 in]
                  n1760 = Array Size(array=w2245) -> (size(s)=w2238:i32)
                  n1761 = Increment(x=w2239) -> (x+1=w2241:i32)
                  n1762 = Less Or Equal?(x=w2241, y=w2238) -> (x <= y?=w2242:bool)
                  n1763 = Select(t=w2241, s=w2242, f=w2238) -> (s? t:f=w2240:i32)
                  n1764 = local write "Code number display"(w2240) -> ()
                }
              }
              n1765 = case shown="True" "Previous" {
                frame False {
                }
                frame True {
                  n1766 = local read "Code number display"() -> (w2246:i32)
                  n1767 = Decrement(x=w2246) -> (x-1=w2249:i32)
                  n1768 = Greater Than 0?(x=w2249) -> (x > 0?=w2250:bool)
                  n1769 = Select(t=w2249, s=w2250, f=1) -> (s? t:f=w2247:i32)
                  n1770 = local write "Code number display"(w2247) -> ()
                }
              }
              n1771 = Compound Arithmetic op=OR(w2224, "Reset", "Previous", "Next") -> (w2232:bool)
              n1772 = Select(t=T1."Examine coding" ("Main tab"), s=w2232, f=T1."Edit coding" ("Main tab")) -> (s? t:f=w2227:T1)
              n1773 = Select(t=T1."Update coding" ("Main tab"), s="Update", f=w2227) -> (s? t:f=w2226:T1)
            }
          }
          n1774 = local read "refnum of data save file"() -> (w2142:refnum<file>)
        }
        frame "Update coding" {
          w2251 = "\t"
          w2275 = "\r"
          n1775 = flat-sequence {
            tunnel: w2279 -> [w2374]
            tunnel: [w2371] -> w2278
            tunnel: w2278 -> [w2458]
            tunnel: [w2458] -> w2261
            frame #0 {
              w2321 = FALSE
              n1776 = local read "Service1 2"() -> (w2320:bool)
              n1777 = local read "Service2 2"() -> (w2319:bool)
              n1778 = local read "Button 10"() -> (w2306:bool)
              n1779 = local read "Player1 2"() -> (w2312:bool)
              n1780 = local read "Player2 2"() -> (w2311:bool)
              n1781 = local read "Button 6"() -> (w2310:bool)
              n1782 = local read "Button 7"() -> (w2309:bool)
              n1783 = local read "Button 8"() -> (w2308:bool)
              n1784 = local read "Button 9"() -> (w2307:bool)
              n1785 = local read "S1 2"() -> (w2318:bool)
              n1786 = local read "S2 2"() -> (w2317:bool)
              n1787 = local read "S3 2"() -> (w2316:bool)
              n1788 = local read "S4 2"() -> (w2315:bool)
              n1789 = local read "S5 2"() -> (w2314:bool)
              n1790 = local read "S6 2"() -> (w2313:bool)
              n1791 = local read "1 10"() -> (w2368:bool)
              n1792 = local read "2 10"() -> (w2364:bool)
              n1793 = local read "5 8"() -> (w2301:bool)
              n1794 = local read "5 7"() -> (w2300:bool)
              n1795 = local read "5 6"() -> (w2299:bool)
              n1796 = local read "5 5"() -> (w2298:bool)
              n1797 = local read "6 8"() -> (w2297:bool)
              n1798 = local read "6 7"() -> (w2296:bool)
              n1799 = local read "6 6"() -> (w2295:bool)
              n1800 = local read "6 5"() -> (w2294:bool)
              n1801 = local read "1 7"() -> (w2367:bool)
              n1802 = local read "1 6"() -> (w2366:bool)
              n1803 = local read "1 5"() -> (w2365:bool)
              n1804 = local read "2 7"() -> (w2363:bool)
              n1805 = local read "2 6"() -> (w2362:bool)
              n1806 = local read "2 5"() -> (w2361:bool)
              n1807 = local read "3 9"() -> (w2360:bool)
              n1808 = local read "3 7"() -> (w2359:bool)
              n1809 = local read "3 6"() -> (w2358:bool)
              n1810 = local read "3 5"() -> (w2357:bool)
              n1811 = local read "4 9"() -> (w2356:bool)
              n1812 = local read "4 7"() -> (w2355:bool)
              n1813 = local read "4 6"() -> (w2354:bool)
              n1814 = local read "4 5"() -> (w2353:bool)
              n1815 = Build Array(w2320, w2319, w2318, w2317, w2316, w2315, w2314, w2313, w2312, w2311, w2310, w2309, w2308, w2307, w2306) -> (w2303:bool[])
              n1816 = Build Array(w2368, w2367, w2366, w2365, w2364, w2363, w2362, w2361, w2360, w2359, w2358, w2357, w2356, w2355, w2354, w2353, w2301, w2300, w2299, w2298, w2297, w2296, w2295, w2294) -> (w2305:bool[])
              n1817 = local read "Unexpected Winner1 2"() -> (w2334:bool)
              n1818 = local read "Unexpected Winner2 2"() -> (w2327:bool)
              n1819 = local read "Expected Winner1 2"() -> (w2335:bool)
              n1820 = local read "Expected Winner2 2"() -> (w2328:bool)
              n1821 = local read "Unforced Error1 2"() -> (w2324:bool)
              n1822 = local read "Unforced Error2 2"() -> (w2331:bool)
              n1823 = local read "Forced Error1 2"() -> (w2325:bool)
              n1824 = local read "Forced Error2 2"() -> (w2332:bool)
              n1825 = local read "ASWdrive"() -> (w2350:bool)
              n1826 = local read "DSWdrive"() -> (w2349:bool)
              n1827 = local read "Smash 13"() -> (w2343:bool)
              n1828 = local read "Stroke1 2"() -> (w2333:bool)
              n1829 = local read "Stroke2 2"() -> (w2326:bool)
              n1830 = local read "Volley"() -> (w2336:bool)
              n1831 = local read "Chop 13"() -> (w2347:bool)
              n1832 = local read "Half Volley"() -> (w2337:bool)
              n1833 = local read "Nolet1 2"() -> (w2323:bool)
              n1834 = local read "Nolet2 2"() -> (w2330:bool)
              n1835 = local read "Drop 14"() -> (w2348:bool)
              n1836 = local read "Bounce"() -> (w2338:bool)
              n1837 = local read "Boast2"() -> (w2345:bool)
              n1838 = local read "Boast3"() -> (w2344:bool)
              n1839 = local read "Adrive"() -> (w2352:bool)
              n1840 = local read "Ddrive"() -> (w2351:bool)
              n1841 = local read "Let 2"() -> (w2285:bool)
              n1842 = local read "Let 5"() -> (w2286:bool)
              n1843 = local read "Lob"() -> (w2346:bool)
              n1844 = local read "BH"() -> (w2341:bool)
              n1845 = local read "FH"() -> (w2342:bool)
              n1846 = local read "CR"() -> (w2339:bool)
              n1847 = local read "ST"() -> (w2340:bool)
              n1848 = Or(x=w2285, y=w2286) -> (x .or. y?=w2284:bool)
              n1849 = Compound Arithmetic op=OR(w2328, w2327, w2326, w2325, w2324, w2323) -> (w2322:bool)
              n1850 = Compound Arithmetic op=OR(w2335, w2334, w2333, w2332, w2331, w2330) -> (w2329:bool)
              n1851 = Build Array(w2352, w2351, w2350, w2349, w2348, w2347, w2346, w2345, w2344, w2343, w2342, w2341, w2340, w2339, w2338, w2337, w2336, w2335, w2328, w2334, w2327, w2333, w2326, w2325, w2332, w2324, w2331, w2323, w2330, w2284, w2329, w2322, w2321, w2321) -> (w2304:bool[])
              n1852 = Insert Into Array(array=w2305, new element #1=w2304, new element #2=w2303) -> (w2302:bool[])  [unwired: 1 in]
              n1853 = Boolean To (0,1)(Boolean=w2302) -> (0, 1=w2375:i16[])
              "0, 1" <- w2375
              n1854 = local read "Code number display"() -> (w2370:i32)
              n1855 = local read "edited\nevents"() -> (w2376:i64[][])
              n1856 = Decrement(x=w2370) -> (x-1=w2369:i32)
              n1857 = Index Array(array=w2374, index (col)=0 ("disabled index (col)")) -> (element=w2379:i64[])  [unwired: 1 in]
              n1858 = Index Array(array=w2376, index (row)=w2369, index (col)=0) -> (element=w2378:i64)
              n1859 = Search 1D Array(1D array=w2379, element=w2378) -> (index of element=w2372:i32)  [unwired: 1 in]
              n1860 = Index Array(array=w2374, index (row)=w2372) -> (element=w2293:i64[])  [unwired: 1 in]
              n1861 = Delete From Array(array=w2293, index=0) -> ()  [unwired: 1 in, 2 out]
              n1862 = Index Array(array=w2293, index #1=0 ("index"), index #2=1 ("index"), index #3=2 ("index")) -> (element #1=w2292:i64, element #2=w2291:i64, element #3=w2290:i64)
              n1863 = Build Array (concatenate)(w2292, w2291, w2290, w2375) -> (w2373:i64[])
              "appended array" <- w2373
              n1864 = Replace Array Subset(array=w2374, new element=w2373, index (row)=w2372) -> (w2371:i64[][])  [unwired: 1 in]
              "output array" <- w2371
            }
            frame #1 {
              n1865 = local read "Last Edit"() -> (w2456:bool[])
              n1866 = Split 1D Array(array=w2456, index=24) -> (first subarray=w2407:bool[], second subarray=w2408:bool[])
              n1867 = Index Array(array=w2407) -> (element #1=w2406:bool, element #2=w2405:bool, element #3=w2404:bool, element #4=w2403:bool, element #5=w2402:bool, element #6=w2401:bool, element #7=w2400:bool, element #8=w2399:bool, element #9=w2398:bool, element #10=w2397:bool, element #11=w2396:bool, element #12=w2395:bool, element #13=w2394:bool, element #14=w2393:bool, element #15=w2392:bool, element #16=w2391:bool, element #17=w2390:bool, element #18=w2389:bool, element #19=w2388:bool, element #20=w2387:bool, element #21=w2386:bool, element #22=w2385:bool, element #23=w2384:bool, element #24=w2383:bool)  [unwired: 30 in, 6 out]
              n1868 = Split 1D Array(array=w2408, index=30) -> (first subarray=w2409:bool[], second subarray=w2410:bool[])
              n1869 = local write "1 10"(w2406) -> ()
              n1870 = local write "1 7"(w2405) -> ()
              n1871 = local write "1 6"(w2404) -> ()
              n1872 = local write "1 5"(w2403) -> ()
              n1873 = local write "2 10"(w2402) -> ()
              n1874 = local write "2 7"(w2401) -> ()
              n1875 = local write "2 6"(w2400) -> ()
              n1876 = local write "2 5"(w2399) -> ()
              n1877 = local write "3 9"(w2398) -> ()
              n1878 = local write "3 7"(w2397) -> ()
              n1879 = local write "3 6"(w2396) -> ()
              n1880 = local write "3 5"(w2395) -> ()
              n1881 = local write "4 9"(w2394) -> ()
              n1882 = local write "4 7"(w2393) -> ()
              n1883 = local write "4 6"(w2392) -> ()
              n1884 = local write "4 5"(w2391) -> ()
              n1885 = local write "5 8"(w2390) -> ()
              n1886 = local write "5 7"(w2389) -> ()
              n1887 = local write "5 6"(w2388) -> ()
              n1888 = local write "5 5"(w2387) -> ()
              n1889 = local write "6 8"(w2386) -> ()
              n1890 = local write "6 7"(w2385) -> ()
              n1891 = local write "6 6"(w2384) -> ()
              n1892 = local write "6 5"(w2383) -> ()
              n1893 = Index Array(array=w2409) -> (element #1=w2455:bool, element #2=w2454:bool, element #3=w2453:bool, element #4=w2452:bool, element #5=w2451:bool, element #6=w2450:bool, element #7=w2449:bool, element #8=w2448:bool, element #9=w2447:bool, element #10=w2446:bool, element #11=w2445:bool, element #12=w2444:bool, element #13=w2443:bool, element #14=w2442:bool, element #15=w2441:bool, element #16=w2440:bool, element #17=w2439:bool, element #18=w2438:bool, element #19=w2437:bool, element #20=w2436:bool, element #21=w2435:bool, element #22=w2434:bool, element #23=w2433:bool, element #24=w2432:bool, element #25=w2431:bool, element #26=w2430:bool, element #27=w2429:bool, element #28=w2428:bool, element #29=w2427:bool, element #30=w2382:bool)  [unwired: 30 in]
              n1894 = local write "Adrive"(w2455) -> ()
              n1895 = local write "Ddrive"(w2454) -> ()
              n1896 = local write "ASWdrive"(w2453) -> ()
              n1897 = local write "DSWdrive"(w2452) -> ()
              n1898 = local write "Drop 14"(w2451) -> ()
              n1899 = local write "Chop 13"(w2450) -> ()
              n1900 = local write "Lob"(w2449) -> ()
              n1901 = local write "Boast2"(w2448) -> ()
              n1902 = local write "Boast3"(w2447) -> ()
              n1903 = local write "Smash 13"(w2446) -> ()
              n1904 = local write "FH"(w2445) -> ()
              n1905 = local write "BH"(w2444) -> ()
              n1906 = local write "ST"(w2443) -> ()
              n1907 = local write "CR"(w2442) -> ()
              n1908 = local write "Bounce"(w2441) -> ()
              n1909 = local write "Half Volley"(w2440) -> ()
              n1910 = local write "Volley"(w2439) -> ()
              n1911 = local write "Expected Winner1 2"(w2438) -> ()
              n1912 = local write "Expected Winner2 2"(w2437) -> ()
              n1913 = local write "Unexpected Winner1 2"(w2436) -> ()
              n1914 = local write "Unexpected Winner2 2"(w2435) -> ()
              n1915 = local write "Stroke1 2"(w2434) -> ()
              n1916 = local write "Stroke2 2"(w2433) -> ()
              n1917 = local write "Forced Error1 2"(w2432) -> ()
              n1918 = local write "Forced Error2 2"(w2431) -> ()
              n1919 = local write "Unforced Error1 2"(w2430) -> ()
              n1920 = local write "Unforced Error2 2"(w2429) -> ()
              n1921 = local write "Nolet1 2"(w2428) -> ()
              n1922 = local write "Nolet2 2"(w2427) -> ()
              n1923 = local write "Let 2"(w2382) -> ()
              n1924 = local write "Let 5"(w2382) -> ()
              n1925 = Index Array(array=w2410) -> (element #1=w2426:bool, element #2=w2425:bool, element #3=w2424:bool, element #4=w2423:bool, element #5=w2422:bool, element #6=w2421:bool, element #7=w2420:bool, element #8=w2419:bool, element #9=w2418:bool, element #10=w2417:bool, element #11=w2416:bool, element #12=w2415:bool, element #13=w2414:bool, element #14=w2413:bool, element #15=w2412:bool)  [unwired: 15 in]
              n1926 = local write "Service1 2"(w2426) -> ()
              n1927 = local write "Service2 2"(w2425) -> ()
              n1928 = local write "S1 2"(w2424) -> ()
              n1929 = local write "S2 2"(w2423) -> ()
              n1930 = local write "S3 2"(w2422) -> ()
              n1931 = local write "S4 2"(w2421) -> ()
              n1932 = local write "S5 2"(w2420) -> ()
              n1933 = local write "S6 2"(w2419) -> ()
              n1934 = local write "Player1 2"(w2418) -> ()
              n1935 = local write "Player2 2"(w2417) -> ()
              n1936 = local write "Button 6"(w2416) -> ()
              n1937 = local write "Button 7"(w2415) -> ()
              n1938 = local write "Button 8"(w2414) -> ()
              n1939 = local write "Button 9"(w2413) -> ()
              n1940 = local write "Button 10"(w2412) -> ()
            }
          }
          n1941 = local read "Btn 10"() -> (w2254:string)
          n1942 = local read "Btn 7"() -> (w2257:string)
          n1943 = local read "Btn 8"() -> (w2258:string)
          n1944 = local read "Btn 9"() -> (w2255:string)
          n1945 = local read "Btn 6"() -> (w2256:string)
          n1946 = Concatenate Strings(w2256, w2251, w2257, w2251, w2258, w2251, w2255, w2251, w2254, w2251, "Error" ("String")) -> (w2264:string)
          n1947 = for {
            tunnel: string[] ["frame number", "Lead", "Lag", "position 1", "position 2", "position 3", "position 4", "position 5", "position 6", "position 7", "position 8", "position 9", "position 10", "position 11", "position 12", "position 13", "position 14", "position 15", "position 16", "position 17", "position 18", "position 19", "position 20", "position 21", "position 22", "position 23", "position 24", "Drive A", "Drive D", "SW Drive A", "SW Drive D", "drop", "chop", "lob", "boast 2", "boast 3", "smash", "Forehand", "Backhand", "Straight", "Cross", "Bounce", "Half Volley", "Volley", "Expected winner 1", "Expected winner 2", "Unexpected winner 1", "Unexpected winner 2", "Stroke 1", "Stroke 2", "Forced error 1", "Forced error 2", "Unforced error 1", "Unforced error 2", "No let 1", "No let 2", "Let", "point1", "point2", "score1", "score2", "service1", "service2", "s1", "s2", "s3", "s4", "s5", "s6", "player1", "player2"] ("all rows") -> [w2283] mode=indexing
            tunnel: [w2281] -> w2262 mode=indexing
            n1948 = Concatenate Strings(w2283, "\t") -> (w2281:string)
          }
          n1949 = Concatenate Strings(w2262, w2264, "\r") -> (w2259:string)
          n1950 = Array To Spreadsheet String(delimiter (Tab)="\t" ("delimiter (\\t)"), array=w2261, 3:"%.3f" ("format (%.3f)")) -> (spreadsheet string=w2260:string)
          n1951 = local read "Video file"() -> (w2272:path)
          n1952 = local read "Data file"() -> (w2268:path)
          n1953 = call <vilib>:"Get File Extension.vi"("file"=w2272) -> ("filename without extension"=w2274:string)  [unwired: 7 in, 3 out]
          n1954 = Open/Create/Replace File(file path (use dialog)=w2268, operation (0:open)=T3."replace") -> (refnum out=w2270:refnum<file>, error out=w2269:errorcluster)  [unwired: 4 in, 1 out]
          n1955 = Concatenate Strings("avi file" ("string"), w2275, w2274, w2275, w2275, w2259, w2260) -> (w2276:string)
          n1956 = local write "Update"(FALSE ("Update")) -> ()
          n1957 = Write to Text File(file (use dialog)=w2270, text=w2276, error in=w2269) -> (refnum out=w2267:refnum<file>)  [unwired: 1 in, 2 out]
        }
      }
      "refnum of data save file" <- w374
      n1958 = Equal?(x="Main tab", y=enum32{"Coding", "Display"}."Coding" ("Tab Control 3")) -> (x = y?=w384:bool)
      n1959 = Not Equal?(x=w373, y=w379) -> (x != y?=w383:bool)
      n1960 = Select(t=w379, s=w384, f=w381) -> (s? t:f=w372:T1)
      n1961 = And(x=w383, y=w384) -> (x .and. y?=w382:bool)
      n1962 = Equal?(x=w373, y=w379) -> (x = y?=w378:bool)
      n1963 = Equal?(x=w372, y=w381) -> (x = y?=w380:bool)
      n1964 = And(x=w380, y=w378) -> (x .and. y?=w377:bool)
      n1965 = case shown="True" w382 {
        tunnel: w376 -> [_ w393]
        frame False {
        }
        frame True {
          # "Moving back to coding tab"
          n1966 = flat-sequence {
            tunnel: w393 -> [w397]
            frame #0 {
              n1967 = local read "ful video frames"() -> (w398:i64[])
              n1968 = Index Array(array=w397, index (col)=0 ("disabled index (col)")) -> (element=w395:i64[])  [unwired: 1 in]
              n1969 = Array Max & Min(array=w395) -> (max value=w394:i64)  [unwired: 3 out]
              n1970 = local write "frames 2 play"(w398) -> ()
              n1971 = local write "Progress..."(w394) -> ()
            }
            frame #1 {
              w399 = FALSE ("Next")
              w400 = TRUE ("Play")
              n1972 = local write "stop"(w400) -> ()
              n1973 = local write "Load video"(w400) -> ()
              n1974 = local write "Pause"(w399) -> ()
              n1975 = local write "Update"(w399) -> ()
              n1976 = local write "Next"(w399) -> ()
              n1977 = local write "Previous"(w399) -> ()
              n1978 = local write "Reset"(w399) -> ()
              n1979 = local write "Extract data"(w399) -> ()
              n1980 = local write "Upload edited video"(w399) -> ()
              n1981 = local write "Examine code"(w399) -> ()
            }
          }
        }
      }
      n1982 = case shown="True" w377 {
        frame False {
        }
        frame True {
          n1983 = local write "Progress..."(u32 0 ("Progress...")) -> ()
          n1984 = local write "Pause"(FALSE ("Pause")) -> ()
          n1985 = local write "stop"(TRUE ("stop")) -> ()
        }
      }
      n1986 = local read "START"() -> (w375:bool)
      n1987 = Wait (ms)(milliseconds to wait=u32 200) -> ()  [unwired: 1 out]
      "Main tab 2" <- w373
    }
    n1988 = while {
      tunnel: w10 -> [w223]
      tunnel: w1 -> [_]
      tunnel: [w218] -> w5
      stop <- w218 continue-if-true
      # "This loop is for writing\nvideo to disk"
      n1989 = local read "Video files to write"() -> (w222:string[])
      n1990 = local read "frames to write"() -> (w220:i64[][])
      n1991 = case shown="True" "Write file" {
        tunnel: [FALSE FALSE] -> w225
        tunnel: w223 -> [_ w243]
        tunnel: w222 -> [_ w242]
        tunnel: "Video to write" -> [_ w241]
        tunnel: w220 -> [_ w240]
        tunnel: [u32 0 ("milliseconds to wait") u32 0 ("milliseconds to wait")] -> w219
        frame False {
          w227 = T4."Enabled" ("Disabled")
          n1992 = local read "Video files to write"() -> (w231:string[])
          n1993 = property on="Add to lib" class="Bool (strict)"("DisabledEnum"=w227) -> ()  [unwired: 2 in, 2 out]
          n1994 = property on="File name" class="Str"("DisabledEnum"=w227) -> ()  [unwired: 2 in, 2 out]
          n1995 = property on="Video to write" class="Path"("DisabledEnum"=w227) -> ()  [unwired: 2 in, 2 out]
          n1996 = property on="START" class="Bool (strict)"("DisabledEnum"=w227) -> ()  [unwired: 2 in, 2 out]
          n1997 = Empty Array?(array=w231) -> (empty?=w230:bool)
          n1998 = Select(t=T4."Disabled and Grayed Out" ("Disabled"), s=w230, f=w227) -> (s? t:f=w228:T4)
          n1999 = property on="Write file" class="Bool (strict)"("DisabledEnum"=w228) -> ()  [unwired: 2 in, 2 out]
          n2000 = local write "Abort"(FALSE ("Abort")) -> ()
        }
        frame True {
          w235 = T4."Disabled and Grayed Out" ("Disabled")
          n2001 = for {
            tunnel: w240 -> [w282] mode=indexing
            tunnel: w242 -> [w273] mode=indexing
            tunnel: w241 -> [w272]
            tunnel: w243 -> [w260]
            tunnel: [w254] -> w238
            tunnel: [w253] -> w237
            tunnel: [w251] -> w236
            i -> [w255]
            stop <- w252 stop-if-true
            w269 = T5 4 items=["Grayscale (U8)", "Grayscale (I16)", "Grayscale (SGL)", "Complex (CSG)", "RGB (U32)", "HSL (U32)", "RGB (U64)"] ("Image Type")
            n2002 = Path To String(path=w272) -> (string=w274:string)
            n2003 = for {
              tunnel: w282 -> [w320] mode=indexing
              tunnel: [w320] -> w259 mode=indexing if=w319
              n2004 = Not Equal To 0?(x=w320) -> (x != 0?=w319:bool)
            }
            n2005 = Concatenate Strings(w274, "\\" ("string"), w273) -> (w277:string)
            n2006 = Array Size(array=w259) -> (size(s)=w258:i32)
            n2007 = Decrement(x=w255) -> (x-1=w256:i32)
            n2008 = Not Equal To 0?(x=w255) -> (x != 0?=w257:bool)
            n2009 = call <vilib>:"Search and Replace Pattern.vi"("string"=w277, "regular expression (\"\")"=".avi" ("regular expression (\"\")")) -> ("result string"=w281:string)  [unwired: 3 in, 1 out]
            n2010 = case shown="True" w257 {
              tunnel: w256 -> [_ w292]
              frame False {
              }
              frame True {
                n2011 = local read "Video files to write"() -> (w296:string[])
                n2012 = local read "frames to write"() -> (w293:i64[][])
                n2013 = Delete From Array(array=w296, index=w292) -> (array with subset deleted=w295:string[])  [unwired: 1 in, 1 out]
                n2014 = Delete From Array(array=w293, index (row)=w292) -> (array with subset deleted=w294:i64[][])  [unwired: 2 in, 1 out]
                n2015 = local write "frames to write"(w294) -> ()
                n2016 = local write "Video files to write"(w295) -> ()
              }
            }
            n2017 = property on="Writing" class="Slide (strict)"("Scale.Maximum"=w258) -> ()  [unwired: 2 in, 2 out]
            n2018 = Concatenate Strings(w281, ".avi" ("string")) -> (w279:string)
            n2019 = String To Path(string=w279) -> (path=w280:path)
            n2020 = while {
              shift-right: [w300] -> _
              shift-left: w280 -> [w299]
              tunnel: w281 -> [w304]
              tunnel: [w299] -> w250
              i -> [w298]
              stop <- w306 continue-if-true
              n2021 = Increment(x=w298) -> (x+1=w297:i32)
              n2022 = call <vilib>:"Check if File or Folder Exists.vi"("path"=w299) -> ("file or folder exists?"=w306:bool)  [unwired: 8 in, 2 out]
              n2023 = Number To Decimal String(number=w297) -> (decimal integer string=w303:string)  [unwired: 1 in]
              n2024 = Concatenate Strings(w304, " (file path clash) - " ("string"), w303, ".avi" ("string")) -> (w301:string)
              n2025 = String To Path(string=w301) -> (path=w300:path)
            }
            n2026 = Select(t="Microsoft Video 1" ("Codec Name"), s="Video compress", f="" ("Codec Name")) -> (s? t:f=w247:string)
            n2027 = local read "framesPerSecond"() -> (w263:u32)
            n2028 = call "IMAQ AVI Create"("Compression Filter"=w247, "Frames Per Second"=w263, "AVI Path"=w250) -> ("error out"=w270:errorcluster, "Avi Refnum"=w264:T6)  [unwired: 7 in]
            n2029 = call "IMAQ Create"("Image Name"="write", "Image Type"=w269, "error in (no error)"=w270) -> ("New Image"=w268:T2, "error out"=w267:errorcluster)  [unwired: 2 in]
            n2030 = for {
              tunnel: w259 -> [w317] mode=indexing
              tunnel: w268 -> [w311]
              tunnel: w267 -> [w316]
              tunnel: [w314] -> w266
              tunnel: [w313] -> w265
              tunnel: w264 -> [w312]
              tunnel: [w311] -> w261
              tunnel: w260 -> [w310]
              tunnel: ["Abort"] -> w252
              i -> [w309]
              stop <- "Abort" stop-if-true
              n2031 = Increment(x=w309) -> (x+1=→"Writing":i32)
              n2032 = call "IMAQ AVI Read Frame"("error in (no error)"=w316, "Frame Number"=w317, "Image"=w311, "Avi Refnum"=w310) -> ("error out"=w318:errorcluster, "Image Out"=w315:T2)  [unwired: 4 in, 2 out]
              n2033 = call "IMAQ AVI Write Frame"("error in (no error)"=w318, "Image"=w315, "Avi Refnum"=w312) -> ("error out"=w313:errorcluster, "Avi Refnum (duplicate)"=w314:T6)  [unwired: 7 in]
            }
            n2034 = call "IMAQ AVI Close"("error in (no error)"=w265, "Avi Refnum"=w266) -> ("error out"=w262:errorcluster)  [unwired: 9 in]
            n2035 = call "IMAQ Dispose"("Image"=w261, "error in (no error)"=w262) -> ("error out"=w249:errorcluster)  [unwired: 4 in]
            n2036 = case shown="False" w252 {
              tunnel: [string[] [] ("Video files to write") w290] -> w254
              tunnel: [i64[][] [] ("to write") w289] -> w253
              tunnel: ["Writing Complete" ("message") "Writing aborted" ("message")] -> w251
              tunnel: w250 -> [_ w287]
              tunnel: w249 -> [_ w286]
              frame False {
              }
              frame True {
                n2037 = local read "Video files to write"() -> (w290:string[])
                n2038 = Delete(path (use dialog)=w287, error in=w286) -> ()  [unwired: 3 in, 3 out]
                n2039 = local read "frames to write"() -> (w289:i64[][])
                n2040 = local write "Abort"(FALSE ("Abort")) -> ()
              }
            }
          }
          n2041 = One Button Dialog(message=w236) -> ()  [unwired: 1 in, 1 out]
          n2042 = local write "Video files to write"(w238) -> ()
          n2043 = local write "frames to write"(w237) -> ()
          n2044 = property on="Add to lib" class="Bool (strict)"("DisabledEnum"=w235) -> ()  [unwired: 2 in, 2 out]
          n2045 = property on="File name" class="Str"("DisabledEnum"=w235) -> ()  [unwired: 2 in, 2 out]
          n2046 = property on="Video to write" class="Path"("DisabledEnum"=w235) -> ()  [unwired: 2 in, 2 out]
          n2047 = property on="START" class="Bool (strict)"("DisabledEnum"=w235) -> ()  [unwired: 2 in, 2 out]
        }
      }
      n2048 = local read "START"() -> (w218:bool)
      n2049 = local write "Write file"(w225) -> ()
      n2050 = local write "Writing"(w219) -> ()
      n2051 = Wait (ms)(milliseconds to wait=u32 200) -> ()  [unwired: 1 out]
    }
    n2052 = while {
      tunnel: [w184] -> w6
      tunnel: w1 -> [_]
      stop <- w184 continue-if-true
      n2053 = case shown="True" "REPORT" {
        frame False {
        }
        frame True {
          w208 = TRUE ("open new instance (false)")
          n2054 = local read "Data file"() -> (w194:path)
          n2055 = local read "Video file"() -> (w193:path)
          n2056 = local write "REPORT"(FALSE ("REPORT")) -> ()
          n2057 = Strip Path(path=w194) -> (stripped path=w192:path)  [unwired: 1 out]
          n2058 = call <vilib>:"Get File Extension.vi"("file"=w193) -> ("filename without extension"=w189:string)  [unwired: 7 in, 3 out]
          n2059 = Path To String(path=w192) -> (string=w191:string)
          n2060 = Concatenate Strings(w191, "\\" ("string"), w189, " (BStAT Report).doc" ("string")) -> (w195:string)
          n2061 = String To Path(string=w195) -> (path=w197:path)
          n2062 = call <vilib>:"Check if File or Folder Exists.vi"("path"=w197) -> ("file or folder exists?"=w196:bool)  [unwired: 8 in, 2 out]
          n2063 = Automation Open(Automation Refnum=refnum<k7> refnum ("Word._Application"), 9:w208) -> (Automation Refnum=w201:refnum<k7>, error out=w202:errorcluster)  [unwired: 2 in]
          n2064 = property class="_Application"(reference=w201, error in=w202, "Visible"=w208) -> (reference out=w203:refnum<k7>, error out=w204:errorcluster)
          n2065 = case shown="True" w196 {
            tunnel: w197 -> [w211 w217]
            tunnel: [w210 w217] -> w187
            frame False {
              n2066 = Current VI's Path() -> (path=w214:path)
              n2067 = Strip Path(path=w214) -> (stripped path=w213:path)  [unwired: 1 out]
              n2068 = Build Path(base path=w213, name or relative path="BStAT report.doc") -> (appended path=w212:path)
              n2069 = One Button Dialog(message="***New report generated***\n\nRight-click on the white strip on the LEFT of the data area to copy the data ") -> ()  [unwired: 1 in, 1 out]
              n2070 = Copy(10:w211, 11:w212) -> (3:w210:path)  [unwired: 3 in, 2 out]
            }
            frame True {
              n2071 = One Button Dialog(message="***Report found***\n\nRight-click on the white strip on the LEFT of the data area to copy the data ") -> ()  [unwired: 1 in, 1 out]
            }
          }
          n2072 = property class="_Application"(reference=w203, error in=w204) -> (error out=w206:errorcluster, "Documents"=w205:refnum<k7>)  [unwired: 1 out]
          n2073 = invoke class="Documents" method="Open"(reference=w205, error in=w206, "FileName"=w187, "ReadOnly"=TRUE, "Visible"=TRUE) -> ()  [unwired: 14 in, 19 out]
        }
      }
      n2074 = local read "START"() -> (w184:bool)
      n2075 = Wait (ms)(milliseconds to wait=u32 200) -> ()  [unwired: 1 out]
    }
    n2076 = flat-sequence {
      tunnel: w7 -> [w33]
      tunnel: w6 -> [_]
      tunnel: w5 -> [_]
      tunnel: w4 -> [w34]
      frame #0 {
        w28 = T5 4 items=["Grayscale (U8)", "Grayscale (I16)", "Grayscale (SGL)", "Complex (CSG)", "RGB (U32)", "HSL (U32)", "RGB (U64)"] ("Image Type")
        w29 = T5 4 items=["Grayscale (U8)", "Grayscale (I16)", "Grayscale (SGL)", "Complex (CSG)", "RGB (U32)", "HSL (U32)", "RGB (U64)"] ("Image Type")
        w31 = T5 4 items=["Grayscale (U8)", "Grayscale (I16)", "Grayscale (SGL)", "Complex (CSG)", "RGB (U32)", "HSL (U32)", "RGB (U64)"] ("Image Type")
        n2077 = call "IMAQ AVI Close"("Avi Refnum"=w34) -> ("error out"=w32:errorcluster)  [unwired: 10 in]
        n2078 = Close File(refnum=w33, error in=w32) -> (error out=w26:errorcluster)  [unwired: 1 out]
        n2079 = call "IMAQ Create"("Image Name"="Video", "Image Type"=w28, "error in (no error)"=w26) -> ("New Image"=w22:T2, "error out"=w25:errorcluster)  [unwired: 2 in]
        n2080 = call "IMAQ Create"("Image Name"="pauselag", "Image Type"=w31, "error in (no error)"=w25) -> ("New Image"=w21:T2, "error out"=w23:errorcluster)  [unwired: 2 in]
        n2081 = call "IMAQ Create"("Image Name"="write", "Image Type"=w29, "error in (no error)"=w23) -> ("New Image"=w20:T2, "error out"=w19:errorcluster)  [unwired: 2 in]
        n2082 = call "IMAQ Dispose"("Image"=w22, "error in (no error)"=w19) -> ("error out"=w18:errorcluster)  [unwired: 4 in]
        n2083 = call "IMAQ Dispose"("Image"=w21, "error in (no error)"=w18) -> ("error out"=w17:errorcluster)  [unwired: 4 in]
        n2084 = call "IMAQ Dispose"("Image"=w20, "error in (no error)"=w17) -> ()  [unwired: 4 in, 1 out]
      }
    }
    n2085 = Wait (ms)(milliseconds to wait=u32 100) -> ()  [unwired: 1 out]
  }
  n2086 = while {
    stop <- FALSE stop-if-true
    n2087 = case shown="True" "SWDrive" {
      frame True {
        w2576 = TRUE ("Visible")
        w2575 = TRUE ("Visible")
        n2088 = control-ref of="SWDDrive"() -> (w2574:refnum<vi>)
        n2089 = control-ref of="SWDDrive 2"() -> (w2573:refnum<vi>)
        n2090 = control-ref of="SWDDrive 3"() -> (w2572:refnum<vi>)
        n2091 = control-ref of="SWDDrive 4"() -> (w2571:refnum<vi>)
        n2092 = control-ref of="SWDDrive 5"() -> (w2570:refnum<vi>)
        n2093 = control-ref of="SWDDrive 6"() -> (w2569:refnum<vi>)
        n2094 = control-ref of="SWDDrive 7"() -> (w2568:refnum<vi>)
        n2095 = control-ref of="SWDDrive 8"() -> (w2567:refnum<vi>)
        n2096 = control-ref of="SWDDrive 9"() -> (w2566:refnum<vi>)
        n2097 = control-ref of="SWDDrive 10"() -> (w2565:refnum<vi>)
        n2098 = control-ref of="SWDDrive 11"() -> (w2564:refnum<vi>)
        n2099 = control-ref of="SWDDrive 12"() -> (w2563:refnum<vi>)
        n2100 = property class="Bool (strict)"(reference=w2574, "Visible"=w2576) -> (error out=w2550:errorcluster)  [unwired: 1 in, 1 out]
        n2101 = property class="Bool (strict)"(reference=w2573, "Visible"=w2576) -> (error out=w2549:errorcluster)  [unwired: 1 in, 1 out]
        n2102 = property class="Bool (strict)"(reference=w2572, "Visible"=w2576) -> (error out=w2548:errorcluster)  [unwired: 1 in, 1 out]
        n2103 = property class="Bool (strict)"(reference=w2571, "Visible"=w2576) -> (error out=w2547:errorcluster)  [unwired: 1 in, 1 out]
        n2104 = property class="Bool (strict)"(reference=w2570, "Visible"=w2576) -> (error out=w2546:errorcluster)  [unwired: 1 in, 1 out]
        n2105 = property class="Bool (strict)"(reference=w2569, "Visible"=w2576) -> (error out=w2545:errorcluster)  [unwired: 1 in, 1 out]
        n2106 = property class="Bool (strict)"(reference=w2568, "Visible"=w2576) -> (error out=w2544:errorcluster)  [unwired: 1 in, 1 out]
        n2107 = property class="Bool (strict)"(reference=w2567, "Visible"=w2576) -> (error out=w2543:errorcluster)  [unwired: 1 in, 1 out]
        n2108 = property class="Bool (strict)"(reference=w2566, "Visible"=w2576) -> (error out=w2542:errorcluster)  [unwired: 1 in, 1 out]
        n2109 = property class="Bool (strict)"(reference=w2565, "Visible"=w2576) -> (error out=w2541:errorcluster)  [unwired: 1 in, 1 out]
        n2110 = property class="Bool (strict)"(reference=w2564, "Visible"=w2576) -> (error out=w2540:errorcluster)  [unwired: 1 in, 1 out]
        n2111 = property class="Bool (strict)"(reference=w2563, "Visible"=w2576) -> (error out=w2539:errorcluster)  [unwired: 1 in, 1 out]
        n2112 = control-ref of="SWADrive"() -> (w2562:refnum<vi>)
        n2113 = control-ref of="SWADrive 2"() -> (w2561:refnum<vi>)
        n2114 = control-ref of="SWADrive 3"() -> (w2560:refnum<vi>)
        n2115 = control-ref of="SWADrive 4"() -> (w2559:refnum<vi>)
        n2116 = control-ref of="SWADrive 5"() -> (w2558:refnum<vi>)
        n2117 = control-ref of="SWADrive 6"() -> (w2557:refnum<vi>)
        n2118 = control-ref of="SWADrive 7"() -> (w2556:refnum<vi>)
        n2119 = control-ref of="SWADrive 8"() -> (w2555:refnum<vi>)
        n2120 = control-ref of="SWADrive 9"() -> (w2554:refnum<vi>)
        n2121 = control-ref of="SWADrive 10"() -> (w2553:refnum<vi>)
        n2122 = control-ref of="SWADrive 11"() -> (w2552:refnum<vi>)
        n2123 = control-ref of="SWADrive 12"() -> (w2551:refnum<vi>)
        n2124 = property class="Bool (strict)"(reference=w2562, error in=w2550, "Visible"=w2575) -> ()  [unwired: 2 out]
        n2125 = property class="Bool (strict)"(reference=w2561, error in=w2549, "Visible"=w2575) -> ()  [unwired: 2 out]
        n2126 = property class="Bool (strict)"(reference=w2560, error in=w2548, "Visible"=w2575) -> ()  [unwired: 2 out]
        n2127 = property class="Bool (strict)"(reference=w2559, error in=w2547, "Visible"=w2575) -> ()  [unwired: 2 out]
        n2128 = property class="Bool (strict)"(reference=w2558, error in=w2546, "Visible"=w2575) -> ()  [unwired: 2 out]
        n2129 = property class="Bool (strict)"(reference=w2557, error in=w2545, "Visible"=w2575) -> ()  [unwired: 2 out]
        n2130 = property class="Bool (strict)"(reference=w2556, error in=w2544, "Visible"=w2575) -> ()  [unwired: 2 out]
        n2131 = property class="Bool (strict)"(reference=w2555, error in=w2543, "Visible"=w2575) -> ()  [unwired: 2 out]
        n2132 = property class="Bool (strict)"(reference=w2554, error in=w2542, "Visible"=w2575) -> ()  [unwired: 2 out]
        n2133 = property class="Bool (strict)"(reference=w2553, error in=w2541, "Visible"=w2575) -> ()  [unwired: 2 out]
        n2134 = property class="Bool (strict)"(reference=w2552, error in=w2540, "Visible"=w2575) -> ()  [unwired: 2 out]
        n2135 = property class="Bool (strict)"(reference=w2551, error in=w2539, "Visible"=w2575) -> ()  [unwired: 2 out]
      }
      frame False {
        w2614 = FALSE ("Visible")
        w2613 = FALSE ("Visible")
        n2136 = control-ref of="SWDDrive"() -> (w2612:refnum<vi>)
        n2137 = control-ref of="SWDDrive 2"() -> (w2611:refnum<vi>)
        n2138 = control-ref of="SWDDrive 3"() -> (w2610:refnum<vi>)
        n2139 = control-ref of="SWDDrive 4"() -> (w2609:refnum<vi>)
        n2140 = control-ref of="SWDDrive 5"() -> (w2608:refnum<vi>)
        n2141 = control-ref of="SWDDrive 6"() -> (w2607:refnum<vi>)
        n2142 = control-ref of="SWDDrive 7"() -> (w2606:refnum<vi>)
        n2143 = control-ref of="SWDDrive 8"() -> (w2605:refnum<vi>)
        n2144 = control-ref of="SWDDrive 9"() -> (w2604:refnum<vi>)
        n2145 = control-ref of="SWDDrive 10"() -> (w2603:refnum<vi>)
        n2146 = control-ref of="SWDDrive 11"() -> (w2602:refnum<vi>)
        n2147 = control-ref of="SWDDrive 12"() -> (w2601:refnum<vi>)
        n2148 = property class="Bool (strict)"(reference=w2612, "Visible"=w2614) -> (error out=w2588:errorcluster)  [unwired: 1 in, 1 out]
        n2149 = property class="Bool (strict)"(reference=w2611, "Visible"=w2614) -> (error out=w2587:errorcluster)  [unwired: 1 in, 1 out]
        n2150 = property class="Bool (strict)"(reference=w2610, "Visible"=w2614) -> (error out=w2586:errorcluster)  [unwired: 1 in, 1 out]
        n2151 = property class="Bool (strict)"(reference=w2609, "Visible"=w2614) -> (error out=w2585:errorcluster)  [unwired: 1 in, 1 out]
        n2152 = property class="Bool (strict)"(reference=w2608, "Visible"=w2614) -> (error out=w2584:errorcluster)  [unwired: 1 in, 1 out]
        n2153 = property class="Bool (strict)"(reference=w2607, "Visible"=w2614) -> (error out=w2583:errorcluster)  [unwired: 1 in, 1 out]
        n2154 = property class="Bool (strict)"(reference=w2606, "Visible"=w2614) -> (error out=w2582:errorcluster)  [unwired: 1 in, 1 out]
        n2155 = property class="Bool (strict)"(reference=w2605, "Visible"=w2614) -> (error out=w2581:errorcluster)  [unwired: 1 in, 1 out]
        n2156 = property class="Bool (strict)"(reference=w2604, "Visible"=w2614) -> (error out=w2580:errorcluster)  [unwired: 1 in, 1 out]
        n2157 = property class="Bool (strict)"(reference=w2603, "Visible"=w2614) -> (error out=w2579:errorcluster)  [unwired: 1 in, 1 out]
        n2158 = property class="Bool (strict)"(reference=w2602, "Visible"=w2614) -> (error out=w2578:errorcluster)  [unwired: 1 in, 1 out]
        n2159 = property class="Bool (strict)"(reference=w2601, "Visible"=w2614) -> (error out=w2577:errorcluster)  [unwired: 1 in, 1 out]
        n2160 = control-ref of="SWADrive"() -> (w2600:refnum<vi>)
        n2161 = control-ref of="SWADrive 2"() -> (w2599:refnum<vi>)
        n2162 = control-ref of="SWADrive 3"() -> (w2598:refnum<vi>)
        n2163 = control-ref of="SWADrive 4"() -> (w2597:refnum<vi>)
        n2164 = control-ref of="SWADrive 5"() -> (w2596:refnum<vi>)
        n2165 = control-ref of="SWADrive 6"() -> (w2595:refnum<vi>)
        n2166 = control-ref of="SWADrive 7"() -> (w2594:refnum<vi>)
        n2167 = control-ref of="SWADrive 8"() -> (w2593:refnum<vi>)
        n2168 = control-ref of="SWADrive 9"() -> (w2592:refnum<vi>)
        n2169 = control-ref of="SWADrive 10"() -> (w2591:refnum<vi>)
        n2170 = control-ref of="SWADrive 11"() -> (w2590:refnum<vi>)
        n2171 = control-ref of="SWADrive 12"() -> (w2589:refnum<vi>)
        n2172 = property class="Bool (strict)"(reference=w2600, error in=w2588, "Visible"=w2613) -> ()  [unwired: 2 out]
        n2173 = property class="Bool (strict)"(reference=w2599, error in=w2587, "Visible"=w2613) -> ()  [unwired: 2 out]
        n2174 = property class="Bool (strict)"(reference=w2598, error in=w2586, "Visible"=w2613) -> ()  [unwired: 2 out]
        n2175 = property class="Bool (strict)"(reference=w2597, error in=w2585, "Visible"=w2613) -> ()  [unwired: 2 out]
        n2176 = property class="Bool (strict)"(reference=w2596, error in=w2584, "Visible"=w2613) -> ()  [unwired: 2 out]
        n2177 = property class="Bool (strict)"(reference=w2595, error in=w2583, "Visible"=w2613) -> ()  [unwired: 2 out]
        n2178 = property class="Bool (strict)"(reference=w2594, error in=w2582, "Visible"=w2613) -> ()  [unwired: 2 out]
        n2179 = property class="Bool (strict)"(reference=w2593, error in=w2581, "Visible"=w2613) -> ()  [unwired: 2 out]
        n2180 = property class="Bool (strict)"(reference=w2592, error in=w2580, "Visible"=w2613) -> ()  [unwired: 2 out]
        n2181 = property class="Bool (strict)"(reference=w2591, error in=w2579, "Visible"=w2613) -> ()  [unwired: 2 out]
        n2182 = property class="Bool (strict)"(reference=w2590, error in=w2578, "Visible"=w2613) -> ()  [unwired: 2 out]
        n2183 = property class="Bool (strict)"(reference=w2589, error in=w2577, "Visible"=w2613) -> ()  [unwired: 2 out]
      }
    }
    n2184 = case shown="False" "Drive" {
      frame True {
        w2499 = TRUE ("Visible")
        w2500 = TRUE ("Visible")
        n2185 = control-ref of="ADrive"() -> (w2486:refnum<vi>)
        n2186 = control-ref of="ADrive 2"() -> (w2485:refnum<vi>)
        n2187 = control-ref of="ADrive 3"() -> (w2484:refnum<vi>)
        n2188 = control-ref of="ADrive 4"() -> (w2483:refnum<vi>)
        n2189 = control-ref of="ADrive 5"() -> (w2482:refnum<vi>)
        n2190 = control-ref of="ADrive 6"() -> (w2481:refnum<vi>)
        n2191 = control-ref of="ADrive 7"() -> (w2480:refnum<vi>)
        n2192 = control-ref of="ADrive 8"() -> (w2479:refnum<vi>)
        n2193 = control-ref of="ADrive 9"() -> (w2478:refnum<vi>)
        n2194 = control-ref of="ADrive 10"() -> (w2477:refnum<vi>)
        n2195 = control-ref of="ADrive 11"() -> (w2476:refnum<vi>)
        n2196 = control-ref of="ADrive 12"() -> (w2475:refnum<vi>)
        n2197 = property class="Bool (strict)"(reference=w2486, "Visible"=w2500) -> (error out=w2474:errorcluster)  [unwired: 1 in, 1 out]
        n2198 = property class="Bool (strict)"(reference=w2485, "Visible"=w2500) -> (error out=w2473:errorcluster)  [unwired: 1 in, 1 out]
        n2199 = property class="Bool (strict)"(reference=w2484, "Visible"=w2500) -> (error out=w2472:errorcluster)  [unwired: 1 in, 1 out]
        n2200 = property class="Bool (strict)"(reference=w2483, "Visible"=w2500) -> (error out=w2471:errorcluster)  [unwired: 1 in, 1 out]
        n2201 = property class="Bool (strict)"(reference=w2482, "Visible"=w2500) -> (error out=w2470:errorcluster)  [unwired: 1 in, 1 out]
        n2202 = property class="Bool (strict)"(reference=w2481, "Visible"=w2500) -> (error out=w2469:errorcluster)  [unwired: 1 in, 1 out]
        n2203 = property class="Bool (strict)"(reference=w2480, "Visible"=w2500) -> (error out=w2468:errorcluster)  [unwired: 1 in, 1 out]
        n2204 = property class="Bool (strict)"(reference=w2479, "Visible"=w2500) -> (error out=w2467:errorcluster)  [unwired: 1 in, 1 out]
        n2205 = property class="Bool (strict)"(reference=w2478, "Visible"=w2500) -> (error out=w2466:errorcluster)  [unwired: 1 in, 1 out]
        n2206 = property class="Bool (strict)"(reference=w2477, "Visible"=w2500) -> (error out=w2465:errorcluster)  [unwired: 1 in, 1 out]
        n2207 = property class="Bool (strict)"(reference=w2476, "Visible"=w2500) -> (error out=w2464:errorcluster)  [unwired: 1 in, 1 out]
        n2208 = property class="Bool (strict)"(reference=w2475, "Visible"=w2500) -> (error out=w2463:errorcluster)  [unwired: 1 in, 1 out]
        n2209 = control-ref of="DDrive"() -> (w2498:refnum<vi>)
        n2210 = control-ref of="DDrive 2"() -> (w2497:refnum<vi>)
        n2211 = control-ref of="DDrive 3"() -> (w2496:refnum<vi>)
        n2212 = control-ref of="DDrive 4"() -> (w2495:refnum<vi>)
        n2213 = control-ref of="DDrive 5"() -> (w2494:refnum<vi>)
        n2214 = control-ref of="DDrive 6"() -> (w2493:refnum<vi>)
        n2215 = control-ref of="DDrive 7"() -> (w2492:refnum<vi>)
        n2216 = control-ref of="DDrive 8"() -> (w2491:refnum<vi>)
        n2217 = control-ref of="DDrive 9"() -> (w2490:refnum<vi>)
        n2218 = control-ref of="DDrive 10"() -> (w2489:refnum<vi>)
        n2219 = control-ref of="DDrive 11"() -> (w2488:refnum<vi>)
        n2220 = control-ref of="DDrive 12"() -> (w2487:refnum<vi>)
        n2221 = property class="Bool (strict)"(reference=w2498, error in=w2474, "Visible"=w2499) -> ()  [unwired: 2 out]
        n2222 = property class="Bool (strict)"(reference=w2497, error in=w2473, "Visible"=w2499) -> ()  [unwired: 2 out]
        n2223 = property class="Bool (strict)"(reference=w2496, error in=w2472, "Visible"=w2499) -> ()  [unwired: 2 out]
        n2224 = property class="Bool (strict)"(reference=w2495, error in=w2471, "Visible"=w2499) -> ()  [unwired: 2 out]
        n2225 = property class="Bool (strict)"(reference=w2494, error in=w2470, "Visible"=w2499) -> ()  [unwired: 2 out]
        n2226 = property class="Bool (strict)"(reference=w2493, error in=w2469, "Visible"=w2499) -> ()  [unwired: 2 out]
        n2227 = property class="Bool (strict)"(reference=w2492, error in=w2468, "Visible"=w2499) -> ()  [unwired: 2 out]
        n2228 = property class="Bool (strict)"(reference=w2491, error in=w2467, "Visible"=w2499) -> ()  [unwired: 2 out]
        n2229 = property class="Bool (strict)"(reference=w2490, error in=w2466, "Visible"=w2499) -> ()  [unwired: 2 out]
        n2230 = property class="Bool (strict)"(reference=w2489, error in=w2465, "Visible"=w2499) -> ()  [unwired: 2 out]
        n2231 = property class="Bool (strict)"(reference=w2488, error in=w2464, "Visible"=w2499) -> ()  [unwired: 2 out]
        n2232 = property class="Bool (strict)"(reference=w2487, error in=w2463, "Visible"=w2499) -> ()  [unwired: 2 out]
      }
      frame False {
        w2537 = FALSE ("Visible")
        w2538 = FALSE ("Visible")
        n2233 = control-ref of="ADrive"() -> (w2524:refnum<vi>)
        n2234 = control-ref of="ADrive 2"() -> (w2523:refnum<vi>)
        n2235 = control-ref of="ADrive 3"() -> (w2522:refnum<vi>)
        n2236 = control-ref of="ADrive 4"() -> (w2521:refnum<vi>)
        n2237 = control-ref of="ADrive 5"() -> (w2520:refnum<vi>)
        n2238 = control-ref of="ADrive 6"() -> (w2519:refnum<vi>)
        n2239 = control-ref of="ADrive 7"() -> (w2518:refnum<vi>)
        n2240 = control-ref of="ADrive 8"() -> (w2517:refnum<vi>)
        n2241 = control-ref of="ADrive 9"() -> (w2516:refnum<vi>)
        n2242 = control-ref of="ADrive 10"() -> (w2515:refnum<vi>)
        n2243 = control-ref of="ADrive 11"() -> (w2514:refnum<vi>)
        n2244 = control-ref of="ADrive 12"() -> (w2513:refnum<vi>)
        n2245 = property class="Bool (strict)"(reference=w2524, "Visible"=w2538) -> (error out=w2512:errorcluster)  [unwired: 1 in, 1 out]
        n2246 = property class="Bool (strict)"(reference=w2523, "Visible"=w2538) -> (error out=w2511:errorcluster)  [unwired: 1 in, 1 out]
        n2247 = property class="Bool (strict)"(reference=w2522, "Visible"=w2538) -> (error out=w2510:errorcluster)  [unwired: 1 in, 1 out]
        n2248 = property class="Bool (strict)"(reference=w2521, "Visible"=w2538) -> (error out=w2509:errorcluster)  [unwired: 1 in, 1 out]
        n2249 = property class="Bool (strict)"(reference=w2520, "Visible"=w2538) -> (error out=w2508:errorcluster)  [unwired: 1 in, 1 out]
        n2250 = property class="Bool (strict)"(reference=w2519, "Visible"=w2538) -> (error out=w2507:errorcluster)  [unwired: 1 in, 1 out]
        n2251 = property class="Bool (strict)"(reference=w2518, "Visible"=w2538) -> (error out=w2506:errorcluster)  [unwired: 1 in, 1 out]
        n2252 = property class="Bool (strict)"(reference=w2517, "Visible"=w2538) -> (error out=w2505:errorcluster)  [unwired: 1 in, 1 out]
        n2253 = property class="Bool (strict)"(reference=w2516, "Visible"=w2538) -> (error out=w2504:errorcluster)  [unwired: 1 in, 1 out]
        n2254 = property class="Bool (strict)"(reference=w2515, "Visible"=w2538) -> (error out=w2503:errorcluster)  [unwired: 1 in, 1 out]
        n2255 = property class="Bool (strict)"(reference=w2514, "Visible"=w2538) -> (error out=w2502:errorcluster)  [unwired: 1 in, 1 out]
        n2256 = property class="Bool (strict)"(reference=w2513, "Visible"=w2538) -> (error out=w2501:errorcluster)  [unwired: 1 in, 1 out]
        n2257 = control-ref of="DDrive"() -> (w2536:refnum<vi>)
        n2258 = control-ref of="DDrive 2"() -> (w2535:refnum<vi>)
        n2259 = control-ref of="DDrive 3"() -> (w2534:refnum<vi>)
        n2260 = control-ref of="DDrive 4"() -> (w2533:refnum<vi>)
        n2261 = control-ref of="DDrive 5"() -> (w2532:refnum<vi>)
        n2262 = control-ref of="DDrive 6"() -> (w2531:refnum<vi>)
        n2263 = control-ref of="DDrive 7"() -> (w2530:refnum<vi>)
        n2264 = control-ref of="DDrive 8"() -> (w2529:refnum<vi>)
        n2265 = control-ref of="DDrive 9"() -> (w2528:refnum<vi>)
        n2266 = control-ref of="DDrive 10"() -> (w2527:refnum<vi>)
        n2267 = control-ref of="DDrive 11"() -> (w2526:refnum<vi>)
        n2268 = control-ref of="DDrive 12"() -> (w2525:refnum<vi>)
        n2269 = property class="Bool (strict)"(reference=w2536, error in=w2512, "Visible"=w2537) -> ()  [unwired: 2 out]
        n2270 = property class="Bool (strict)"(reference=w2535, error in=w2511, "Visible"=w2537) -> ()  [unwired: 2 out]
        n2271 = property class="Bool (strict)"(reference=w2534, error in=w2510, "Visible"=w2537) -> ()  [unwired: 2 out]
        n2272 = property class="Bool (strict)"(reference=w2533, error in=w2509, "Visible"=w2537) -> ()  [unwired: 2 out]
        n2273 = property class="Bool (strict)"(reference=w2532, error in=w2508, "Visible"=w2537) -> ()  [unwired: 2 out]
        n2274 = property class="Bool (strict)"(reference=w2531, error in=w2507, "Visible"=w2537) -> ()  [unwired: 2 out]
        n2275 = property class="Bool (strict)"(reference=w2530, error in=w2506, "Visible"=w2537) -> ()  [unwired: 2 out]
        n2276 = property class="Bool (strict)"(reference=w2529, error in=w2505, "Visible"=w2537) -> ()  [unwired: 2 out]
        n2277 = property class="Bool (strict)"(reference=w2528, error in=w2504, "Visible"=w2537) -> ()  [unwired: 2 out]
        n2278 = property class="Bool (strict)"(reference=w2527, error in=w2503, "Visible"=w2537) -> ()  [unwired: 2 out]
        n2279 = property class="Bool (strict)"(reference=w2526, error in=w2502, "Visible"=w2537) -> ()  [unwired: 2 out]
        n2280 = property class="Bool (strict)"(reference=w2525, error in=w2501, "Visible"=w2537) -> ()  [unwired: 2 out]
      }
    }
    n2281 = event shown="[2] Key Down" {
      selector: _ -> [_ _ _]
      dyn-events: _ -> [_ _ _]
      timeout: 100 -> [_ _ _]
      event Timeout {
        n2282 = event-data() -> ()  [unwired: 1 in, 3 out]
        n2283 = local write "fast forward"(FALSE ("fast forward")) -> ()
        n2284 = local write "fast rewind"(FALSE ("fast rewind")) -> ()
      }
      event Key Repeat {
        n2285 = event-data() -> ("VKey"=w2617:T8)  [unwired: 1 in, 9 out]
        n2286 = case shown="\"Right\"" w2617 {
          frame "ASCII", Default {
          }
          frame "Enter" {
          }
          frame "Return" {
          }
          frame "Shift" {
          }
          frame "Ctrl" {
          }
          frame "Alt" {
          }
          frame "Cmd" {
          }
          frame "Opt" {
          }
          frame "Caps" {
          }
          frame "NumLock" {
          }
          frame "Clear" {
          }
          frame "Break" {
          }
          frame "Up" {
          }
          frame "Down" {
          }
          frame "Left" {
            n2287 = local write "fast rewind"(TRUE ("fast rewind")) -> ()
          }
          frame "Right" {
            n2288 = local write "fast forward"(TRUE ("fast forward")) -> ()
          }
          frame "Insert" {
          }
          frame "Delete" {
          }
          frame "Home" {
          }
          frame "End" {
          }
          frame "PageUp" {
          }
          frame "PageDown" {
          }
          frame "Escape" {
          }
          frame "Help" {
          }
          frame "Pause" {
          }
          frame "ScrollLock" {
          }
          frame "F1" {
          }
          frame "F2" {
          }
          frame "F3" {
          }
          frame "F4" {
          }
          frame "F5" {
          }
          frame "F6" {
          }
          frame "F7" {
          }
          frame "F8" {
          }
          frame "F9" {
          }
          frame "F10" {
          }
          frame "F11" {
          }
          frame "F12" {
          }
          frame "F13" {
          }
          frame "F14" {
          }
          frame "F15" {
          }
          frame "F16" {
          }
          frame "F17" {
          }
          frame "F18" {
          }
          frame "F19" {
          }
          frame "F20" {
          }
          frame "F21" {
          }
          frame "F22" {
          }
          frame "F23" {
          }
          frame "F24" {
          }
          frame "Play" {
          }
          frame "VolumeUp" {
          }
          frame "VolumeDown" {
          }
          frame "Mute" {
          }
          frame "Two Byte Char" {
          }
        }
      }
      event Key Down {
        n2289 = event-data() -> ("Char"=w2631:i16, "VKey"=w2620:T8)  [unwired: 1 in, 8 out]
        n2290 = property on="Btn 2" class="Str"() -> ("Key Focus"=w2626:bool)  [unwired: 2 in, 2 out]
        n2291 = property on="Btn 3" class="Str"() -> ("Key Focus"=w2625:bool)  [unwired: 2 in, 2 out]
        n2292 = property on="Btn 4" class="Str"() -> ("Key Focus"=w2624:bool)  [unwired: 2 in, 2 out]
        n2293 = property on="Btn 5" class="Str"() -> ("Key Focus"=w2627:bool)  [unwired: 2 in, 2 out]
        n2294 = property on="Btn 1" class="Str"() -> ("Key Focus"=w2628:bool)  [unwired: 2 in, 2 out]
        n2295 = Equal?(x=i16 32, y=w2631) -> (x = y?=w2622:bool)
        n2296 = Compound Arithmetic op=OR(w2626, w2625, w2624, w2627, w2628) -> (w2629:bool)
        n2297 = Not(x=w2629) -> (.not. x?=w2623:bool)
        n2298 = And(x=w2622, y=w2623) -> (x .and. y?=w2621:bool)
        n2299 = case shown="\"Escape\"" w2620 {
          frame "ASCII", Default {
          }
          frame "Enter" {
          }
          frame "Return" {
          }
          frame "Shift" {
          }
          frame "Ctrl" {
          }
          frame "Alt" {
          }
          frame "Cmd" {
          }
          frame "Opt" {
          }
          frame "Caps" {
          }
          frame "NumLock" {
          }
          frame "Clear" {
          }
          frame "Break" {
          }
          frame "Up" {
          }
          frame "Down" {
          }
          frame "Left" {
          }
          frame "Right" {
          }
          frame "Insert" {
          }
          frame "Delete" {
          }
          frame "Home" {
          }
          frame "End" {
          }
          frame "PageUp" {
          }
          frame "PageDown" {
          }
          frame "Escape" {
            n2300 = local write "Undo"(TRUE ("Undo")) -> ()
          }
          frame "Help" {
          }
          frame "Pause" {
          }
          frame "ScrollLock" {
          }
          frame "F1" {
          }
          frame "F2" {
          }
          frame "F3" {
          }
          frame "F4" {
          }
          frame "F5" {
          }
          frame "F6" {
          }
          frame "F7" {
          }
          frame "F8" {
          }
          frame "F9" {
          }
          frame "F10" {
          }
          frame "F11" {
          }
          frame "F12" {
          }
          frame "F13" {
          }
          frame "F14" {
          }
          frame "F15" {
          }
          frame "F16" {
          }
          frame "F17" {
          }
          frame "F18" {
          }
          frame "F19" {
          }
          frame "F20" {
          }
          frame "F21" {
          }
          frame "F22" {
          }
          frame "F23" {
          }
          frame "F24" {
          }
          frame "Play" {
          }
          frame "VolumeUp" {
          }
          frame "VolumeDown" {
          }
          frame "Mute" {
          }
          frame "Two Byte Char" {
          }
        }
        n2301 = case shown="True" w2621 {
          frame False {
          }
          frame True {
            n2302 = local read "Pause"() -> (w2634:bool)
            n2303 = Not(x=w2634) -> (.not. x?=w2633:bool)
            n2304 = local write "Pause"(w2633) -> ()
          }
        }
      }
    }
  }
